vi "Omniax_MotorDrive_XYZR_LOOP_V.vi"() -> ()   [LabVIEW 2009]
uses:
  <vilib>/Utility/file.llb/Read From Spreadsheet File (DBL).vi
  <vilib>/Utility/file.llb/Read From Spreadsheet File (string).vi
  <vilib>/Instr/_visa.llb/VISA Configure Serial Port (Instr).vi
  <vilib>/Utility/file.llb/Write To Spreadsheet File (string).vi
  <vilib>/Utility/file.llb/Write To Spreadsheet File (DBL).vi
panel:
  out "NewLoop":bool
  out "LoopCheck":bool
  out "Only GO":bool
  in  "Loop Scan":bool
  out "FirstScan":bool
  out "Z Moved":bool
  out "GOBACK":bool
  out "LoopScanConfirmed":bool
  out "counter":i32
  out "OP":bool
  out "CL":bool
  out "Valve \nopend/closed":bool
  in  "OK Button":bool
  out "STATUS":string
  in  "Delete Button":bool
  in  "String":string
  in  "Add Button":bool
  in  "Set Button":bool
  in  "Preset positions":i32(ring) items=["ZERO", "Default", "CDOSE", "QMS", "test", "test2", "test3"]
  out "Presets":i32[][](array[numeric])
  out "X MINPOS":i32=-94296
  out "X MAXPOS":i32=-34296
  out "Y MINPOS":i32=-94296
  out "Y MAXPOS":i32=-34296
  out "R MAXPOS":i32=-34296
  out "R MINPOS":i32=-94296
  out "Z MINPOS":i32=-94296
  out "Z MAXPOS":i32=-34296
  in  "HARDSTOP":bool
  in  "GO":bool
  out "XYZR VEL PV Array":i32[](array[numeric])
  out "XYZ in RANGE Array":bool[](array[boolean])
  out "STEP SP Array":i32[](array[numeric])
  out "RUNHOLDArray":i32[](array[numeric])
  out "ZCONSTArray":dbl[](array[numeric])
  out "RCONSTArray":dbl[](array[numeric])
  out "XCONSTArray":dbl[](array[numeric])
  out "YCONSTArray":dbl[](array[numeric])
  out "Error Array":errorcluster[](array[cluster])
  out "COM PORT Array":refnum<visa-resource-name>[](array[refnum])
  out "Z COM PORT":refnum<visa-resource-name>="COM6"
  in  "Tab Control 3":enum32{"Status", "Reset"}(tab)
  out "Y in Range":bool
  out "Y Scan":bool
  out "Y in Motion":bool
  out "Y Backlash corr":bool
  out "X  in Range":bool
  out "X Scan":bool
  out "X  in Motion":bool
  out "X Backlash corr":bool
  out "Z in Range":bool
  out "Z Scan":bool
  out "Z in Motion":bool
  out "Z Backlash corr":bool
  out "R in Range":bool
  out "R Scan":bool
  out "R in Motion":bool
  out "R Backlash corr":bool
  out "X Ready":bool
  out "Y Ready":bool
  out "Z Ready":bool
  out "R Ready":bool
  in  "Reset Y Position mm":dbl
  out "Reset Y Motor Steps":i32
  in  "Reset X Position mm":dbl
  out "Reset X Motor Steps":i32
  in  "Reset Z Position mm":dbl
  out "Reset Z Motor Steps":i32
  in  "Reset R Position deg":dbl
  out "Reset R Motor Steps":i32
  in  "Reset":bool
  in  "Tab Control 2":enum32{"mm", "step"}(tab)
  in  "X Scan Length SP mm":dbl
  in  "X Scan Velocity SP mm/sec":dbl
  in  "Y Scan Length SP mm":dbl
  in  "Y Scan Velocity SP mm/sec":dbl
  in  "Set Scan \nParameters":bool
  in  "Z Scan Length SP mm":dbl
  in  "Z Scan Velocity SP mm/sec":dbl
  in  "R Scan Length SP deg":dbl
  in  "R Scan Velocity SP deg/sec":dbl
  in  "Z as dominating length":bool
  in  "Nr LOOPS":i32
  in  "X Scan Velocity SP steps/sec":i32=1 min=1 max=102400 step=1
  in  "X Scan Length SP steps":i32 min=-2304000 max=2304000 step=100
  out "X Scan length MV mm":dbl
  out "X Scan velocity MV mm/sec":dbl format="%#_6f"
  in  "Y Scan Velocity SP steps/sec":i32=1 min=1 max=102400 step=1
  in  "Y Scan Length SP steps":i32 min=-2560000 max=2048000 step=100
  out "Y Scan length MV mm":dbl
  out "Y Scan velocity MV mm/sec":dbl format="%#_6f"
  in  "Z Scan Velocity SP steps/sec":i32=1 min=1 max=102400 step=1
  in  "Z Scan Length SP steps":i32 min=-11520000 max=90880000 step=100
  out "Z Scan length MV mm":dbl
  out "Z Scan velocity MV mm/sec":dbl format="%#_6f"
  in  "R Scan Velocity SP steps/sec":i32=1 min=1 max=102400 step=1
  in  "R Scan Length SP steps":i32 min=-1501867 max=4642133 step=100
  out "R Scan length MV deg":dbl
  out "R Scan velocity MV deg/sec":dbl format="%#_6f"
  out "atan Y/Z":dbl
  in  "Tab Control":enum32{"mm", "step"}(tab)
  in  "X Position SP mm":dbl
  in  "X Velocity SP mm/sec":dbl
  in  "X Move Set":bool
  in  "Y Move Set":bool
  in  "Y Position SP mm":dbl
  in  "Y Velocity SP mm/sec":dbl
  in  "Z Position SP mm":dbl
  in  "Z Velocity SP mm/sec":dbl
  in  "Z Move Set":bool
  in  "R Position SP deg":dbl
  in  "R Velocity SP deg/sec":dbl
  in  "R Move Set":bool
  in  "X Velocity SP step/sec":i32 min=1 max=128000
  out "X Velocity MV mm/sec":dbl
  in  "Y Velocity SP step/sec":i32 min=1 max=128000
  out "Y Velocity MV mm/sec":dbl
  in  "Z Velocity SP step/sec":i32 min=1 max=204800
  out "Z Velocity MV mm/sec":dbl
  in  "R Velocity SP step/sec":i32 min=1 max=20000
  out "R Velocity MVdeg/sec":dbl
  in  "Y Step SP":i32=-20000 min=-2304000 max=2304000 step=500
  out "Y Position MV mm":dbl
  in  "X Step SP":i32=-20000 min=-2304000 max=2304000 step=500
  out "X Position MV mm":dbl
  in  "Z Step SP":i32=-20000 min=0 max=102400000 step=500
  out "Z Position MV mm":dbl
  in  "R Step SP":i32=-20000 min=-6144000 max=0 step=500
  out "R Position MV deg":dbl
  out "X Step PV":i32 max=2000
  out "Y Step PV":i32 max=2000
  out "Z Step PV":i32 max=2000
  out "R Step PV":i32 max=2000
  in  "Clear ZY":bool
  out "ZY Graph":cluster{dbl[], dbl[]}(graph)
  out "ZR Graph":cluster{"Y":dbl[], "Y":dbl[]}[](graph)
  out "XY Graph":cluster{"Y":dbl[], "Y":dbl[]}[](graph)
  out "X Scan Duration":dbl
  out "Y Scan Duration":dbl
  out "Z Scan Duration":dbl
  out "R Scan Duration":dbl
  out "R Backlash steps/sec":i32
  out "R Backlash":i32
  out "R Holding Current %":i32
  out "R Run Current %":i32
  out "R offset deg":dbl
  out "R deg/rev":dbl
  out "R steps/rev":u32
  out "R velocity PV step/sec":i32
  out "R COM PORT":refnum<visa-resource-name>="COM5"
  out "R Position deg PV":dbl
  out "Z Backlash steps/sec":i32
  out "Z Backlash":i32
  out "Z Holding Current %":i32
  out "Z Run Current %":i32
  out "Z offset mm":dbl
  out "Z mm/rev":dbl
  out "Z steps/rev":u32
  out "Z  velocity PV step/sec":i32
  out "Z Position mm PV":dbl
  out "X Position mm PV":dbl
  out "X velocity PV step/sec":i32
  in  "Set for Scan":bool
  out "X Backlash steps/sec":i32
  out "X Backlash":i32
  out "X Holding Current %":i32
  out "X Run Current %":i32
  out "X offset mm":dbl
  out "X mm/rev":dbl
  out "X steps/rev":u32
  out "X COM PORT":refnum<visa-resource-name>="COM5"
  out "Y Backlash steps/sec":i32
  out "Y Backlash":i32
  out "Y Holding Current %":i32
  out "Y Run Current %":i32
  in  "Scan Cancel":bool
  out "Y Position mm PV":dbl
  out "Y offset mm":dbl
  out "Y mm/rev":dbl
  out "Y steps/rev":u32
  out "Y velocity PV step/sec":i32
  in  "Scan Go":bool
  in  "Stop":bool
  out "Y COM PORT":refnum<visa-resource-name>="COM5"
  # "MX"
  # "MY"
  # "MZ"
  # "MR"
  # "Indicators"
  # "L"
  # "M"
  # "B"
  # "S"
  # "R"
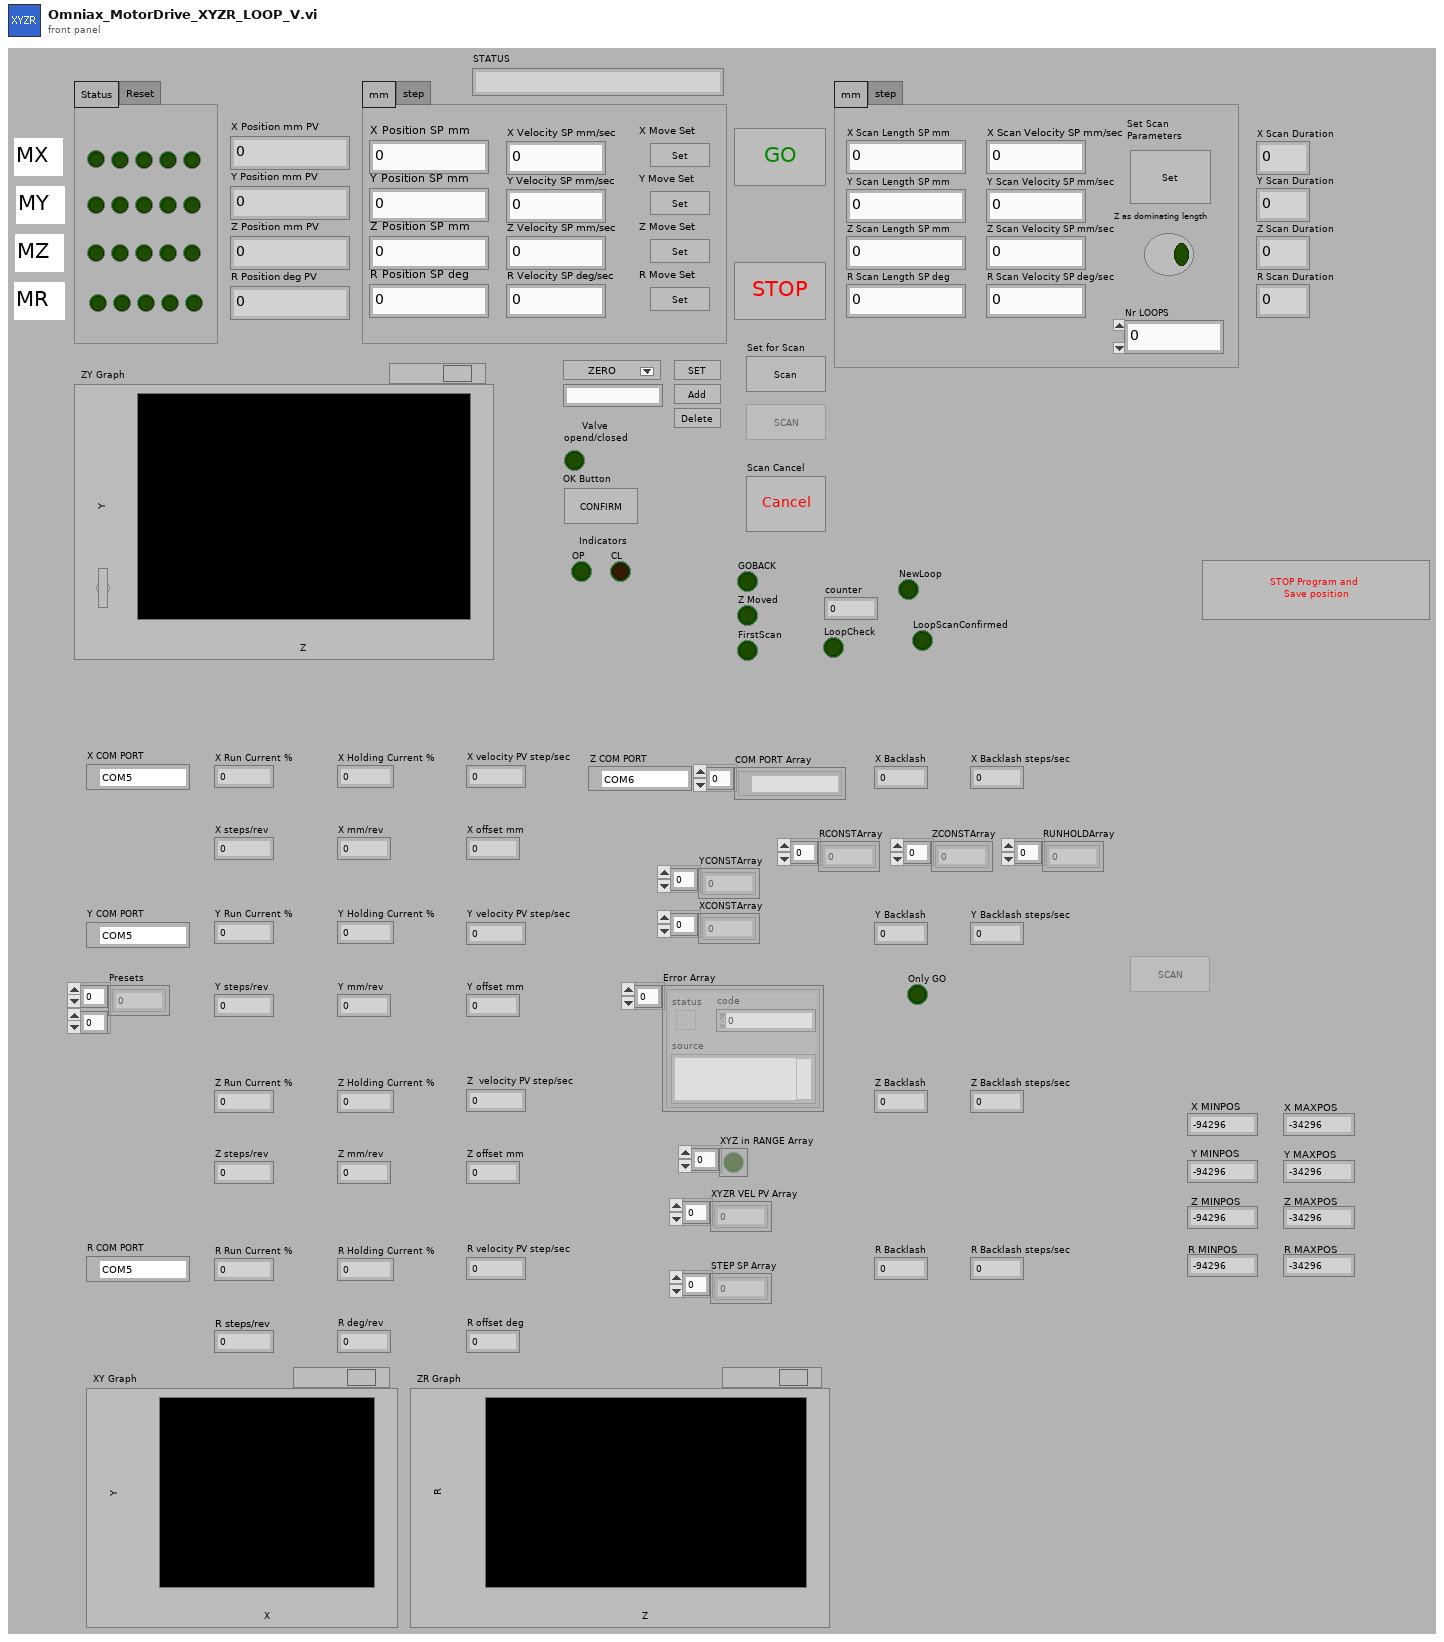
[diagram p1: front panel]
types:
  T1 = enum8{"Enabled", "Disabled", "Disabled and Grayed Out"}
  T2 = cluster{"[0]":i32, "[1]":i32, "[2]":i32, "[3]":i32, "[4]":i32, "[5]":i32, "[6]":i32, "[7]":i32, "[8]":i32}
  T3 = cluster{"XY Max Min array OUT[0]":dbl, "XY Max Min array OUT[1]":dbl, "XY Max Min array OUT[2]":dbl, "XY Max Min array OUT[3]":dbl, "XY Max Min array OUT[4]":dbl, "XY Max Min array OUT[5]":dbl, "XY Max Min array OUT[6]":dbl, "XY Max Min array OUT[7]":dbl, "XY Max Min array OUT[8]":dbl}
  T4 = cluster{"COM PORT Array OUT[0]":refnum<visa-resource-name>, "COM PORT Array OUT[1]":refnum<visa-resource-name>, "COM PORT Array OUT[2]":refnum<visa-resource-name>, "COM PORT Array OUT[3]":refnum<visa-resource-name>, "COM PORT Array OUT[4]":refnum<visa-resource-name>, "COM PORT Array OUT[5]":refnum<visa-resource-name>, "COM PORT Array OUT[6]":refnum<visa-resource-name>, "COM PORT Array OUT[7]":refnum<visa-resource-name>, "COM PORT Array OUT[8]":refnum<visa-resource-name>}
  T5 = cluster{"STEP SP Array OUT[0]":i32, "STEP SP Array OUT[1]":i32, "STEP SP Array OUT[2]":i32, "STEP SP Array OUT[3]":i32, "STEP SP Array OUT[4]":i32, "STEP SP Array OUT[5]":i32, "STEP SP Array OUT[6]":i32, "STEP SP Array OUT[7]":i32, "STEP SP Array OUT[8]":i32}
  T6 = cluster{"XYZ in RANGE Array OUT[0]":bool, "XYZ in RANGE Array OUT[1]":bool, "XYZ in RANGE Array OUT[2]":bool, "XYZ in RANGE Array OUT[3]":bool, "XYZ in RANGE Array OUT[4]":bool, "XYZ in RANGE Array OUT[5]":bool, "XYZ in RANGE Array OUT[6]":bool, "XYZ in RANGE Array OUT[7]":bool, "XYZ in RANGE Array OUT[8]":bool}
  T7 = cluster{"XYZR VEL PV Array OUT[0]":i32, "XYZR VEL PV Array OUT[1]":i32, "XYZR VEL PV Array OUT[2]":i32, "XYZR VEL PV Array OUT[3]":i32, "XYZR VEL PV Array OUT[4]":i32, "XYZR VEL PV Array OUT[5]":i32, "XYZR VEL PV Array OUT[6]":i32, "XYZR VEL PV Array OUT[7]":i32, "XYZR VEL PV Array OUT[8]":i32}
  T8 = cluster{"XYZR MAX MIN POS[0]":i32, "XYZR MAX MIN POS[1]":i32, "XYZR MAX MIN POS[2]":i32, "XYZR MAX MIN POS[3]":i32, "XYZR MAX MIN POS[4]":i32, "XYZR MAX MIN POS[5]":i32, "XYZR MAX MIN POS[6]":i32, "XYZR MAX MIN POS[7]":i32, "XYZR MAX MIN POS[8]":i32}
  T9 = cluster{"Error Array OUT[0]":errorcluster, "Error Array OUT[1]":errorcluster, "Error Array OUT[2]":errorcluster, "Error Array OUT[3]":errorcluster, "Error Array OUT[4]":errorcluster, "Error Array OUT[5]":errorcluster, "Error Array OUT[6]":errorcluster, "Error Array OUT[7]":errorcluster, "Error Array OUT[8]":errorcluster}
  T10 = enum16{"Stop", "Reset", "Run Current", "Holding Current", "Accel Rate", "Decel Rate", "Move to Relative Position", "Move to Absolute Position", "Echo Mode", "Print Parameter", "Send String", "Microstep Resolution", "Set Current Position", "Max Velocity"}
  T11 = cluster{"Presets[0]":i32, "Presets[1]":i32, "Presets[2]":i32, "Presets[3]":i32, "Presets[4]":i32, "Presets[5]":i32, "Presets[6]":i32, "Presets[7]":i32, "Presets[8]":i32}
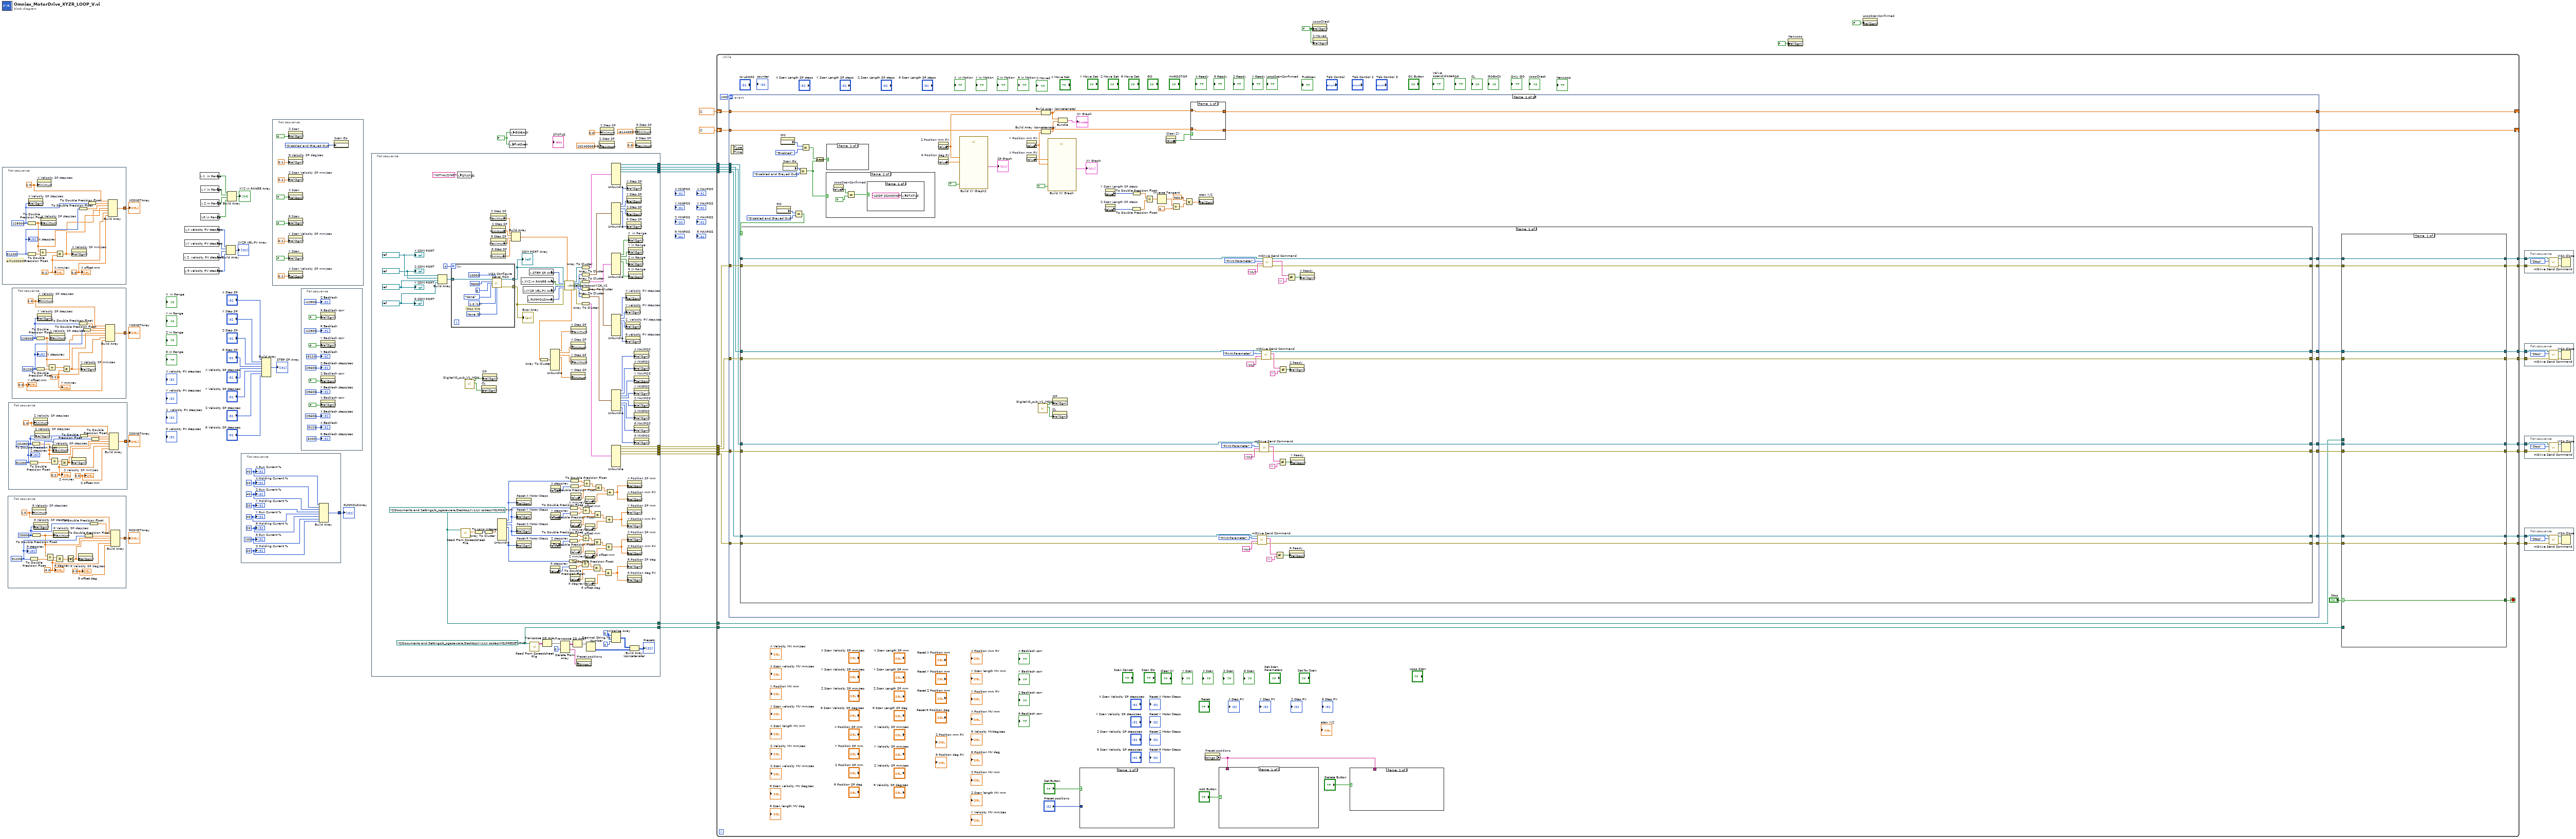
[diagram p0: block diagram]
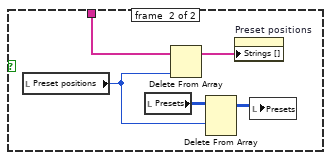
[diagram p2: hidden frame]
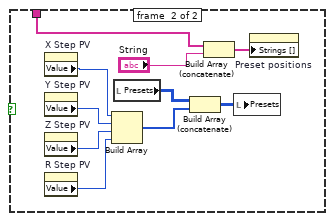
[diagram p3: hidden frame]
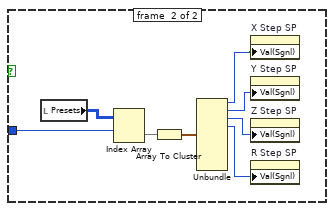
[diagram p4: hidden frame]
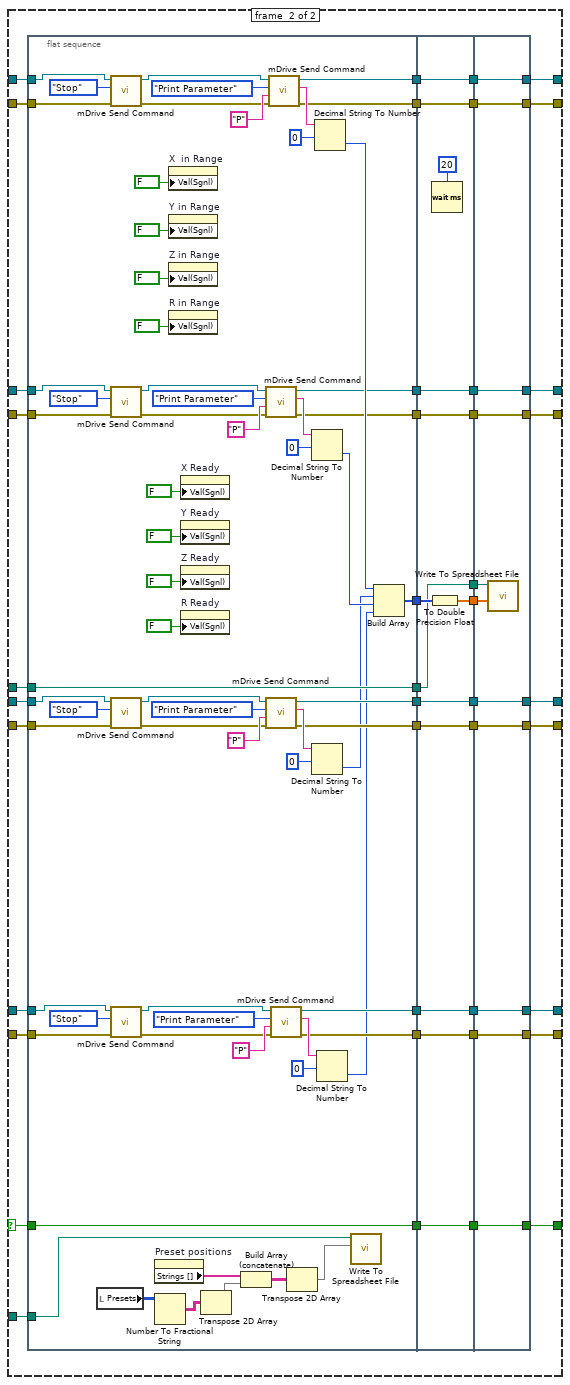
[diagram p5: hidden frame]
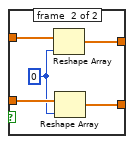
[diagram p6: hidden frame]
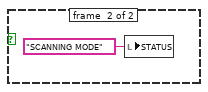
[diagram p7: hidden frame]
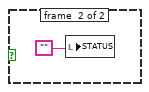
[diagram p9: hidden frame]
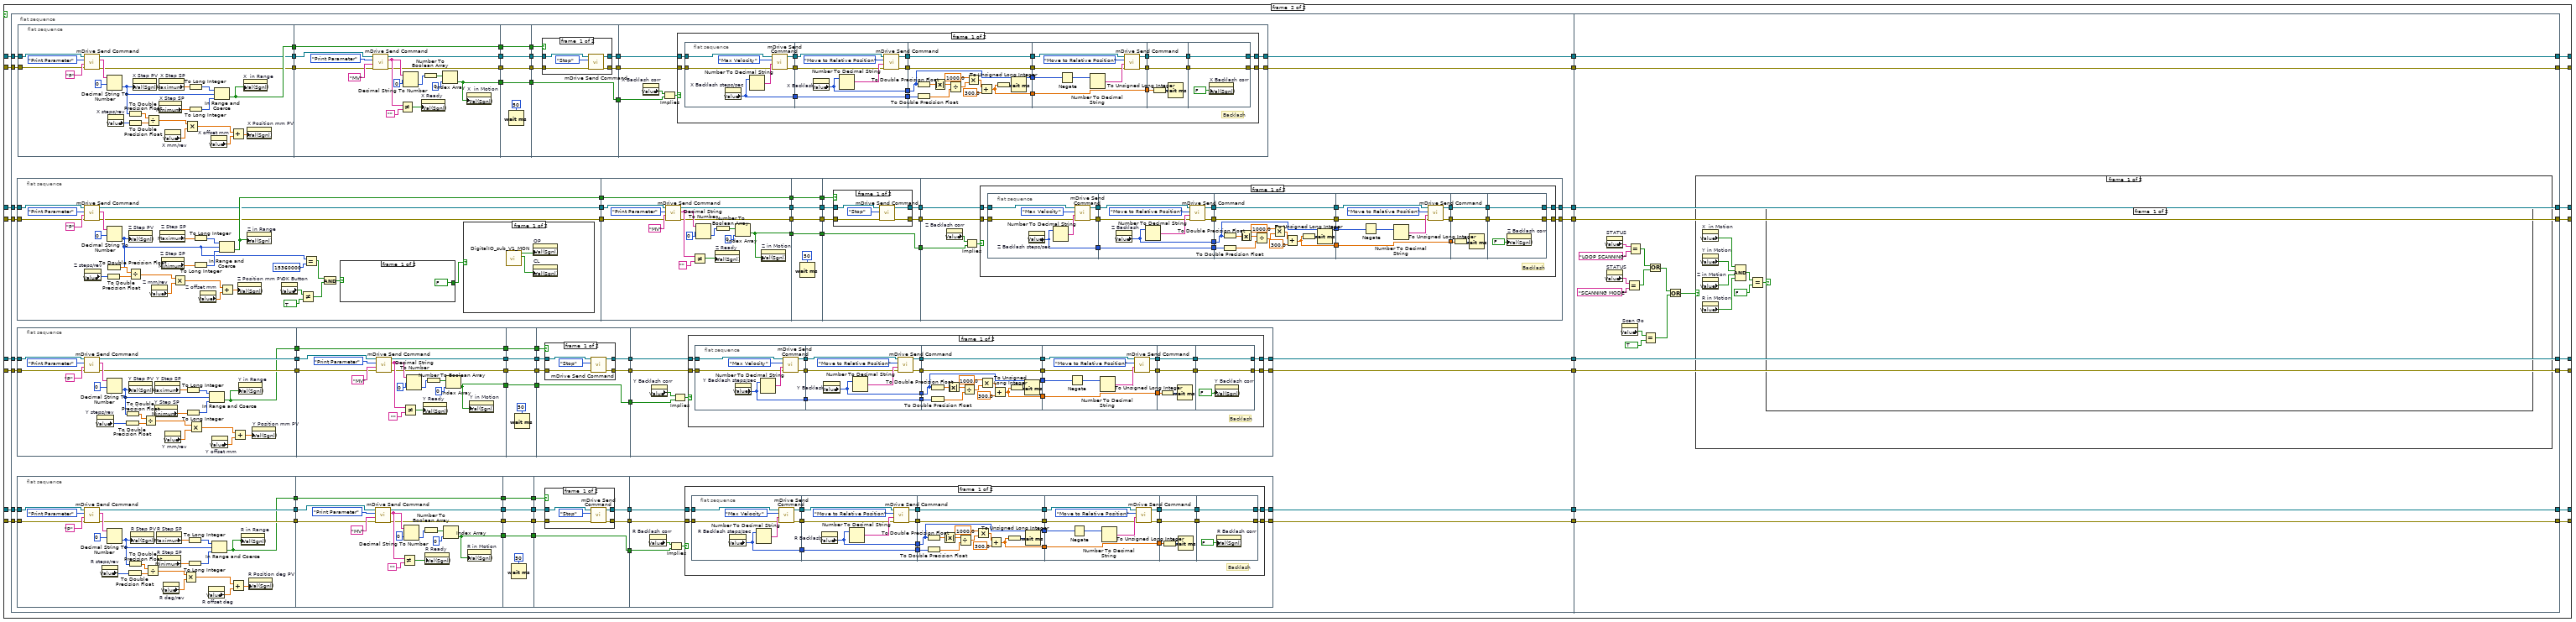
[diagram p10: hidden frame]
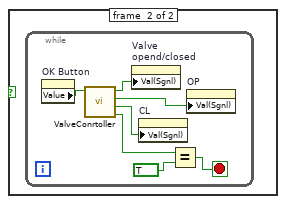
[diagram p15: hidden frame]
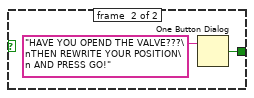
[diagram p16: hidden frame]
diagram:
  w3 = FALSE ("Value (Signaling)")
  w4 = FALSE
  n1 = flat-sequence {
    tunnel: [w56] -> w39
    frame #0 {
      w54 = 0.2 ("MM/rev")
      w59 = u32 51200 ("step/rev")
      w61 = 128000 ("Value (Signaling)")
      w62 = 1.0 ("Data Entry Limits:Minimum")
      w55 = 0.0 ("offset")
      # "a=1000000"
      n2 = To Double Precision Float(number=w61) -> (double precision float=w53:dbl)
      n3 = To Double Precision Float(number=w59) -> (double precision float=w64:dbl)
      n4 = property on="X Velocity SP step/sec" class="DigNum (strict)"("Val(Sgnl)"=w61) -> ()  [unwired: 2 in, 2 out]
      n5 = property on="X Velocity SP step/sec" class="DigNum (strict)"("Minimum"=w62) -> ()  [unwired: 2 in, 2 out]
      n6 = Divide(x=w53, y=w64) -> (x/y=w63:dbl)
      n7 = property on="X Velocity SP step/sec" class="DigNum (strict)"("Maximum"=w53) -> ()  [unwired: 2 in, 2 out]
      n8 = Multiply(x=w63, y=w54) -> (x*y=w57:dbl)
      n9 = property on="X Velocity SP mm/sec" class="DigNum (strict)"("Val(Sgnl)"=w57) -> ()  [unwired: 2 in, 2 out]
      n10 = To Double Precision Float(number=w59) -> (double precision float=w58:dbl)
      n11 = To Double Precision Float(number=w61) -> (double precision float=w60:dbl)
      n12 = Build Array(w62, w60, w58, w57, w53, w54, w55) -> (w56:dbl[])
      "X offset mm" <- w55
      "X steps/rev" <- w59
      "X mm/rev" <- w54
    }
  }
  n13 = flat-sequence {
    tunnel: [w65] -> w38
    frame #0 {
      w74 = 1.0 ("Data Entry Limits:Minimum")
      w68 = 0.0 ("R offset deg")
      w69 = -3.0 ("R deg/rev")
      w72 = u32 51200 ("step/rev")
      w73 = 20000 ("Value (Signaling)")
      n14 = To Double Precision Float(number=w72) -> (double precision float=w75:dbl)
      n15 = To Double Precision Float(number=w73) -> (double precision float=w71:dbl)
      n16 = property on="R Velocity SP step/sec" class="DigNum (strict)"("Minimum"=w74) -> ()  [unwired: 2 in, 2 out]
      n17 = property on="R Velocity SP step/sec" class="DigNum (strict)"("Val(Sgnl)"=w73) -> ()  [unwired: 2 in, 2 out]
      n18 = Divide(x=w71, y=w75) -> (x/y=w77:dbl)
      n19 = property on="R Velocity SP step/sec" class="DigNum (strict)"("Maximum"=w71) -> ()  [unwired: 2 in, 2 out]
      n20 = Multiply(x=w77, y=w69) -> (x*y=w76:dbl)
      n21 = Absolute Value(x=w76) -> (abs(x)=w70:dbl)
      n22 = property on="R Velocity SP deg/sec" class="DigNum (strict)"("Val(Sgnl)"=w70) -> ()  [unwired: 2 in, 2 out]
      n23 = To Double Precision Float(number=w72) -> (double precision float=w66:dbl)
      n24 = To Double Precision Float(number=w73) -> (double precision float=w67:dbl)
      n25 = Build Array(w74, w67, w66, w71, w70, w69, w68) -> (w65:dbl[])
      "R offset deg" <- w68
      "R deg/rev" <- w69
      "R steps/rev" <- w72
    }
  }
  n26 = flat-sequence {
    tunnel: [w78] -> w37
    frame #0 {
      w80 = 0.2 ("Z mm/rev")
      w84 = u32 51200 ("step/rev")
      w86 = 204800 ("Value (Signaling)")
      w87 = 1.0 ("Data Entry Limits:Minimum")
      w79 = 0.0 ("Z offset mm")
      n27 = To Double Precision Float(number=w84) -> (double precision float=w89:dbl)
      n28 = To Double Precision Float(number=w86) -> (double precision float=w82:dbl)
      n29 = property on="Z Velocity SP step/sec" class="DigNum (strict)"("Minimum"=w87) -> ()  [unwired: 2 in, 2 out]
      n30 = property on="Z Velocity SP step/sec" class="DigNum (strict)"("Val(Sgnl)"=w86) -> ()  [unwired: 2 in, 2 out]
      n31 = Divide(x=w82, y=w89) -> (x/y=w88:dbl)
      n32 = property on="Z Velocity SP step/sec" class="DigNum (strict)"("Maximum"=w82) -> ()  [unwired: 2 in, 2 out]
      n33 = Multiply(x=w88, y=w80) -> (x*y=w81:dbl)
      n34 = property on="Z Velocity SP mm/sec" class="DigNum (strict)"("Val(Sgnl)"=w81) -> ()  [unwired: 2 in, 2 out]
      n35 = To Double Precision Float(number=w86) -> (double precision float=w85:dbl)
      n36 = To Double Precision Float(number=w84) -> (double precision float=w83:dbl)
      n37 = Build Array(w87, w85, w83, w82, w81, w80, w79) -> (w78:dbl[])
      "Z offset mm" <- w79
      "Z mm/rev" <- w80
      "Z steps/rev" <- w84
    }
  }
  n38 = flat-sequence {
    tunnel: [w93] -> w40
    frame #0 {
      w91 = 0.2 ("MM/rev")
      w96 = u32 51200 ("step/rev")
      w98 = 128000 ("Value (Signaling)")
      w99 = 1.0 ("Data Entry Limits:Minimum")
      w92 = 0.0 ("offset")
      n39 = To Double Precision Float(number=w98) -> (double precision float=w90:dbl)
      n40 = To Double Precision Float(number=w96) -> (double precision float=w101:dbl)
      n41 = property on="Y Velocity SP step/sec" class="DigNum (strict)"("Val(Sgnl)"=w98) -> ()  [unwired: 2 in, 2 out]
      n42 = property on="Y Velocity SP step/sec" class="DigNum (strict)"("Minimum"=w99) -> ()  [unwired: 2 in, 2 out]
      n43 = Divide(x=w90, y=w101) -> (x/y=w100:dbl)
      n44 = property on="Y Velocity SP step/sec" class="DigNum (strict)"("Maximum"=w90) -> ()  [unwired: 2 in, 2 out]
      n45 = Multiply(x=w100, y=w91) -> (x*y=w94:dbl)
      n46 = To Double Precision Float(number=w98) -> (double precision float=w97:dbl)
      n47 = property on="Y Velocity SP mm/sec" class="DigNum (strict)"("Val(Sgnl)"=w94) -> ()  [unwired: 2 in, 2 out]
      n48 = To Double Precision Float(number=w96) -> (double precision float=w95:dbl)
      n49 = Build Array(w99, w97, w95, w94, w90, w91, w92) -> (w93:dbl[])
      "Y offset mm" <- w92
      "Y steps/rev" <- w96
      "Y mm/rev" <- w91
    }
  }
  n50 = local read "Z  velocity PV step/sec"() -> (w20:i32)
  n51 = local read "R velocity PV step/sec"() -> (w22:i32)
  n52 = local read "X velocity PV step/sec"() -> (w23:i32)
  n53 = local read "Y velocity PV step/sec"() -> (w21:i32)
  n54 = local read "X  in Range"() -> (w27:bool)
  n55 = local read "R in Range"() -> (w24:bool)
  n56 = local read "Y in Range"() -> (w26:bool)
  n57 = local read "Z in Range"() -> (w25:bool)
  n58 = Build Array(w23, w21, w20, w22) -> (→"XYZR VEL PV Array":i32[])
  n59 = Build Array(w27, w26, w25, w24) -> (→"XYZ in RANGE Array":bool[])
  n60 = flat-sequence {
    tunnel: [w102] -> w36
    frame #0 {
      w105 = 20 ("R Holding Current %")
      w104 = 100 ("R Run Current %")
      w107 = 20 ("Holding Current %")
      w106 = 40 ("Run Current %")
      w109 = 20 ("Holding Current %")
      w110 = 40 ("Run Current %")
      w108 = 40 ("Z Run Current %")
      w103 = 20 ("Z Holding Current %")
      n61 = Build Array(w110, w109, w108, w107, w106, w105, w104, w103) -> (w102:i32[])
      "Z Holding Current %" <- w103
      "Z Run Current %" <- w108
      "X Run Current %" <- w110
      "X Holding Current %" <- w109
      "Y Run Current %" <- w106
      "Y Holding Current %" <- w107
      "R Holding Current %" <- w105
      "R Run Current %" <- w104
    }
  }
  n62 = Build Array("X Step SP", "Y Step SP", "Z Step SP", "R Step SP", "X Velocity SP step/sec", "Y Velocity SP step/sec", "Z Velocity SP step/sec", "R Velocity SP step/sec") -> (→"STEP SP Array":i32[])
  n63 = flat-sequence {
    frame #0 {
      n64 = property on="Z Scan" class="Bool (strict)"("Val(Sgnl)"=FALSE ("Value (Signaling)")) -> ()  [unwired: 2 in, 2 out]
      n65 = property on="R Velocity SP deg/sec" class="DigNum (strict)"("Val(Sgnl)"=0.1 ("Value (Signaling)")) -> ()  [unwired: 2 in, 2 out]
      n66 = property on="Z Scan Velocity SP mm/sec" class="DigNum (strict)"("Val(Sgnl)"=0.1 ("Value (Signaling)")) -> ()  [unwired: 2 in, 2 out]
      n67 = property on="X Scan" class="Bool (strict)"("Val(Sgnl)"=FALSE ("Value (Signaling)")) -> ()  [unwired: 2 in, 2 out]
      n68 = property on="R Scan" class="Bool (strict)"("Val(Sgnl)"=FALSE ("Value (Signaling)")) -> ()  [unwired: 2 in, 2 out]
      n69 = property on="Y Scan Velocity SP mm/sec" class="DigNum (strict)"("Val(Sgnl)"=0.1 ("Value (Signaling)")) -> ()  [unwired: 2 in, 2 out]
      n70 = property on="Y Scan" class="Bool (strict)"("Val(Sgnl)"=FALSE ("Value (Signaling)")) -> ()  [unwired: 2 in, 2 out]
      n71 = property on="X Scan Velocity SP mm/sec" class="DigNum (strict)"("Val(Sgnl)"=0.1 ("Value (Signaling)")) -> ()  [unwired: 2 in, 2 out]
      n72 = property on="Scan Go" class="Bool (strict)"("DisabledEnum"=T1."Disabled and Grayed Out" ("Disabled")) -> ()  [unwired: 2 in, 2 out]
    }
  }
  n73 = flat-sequence {
    frame #0 {
      n74 = property on="R Backlash corr" class="Bool (strict)"("Val(Sgnl)"=FALSE ("Value (Signaling)")) -> ()  [unwired: 2 in, 2 out]
      n75 = property on="Y Backlash corr" class="Bool (strict)"("Val(Sgnl)"=FALSE ("Value (Signaling)")) -> ()  [unwired: 2 in, 2 out]
      n76 = property on="Z Backlash corr" class="Bool (strict)"("Val(Sgnl)"=FALSE ("Value (Signaling)")) -> ()  [unwired: 2 in, 2 out]
      n77 = property on="X Backlash corr" class="Bool (strict)"("Val(Sgnl)"=FALSE ("Value (Signaling)")) -> ()  [unwired: 2 in, 2 out]
      "Z Backlash steps/sec" <- 25600 ("Z Backlash steps/sec")
      "Z Backlash" <- -12800 ("Z Backlash")
      "X Backlash steps/sec" <- 25600 ("Value (Signaling)")
      "X Backlash" <- 5120 ("Backlash2")
      "Y Backlash" <- -5120 ("Backlash2")
      "Y Backlash steps/sec" <- 25600 ("Value (Signaling)")
      "R Backlash steps/sec" <- 6400 ("R Backlash steps/sec")
      "R Backlash" <- -12800 ("R Backlash")
    }
  }
  n78 = flat-sequence {
    tunnel: [w226] -> w16
    tunnel: [w225] -> w15
    tunnel: [w224] -> w14
    tunnel: [w223] -> w13
    tunnel: [w222] -> w12
    tunnel: [w221] -> w11
    tunnel: [w220] -> w10
    tunnel: [w219] -> w9
    tunnel: [w216] -> w8
    tunnel: [w186] -> w7
    frame #0 {
      w186 = path "C:/Documents and Settings/b_ogasawara/Desktop/lv1/LV codes/IMS/PRESET.TXT"
      w184 = 0 ("element")
      w216 = path "C:/Documents and Settings/b_ogasawara/Desktop/lv1/LV codes/IMS/POS.TXT"
      w246 = refnum<visa-resource-name> "COM7" ("COM PORT")
      w247 = refnum<visa-resource-name> "COM5" ("COM PORT")
      w248 = refnum<visa-resource-name> "COM6" ("VISA resource name")
      w249 = refnum<visa-resource-name> "COM4" ("COM PORT")
      n79 = Build Array(w249, w248, w247, w246) -> (w244:refnum<visa-resource-name>[])
      n80 = for {
        N: 4 -> [_]
        tunnel: w244 -> [w252] mode=indexing
        tunnel: [w251] -> w242 mode=indexing
        tunnel: [w250] -> w243 mode=indexing
        w254 = u16 0 items=["None", "XON/XOFF", "RTS/CTS", "XON/XOFF & RTS/CTS", "DTR/DSR", "XON/XOFF & DTR/DSR"] ("flow control (0:none)")
        w255 = u16 10 items=["1.0"=10, "1.5"=15, "2.0"=20] ("stop bits (10: 1 bit)")
        # "Stop bits"
        n81 = call-poly "VISA Configure Serial Port"("VISA resource name"=w252, "timeout (10sec)"=u32 10000, "baud rate (9600)"=u32 9600, "data bits (8)"=u16 8, "parity (0:none)"=enum16{"None", "Odd", "Even", "Mark", "Space"}."None", "stop bits (10: 1 bit)"=w255, "flow control (0:none)"=w254) -> ("VISA resource name out"=w251:refnum<visa-resource-name>, "error out"=w250:errorcluster)  [unwired: 7 in]
      }
      "COM PORT Array" <- w242
      "Error Array" <- w243
      n82 = local write "STATUS"("INITIALIZING" ("STATUS")) -> ()
      n83 = call-poly <vilib>:"Read From Spreadsheet File.vi"("file path (dialog if empty)"=w216) -> ("first row"=w217:dbl[])  [unwired: 6 in, 4 out]
      n84 = call "DigitalIO_sub_V1_MON.vi"() -> ("CL"=w143:bool, "OP"=w144:bool)  [unwired: 8 in]
      n85 = To Long Integer(number=w217) -> (32bit integer=w183:i32[])
      n86 = property on="CL" class="Bool (strict)"("Val(Sgnl)"=w143) -> ()  [unwired: 2 in, 2 out]
      n87 = property on="OP" class="Bool (strict)"("Val(Sgnl)"=w144) -> ()  [unwired: 2 in, 2 out]
      n88 = Array To Cluster(array=w183) -> (cluster=w182:T2)
      n89 = property on="Z Step SP" class="DigNum (strict)"() -> ("Maximum"=w141:dbl)  [unwired: 2 in, 2 out]
      n90 = property on="R Step SP" class="DigNum (strict)"() -> ("Maximum"=w139:dbl)  [unwired: 2 in, 2 out]
      n91 = property on="R Step SP" class="DigNum (strict)"() -> ("Minimum"=w140:dbl)  [unwired: 2 in, 2 out]
      n92 = property on="Z Step SP" class="DigNum (strict)"() -> ("Minimum"=w142:dbl)  [unwired: 2 in, 2 out]
      n93 = Unbundle(w182) -> ("[0]"=w158:i32, "[1]"=w159:i32, "[2]"=w160:i32, "[3]"=w161:i32)  [unwired: 5 out]
      n94 = Build Array(w141, w142, w139, w140) -> (w138:dbl[])
      n95 = property on="Reset X Motor Steps" class="DigNum (strict)"("Val(Sgnl)"=w158) -> ()  [unwired: 2 in, 2 out]
      n96 = property on="Reset Y Motor Steps" class="DigNum (strict)"("Val(Sgnl)"=w159) -> ()  [unwired: 2 in, 2 out]
      n97 = property on="Reset Z Motor Steps" class="DigNum (strict)"("Val(Sgnl)"=w160) -> ()  [unwired: 2 in, 2 out]
      n98 = property on="Reset R Motor Steps" class="DigNum (strict)"("Val(Sgnl)"=w161) -> ()  [unwired: 2 in, 2 out]
      n99 = local read "XYZ in RANGE Array"() -> (w238:bool[])
      n100 = local read "XYZR VEL PV Array"() -> (w237:i32[])
      n101 = local read "RUNHOLDArray"() -> (w236:i32[])
      n102 = local read "STEP SP Array"() -> (w239:i32[])
      n103 = call-poly <vilib>:"Read From Spreadsheet File.vi"("file path (dialog if empty)"=w186) -> ("all rows"=w191:string[][])  [unwired: 6 in, 4 out]
      n104 = Transpose 2D Array(2D array=w191) -> (transposed array=w190:string[][])
      n105 = property on="R steps/rev" class="DigNum (strict)"() -> ("Value"=w154:u32)  [unwired: 2 in, 2 out]
      n106 = property on="X steps/rev" class="DigNum (strict)"() -> ("Value"=w157:u32)  [unwired: 2 in, 2 out]
      n107 = property on="Y steps/rev" class="DigNum (strict)"() -> ("Value"=w156:u32)  [unwired: 2 in, 2 out]
      n108 = property on="Z steps/rev" class="DigNum (strict)"() -> ("Value"=w155:u32)  [unwired: 2 in, 2 out]
      n109 = Delete From Array(array=w190, index (row)=0) -> (deleted portion=w185:string[], array with subset deleted=w188:string[][])  [unwired: 2 in]
      n110 = call "InitializeMotorsXYZR_V2.vi"("COM PORT Array IN"=w242, "STEP SP Array IN"=w239, "XYZ in RANGE Array IN"=w238, "XYZR VEL PV Array IN"=w237, "RUNHOLDArray IN"=w236, "Error Array IN"=w243, "ZR Max Min array"=w138) -> ("XY Max Min array OUT"=w137:dbl[], "COM PORT Array OUT"=w241:refnum<visa-resource-name>[], "STEP SP Array OUT"=w235:i32[], "XYZ in RANGE Array OUT"=w234:bool[], "XYZR VEL PV Array OUT"=w233:i32[], "XYZR MAX MIN POS"=w218:i32[], "Error Array OUT"=w240:errorcluster[])  [unwired: 6 in]
      n111 = Array To Cluster(array=w137) -> (cluster=w136:T3)
      n112 = Unbundle(w136) -> ("XY Max Min array OUT[0]"=w135:dbl, "XY Max Min array OUT[1]"=w133:dbl, "XY Max Min array OUT[2]"=w132:dbl, "XY Max Min array OUT[3]"=w134:dbl)  [unwired: 5 out]
      n113 = To Double Precision Float(number=w161) -> (double precision float=w167:dbl)
      n114 = To Double Precision Float(number=w154) -> (double precision float=w166:dbl)
      n115 = To Double Precision Float(number=w160) -> (double precision float=w171:dbl)
      n116 = To Double Precision Float(number=w155) -> (double precision float=w170:dbl)
      n117 = To Double Precision Float(number=w159) -> (double precision float=w175:dbl)
      n118 = To Double Precision Float(number=w156) -> (double precision float=w174:dbl)
      n119 = To Double Precision Float(number=w158) -> (double precision float=w179:dbl)
      n120 = To Double Precision Float(number=w157) -> (double precision float=w178:dbl)
      n121 = property on="R deg/rev" class="DigNum (strict)"() -> ("Value"=w150:dbl)  [unwired: 2 in, 2 out]
      n122 = property on="X Step SP" class="DigNum (strict)"("Maximum"=w135) -> ()  [unwired: 2 in, 2 out]
      n123 = property on="X Step SP" class="DigNum (strict)"("Minimum"=w133) -> ()  [unwired: 2 in, 2 out]
      n124 = property on="Y Step SP" class="DigNum (strict)"("Maximum"=w132) -> ()  [unwired: 2 in, 2 out]
      n125 = property on="Y Step SP" class="DigNum (strict)"("Minimum"=w134) -> ()  [unwired: 2 in, 2 out]
      n126 = property on="X mm/rev" class="DigNum (strict)"() -> ("Value"=w151:dbl)  [unwired: 2 in, 2 out]
      n127 = property on="Y mm/rev" class="DigNum (strict)"() -> ("Value"=w152:dbl)  [unwired: 2 in, 2 out]
      n128 = property on="Z mm/rev" class="DigNum (strict)"() -> ("Value"=w153:dbl)  [unwired: 2 in, 2 out]
      n129 = Transpose 2D Array(2D array=w188) -> (transposed array=w187:string[][])
      n130 = property on="Preset positions" class="Ring (strict)"("Strings []"=w185) -> ()  [unwired: 2 in, 2 out]
      n131 = Divide(x=w167, y=w166) -> (x/y=w169:dbl)
      n132 = Array To Cluster(array=w241) -> (cluster=w232:T4)
      n133 = Array To Cluster(array=w235) -> (cluster=w230:T5)
      n134 = Array To Cluster(array=w234) -> (cluster=w229:T6)
      n135 = Array To Cluster(array=w233) -> (cluster=w228:T7)
      n136 = Array To Cluster(array=w218) -> (cluster=w227:T8)
      n137 = Array To Cluster(array=w240) -> (cluster=w231:T9)
      n138 = Divide(x=w171, y=w170) -> (x/y=w173:dbl)
      n139 = Divide(x=w175, y=w174) -> (x/y=w177:dbl)
      n140 = Divide(x=w179, y=w178) -> (x/y=w181:dbl)
      n141 = property on="X offset mm" class="DigNum (strict)"() -> ("Value"=w146:dbl)  [unwired: 2 in, 2 out]
      n142 = property on="Y offset mm" class="DigNum (strict)"() -> ("Value"=w147:dbl)  [unwired: 2 in, 2 out]
      n143 = property on="Z offset mm" class="DigNum (strict)"() -> ("Value"=w148:dbl)  [unwired: 2 in, 2 out]
      n144 = property on="R offset deg" class="DigNum (strict)"() -> ("Value"=w149:dbl)  [unwired: 2 in, 2 out]
      n145 = Decimal String To Number(string=w187) -> (number=w189:i32[][])  [unwired: 2 in, 1 out]
      n146 = Multiply(x=w169, y=w150) -> (x*y=w168:dbl)
      n147 = Multiply(x=w173, y=w153) -> (x*y=w172:dbl)
      n148 = Multiply(x=w177, y=w152) -> (x*y=w176:dbl)
      n149 = Multiply(x=w181, y=w151) -> (x*y=w180:dbl)
      n150 = Add(x=w168, y=w149) -> (x+y=w165:dbl)
      n151 = Add(x=w172, y=w148) -> (x+y=w164:dbl)
      n152 = Add(x=w176, y=w147) -> (x+y=w163:dbl)
      n153 = Add(x=w180, y=w146) -> (x+y=w162:dbl)
      n154 = Unbundle(w232) -> ("COM PORT Array OUT[0]"=w226:refnum<visa-resource-name>, "COM PORT Array OUT[1]"=w225:refnum<visa-resource-name>, "COM PORT Array OUT[2]"=w224:refnum<visa-resource-name>, "COM PORT Array OUT[3]"=w223:refnum<visa-resource-name>)  [unwired: 5 out]
      n155 = Unbundle(w230) -> ("STEP SP Array OUT[0]"=w200:i32, "STEP SP Array OUT[1]"=w201:i32, "STEP SP Array OUT[2]"=w202:i32, "STEP SP Array OUT[3]"=w203:i32)  [unwired: 5 out]
      n156 = Unbundle(w229) -> ("XYZ in RANGE Array OUT[0]"=w215:bool, "XYZ in RANGE Array OUT[1]"=w214:bool, "XYZ in RANGE Array OUT[2]"=w213:bool, "XYZ in RANGE Array OUT[3]"=w212:bool)  [unwired: 5 out]
      n157 = Unbundle(w228) -> ("XYZR VEL PV Array OUT[0]"=w199:i32, "XYZR VEL PV Array OUT[1]"=w198:i32, "XYZR VEL PV Array OUT[2]"=w197:i32, "XYZR VEL PV Array OUT[3]"=w196:i32)  [unwired: 5 out]
      n158 = Unbundle(w227) -> ("XYZR MAX MIN POS[0]"=w211:i32, "XYZR MAX MIN POS[1]"=w210:i32, "XYZR MAX MIN POS[2]"=w209:i32, "XYZR MAX MIN POS[3]"=w208:i32, "XYZR MAX MIN POS[4]"=w207:i32, "XYZR MAX MIN POS[5]"=w206:i32, "XYZR MAX MIN POS[6]"=w205:i32, "XYZR MAX MIN POS[7]"=w204:i32)  [unwired: 1 out]
      n159 = Unbundle(w231) -> ("Error Array OUT[0]"=w222:errorcluster, "Error Array OUT[1]"=w221:errorcluster, "Error Array OUT[2]"=w220:errorcluster, "Error Array OUT[3]"=w219:errorcluster)  [unwired: 5 out]
      n160 = Initialize Array(w184, w184, 4 ("dimension size")) -> (w194:i32[][])
      n161 = property on="X velocity PV step/sec" class="DigNum (strict)"("Val(Sgnl)"=w199) -> ()  [unwired: 2 in, 2 out]
      n162 = property on="Y velocity PV step/sec" class="DigNum (strict)"("Val(Sgnl)"=w198) -> ()  [unwired: 2 in, 2 out]
      n163 = property on="Z  velocity PV step/sec" class="DigNum (strict)"("Val(Sgnl)"=w197) -> ()  [unwired: 2 in, 2 out]
      n164 = property on="R velocity PV step/sec" class="DigNum (strict)"("Val(Sgnl)"=w196) -> ()  [unwired: 2 in, 2 out]
      n165 = property on="X Step SP" class="DigNum (strict)"("Val(Sgnl)"=w200) -> ()  [unwired: 2 in, 2 out]
      n166 = property on="Y Step SP" class="DigNum (strict)"("Val(Sgnl)"=w201) -> ()  [unwired: 2 in, 2 out]
      n167 = property on="Z Step SP" class="DigNum (strict)"("Val(Sgnl)"=w202) -> ()  [unwired: 2 in, 2 out]
      n168 = property on="R Step SP" class="DigNum (strict)"("Val(Sgnl)"=w203) -> ()  [unwired: 2 in, 2 out]
      n169 = property on="X Position SP mm" class="DigNum (strict)"("Val(Sgnl)"=w162) -> ()  [unwired: 2 in, 2 out]
      n170 = property on="X Position mm PV" class="DigNum (strict)"("Val(Sgnl)"=w162) -> ()  [unwired: 2 in, 2 out]
      n171 = property on="Y Position SP mm" class="DigNum (strict)"("Val(Sgnl)"=w163) -> ()  [unwired: 2 in, 2 out]
      n172 = property on="Y Position mm PV" class="DigNum (strict)"("Val(Sgnl)"=w163) -> ()  [unwired: 2 in, 2 out]
      n173 = property on="Z Position SP mm" class="DigNum (strict)"("Val(Sgnl)"=w164) -> ()  [unwired: 2 in, 2 out]
      n174 = property on="Z Position mm PV" class="DigNum (strict)"("Val(Sgnl)"=w164) -> ()  [unwired: 2 in, 2 out]
      n175 = property on="R Position SP deg" class="DigNum (strict)"("Val(Sgnl)"=w165) -> ()  [unwired: 2 in, 2 out]
      n176 = property on="R Position deg PV" class="DigNum (strict)"("Val(Sgnl)"=w165) -> ()  [unwired: 2 in, 2 out]
      n177 = property on="X  in Range" class="Bool (strict)"("Val(Sgnl)"=w215) -> ()  [unwired: 2 in, 2 out]
      n178 = property on="Y in Range" class="Bool (strict)"("Val(Sgnl)"=w214) -> ()  [unwired: 2 in, 2 out]
      n179 = property on="Z in Range" class="Bool (strict)"("Val(Sgnl)"=w213) -> ()  [unwired: 2 in, 2 out]
      n180 = property on="R in Range" class="Bool (strict)"("Val(Sgnl)"=w212) -> ()  [unwired: 2 in, 2 out]
      n181 = Build Array (concatenate)(w194, w189) -> (→"Presets":i32[][])
      n182 = property on="X MAXPOS" class="DigNum (strict)"("Val(Sgnl)"=w211) -> ()  [unwired: 2 in, 2 out]
      n183 = property on="X MINPOS" class="DigNum (strict)"("Val(Sgnl)"=w210) -> ()  [unwired: 2 in, 2 out]
      n184 = property on="Y MAXPOS" class="DigNum (strict)"("Val(Sgnl)"=w209) -> ()  [unwired: 2 in, 2 out]
      n185 = property on="Y MINPOS" class="DigNum (strict)"("Val(Sgnl)"=w208) -> ()  [unwired: 2 in, 2 out]
      n186 = property on="Z MAXPOS" class="DigNum (strict)"("Val(Sgnl)"=w207) -> ()  [unwired: 2 in, 2 out]
      n187 = property on="Z MINPOS" class="DigNum (strict)"("Val(Sgnl)"=w206) -> ()  [unwired: 2 in, 2 out]
      n188 = property on="R MAXPOS" class="DigNum (strict)"("Val(Sgnl)"=w205) -> ()  [unwired: 2 in, 2 out]
      n189 = property on="R MINPOS" class="DigNum (strict)"("Val(Sgnl)"=w204) -> ()  [unwired: 2 in, 2 out]
      "X COM PORT" <- w249
      "Z COM PORT" <- w248
      "Y COM PORT" <- w247
      "R COM PORT" <- w246
    }
  }
  n190 = local write "FirstScan"(w4) -> ()
  n191 = local write "GOBACK"(w4) -> ()
  n192 = property on="Z Step SP" class="DigNum (strict)"("Maximum"=102400000.0 ("upper limit")) -> ()  [unwired: 2 in, 2 out]
  n193 = property on="Z Step SP" class="DigNum (strict)"("Minimum"=0.0 ("lower limit")) -> ()  [unwired: 2 in, 2 out]
  n194 = property on="R Step SP" class="DigNum (strict)"("Maximum"=0.0 ("Data Entry Limits:Maximum")) -> ()  [unwired: 2 in, 2 out]
  n195 = property on="R Step SP" class="DigNum (strict)"("Minimum"=-6144000.0 ("Data Entry Limits:Minimum")) -> ()  [unwired: 2 in, 2 out]
  n196 = while {
    tunnel: [w273] -> w43
    tunnel: [w276] -> w44
    tunnel: [w279] -> w52
    tunnel: [w272] -> w51
    tunnel: [w278] -> w46
    tunnel: [w277] -> w45
    tunnel: [w275] -> w42
    tunnel: [w274] -> w41
    tunnel: w16 -> [w295]
    tunnel: w15 -> [w293]
    tunnel: w14 -> [w291]
    tunnel: w13 -> [w289]
    tunnel: w12 -> [w294]
    tunnel: w11 -> [w292]
    tunnel: w10 -> [w290]
    tunnel: w9 -> [w288]
    tunnel: w8 -> [w269]
    tunnel: w7 -> [w268]
    shift-right: [w262] -> _
    shift-left: dbl[] [] -> [w260]
    shift-right: [w261] -> _
    shift-left: dbl[] [] -> [w259]
    stop <- w270 stop-if-true
    n197 = event shown="[15] \"Scan Go\": Mouse Up" {
      selector: _ -> [_ _ _ _ _ _ _ _ _ _ _ _ _ _ _ _ _ _]
      dyn-events: _ -> [_ _ _ _ _ _ _ _ _ _ _ _ _ _ _ _ _ _]
      timeout: 100 -> [_ _ _ _ _ _ _ _ _ _ _ _ _ _ _ _ _ _]
      tunnel: [w493 w1343 w1380 w1701 w2035 w2163 w2207 w2285 w2375 w2404 w2432 w2462 w2491 w2618 w2805 w2877 w3115 w3354] -> w285
      tunnel: [w494 w1338 w1381 w1702 w2036 w2160 w2204 w2282 w2372 w2401 w2430 w2459 w2488 w2615 w2806 w2878 w3116 w3355] -> w284
      tunnel: [w512 w1340 w1389 w1706 w2026 w2158 w2202 w2280 w2370 w2399 w2428 w2457 w2486 w2642 w2799 w2870 w3120 w3359] -> w281
      tunnel: [w511 w1345 w1388 w1705 w2025 w2165 w2209 w2287 w2377 w2406 w2435 w2464 w2493 w2641 w2798 w2868 w3119 w3358] -> w280
      tunnel: [w496 w1339 w1385 w1704 w2024 w2159 w2203 w2281 w2371 w2400 w2429 w2458 w2487 w2602 w2795 w2876 w3118 w3357] -> w282
      tunnel: [w495 w1344 w1384 w1703 w2023 w2164 w2208 w2286 w2376 w2405 w2434 w2463 w2492 w2601 w2794 w2875 w3117 w3356] -> w283
      tunnel: [w462 w1341 w1377 w1700 w2034 w2161 w2205 w2283 w2373 w2402 w2431 w2460 w2489 w2588 w2791 w2873 w3114 w3353] -> w287
      tunnel: [w461 w1342 w1376 w1699 w2033 w2162 w2206 w2284 w2374 w2403 w2433 w2461 w2490 w2587 w2790 w2872 w3113 w3352] -> w286
      tunnel: w295 -> [w490 w1340 w1391 w1713 w2029 w2158 w2202 w2280 w2370 w2399 w2428 w2457 w2486 w2637 w2789 w2866 w3126 w3347]
      tunnel: w294 -> [w489 w1345 w1390 w1714 w2054 w2165 w2209 w2287 w2377 w2406 w2435 w2464 w2493 w2638 w2787 w2865 w3128 w3351]
      tunnel: w293 -> [w488 w1339 w1386 w1711 w2032 w2159 w2203 w2281 w2371 w2400 w2429 w2458 w2487 w2603 w2788 w2864 w3125 w3346]
      tunnel: w292 -> [w487 w1344 w1387 w1712 w2053 w2164 w2208 w2286 w2376 w2405 w2434 w2463 w2492 w2604 w2786 w2863 w3127 w3350]
      tunnel: w291 -> [w486 w1338 w1382 w1709 w2039 w2160 w2204 w2282 w2372 w2401 w2430 w2459 w2488 w2616 w2785 w2862 w3124 w3345]
      tunnel: w290 -> [w485 w1343 w1383 w1710 w2052 w2163 w2207 w2285 w2375 w2404 w2432 w2462 w2491 w2617 w2783 w2861 w3122 w3349]
      tunnel: w289 -> [w484 w1341 w1378 w1707 w2042 w2161 w2205 w2283 w2373 w2402 w2431 w2460 w2489 w2589 w2784 w2860 w3123 w3344]
      tunnel: w288 -> [w483 w1342 w1379 w1708 w2051 w2162 w2206 w2284 w2374 w2403 w2433 w2461 w2490 w2590 w2782 w2859 w3121 w3348]
      tunnel: [w466 _ _ w1698 w2021 w2156 _ _ _ _ _ _ _ _ _ w2848 _ _] -> w262
      tunnel: [w464 _ _ w1697 w2020 w2155 _ _ _ _ _ _ _ _ _ w2847 _ _] -> w261
      tunnel: w260 -> [w469 _ _ w1698 w2021 w2156 _ _ _ _ _ _ _ _ _ w2848 _ _]
      tunnel: w259 -> [w468 _ _ w1697 w2020 w2155 _ _ _ _ _ _ _ _ _ w2847 _ _]
      event #0 {
        n198 = event-data() -> ()  [unwired: 1 in, 2 out]
        n199 = property on="GO" class="Bool"() -> ("DisabledEnum"=w482:T1)  [unwired: 2 in, 2 out]
        n200 = property on="GO" class="Bool"() -> ("DisabledEnum"=w479:T1)  [unwired: 2 in, 2 out]
        n201 = property on="Scan Go" class="Bool (strict)"() -> ("DisabledEnum"=w476:T1)  [unwired: 2 in, 2 out]
        n202 = Equal?(x=w482, y=T1."Disabled and Grayed Out") -> (x = y?=w480:bool)
        n203 = case shown="True" w480 {
          tunnel: [w539 w587] -> w512
          tunnel: [w538 w586] -> w511
          tunnel: [w537 w585] -> w496
          tunnel: [w536 w584] -> w495
          tunnel: [w535 w583] -> w494
          tunnel: [w534 w582] -> w493
          tunnel: [w533 w565] -> w462
          tunnel: [w532 w564] -> w461
          tunnel: w490 -> [w547 w581]
          tunnel: w489 -> [w546 w580]
          tunnel: w488 -> [w545 w579]
          tunnel: w487 -> [w544 w578]
          tunnel: w486 -> [w543 w577]
          tunnel: w485 -> [w542 w576]
          tunnel: w484 -> [w541 w575]
          tunnel: w483 -> [w540 w574]
          frame #0 {
            n204 = call "DigitalIO_sub_V1_MON.vi"() -> ("CL"=w526:bool, "OP"=w527:bool)  [unwired: 8 in]
            n205 = property on="CL" class="Bool (strict)"("Val(Sgnl)"=w526) -> ()  [unwired: 2 in, 2 out]
            n206 = property on="OP" class="Bool (strict)"("Val(Sgnl)"=w527) -> ()  [unwired: 2 in, 2 out]
            n207 = call "mDrive Send Command.vi"("error in (no error)"=w540, "Extra"="MV", "Command"=T10."Print Parameter", "VISA resource name"=w541) -> ("error out"=w532:errorcluster, "read buffer"=w549:string, "VISA resource name out"=w533:refnum<visa-resource-name>)  [unwired: 3 in]
            n208 = call "mDrive Send Command.vi"("error in (no error)"=w542, "Extra"="MV", "Command"=T10."Print Parameter", "VISA resource name"=w543) -> ("error out"=w534:errorcluster, "read buffer"=w553:string, "VISA resource name out"=w535:refnum<visa-resource-name>)  [unwired: 3 in]
            n209 = call "mDrive Send Command.vi"("error in (no error)"=w544, "Extra"="MV", "Command"=T10."Print Parameter", "VISA resource name"=w545) -> ("error out"=w536:errorcluster, "read buffer"=w557:string, "VISA resource name out"=w537:refnum<visa-resource-name>)  [unwired: 3 in]
            n210 = call "mDrive Send Command.vi"("error in (no error)"=w546, "Extra"="MV", "Command"=T10."Print Parameter", "VISA resource name"=w547) -> ("error out"=w538:errorcluster, "read buffer"=w561:string, "VISA resource name out"=w539:refnum<visa-resource-name>)  [unwired: 3 in]
            n211 = Not Equal?(x=w549, y="") -> (x != y?=w528:bool)
            n212 = Not Equal?(x=w553, y="") -> (x != y?=w529:bool)
            n213 = Not Equal?(x=w557, y="") -> (x != y?=w530:bool)
            n214 = Not Equal?(x=w561, y="") -> (x != y?=w531:bool)
            n215 = property on="R Ready" class="Bool (strict)"("Val(Sgnl)"=w528) -> ()  [unwired: 2 in, 2 out]
            n216 = property on="Z Ready" class="Bool (strict)"("Val(Sgnl)"=w530) -> ()  [unwired: 2 in, 2 out]
            n217 = property on="Y Ready" class="Bool (strict)"("Val(Sgnl)"=w529) -> ()  [unwired: 2 in, 2 out]
            n218 = property on="X Ready" class="Bool (strict)"("Val(Sgnl)"=w531) -> ()  [unwired: 2 in, 2 out]
          }
          frame #1 {
            n219 = flat-sequence {
              tunnel: w581 -> [w595]
              tunnel: w580 -> [w594]
              tunnel: w579 -> [w593]
              tunnel: w578 -> [w592]
              tunnel: w577 -> [w591]
              tunnel: w576 -> [w590]
              tunnel: w575 -> [w589]
              tunnel: w574 -> [w588]
              tunnel: [w603] -> w573
              tunnel: [w602] -> w572
              tunnel: [w601] -> w571
              tunnel: [w600] -> w570
              tunnel: [w599] -> w569
              tunnel: [w598] -> w568
              tunnel: [w597] -> w567
              tunnel: [w596] -> w566
              tunnel: [w1202] -> w564
              tunnel: [w1203] -> w565
              tunnel: [w1204] -> w582
              tunnel: [w1205] -> w583
              tunnel: [w1206] -> w584
              tunnel: [w1207] -> w585
              tunnel: [w1208] -> w586
              tunnel: [w1209] -> w587
              tunnel: w573 -> [w1209]
              tunnel: w572 -> [w1208]
              tunnel: w571 -> [w1207]
              tunnel: w570 -> [w1206]
              tunnel: w569 -> [w1205]
              tunnel: w568 -> [w1204]
              tunnel: w567 -> [w1203]
              tunnel: w566 -> [w1202]
              frame #0 {
                n220 = flat-sequence {
                  tunnel: [w934] -> w645
                  tunnel: [w925] -> w644
                  tunnel: [w924] -> w643
                  tunnel: w593 -> [w928]
                  tunnel: w592 -> [w927]
                  tunnel: [w966] -> w642
                  tunnel: [w965] -> w641
                  tunnel: [w964] -> w640
                  tunnel: [w957] -> w639
                  tunnel: w645 -> [w964]
                  tunnel: w644 -> [w963]
                  tunnel: w643 -> [w962]
                  tunnel: w642 -> [w976]
                  tunnel: [w976] -> w635
                  tunnel: w641 -> [w975]
                  tunnel: [w975] -> w636
                  tunnel: w640 -> [w974]
                  tunnel: [w974] -> w637
                  tunnel: w639 -> [w973]
                  tunnel: [w973] -> w638
                  tunnel: [w980] -> w634
                  tunnel: [w981] -> w633
                  tunnel: [w977] -> w632
                  tunnel: w638 -> [w977]
                  tunnel: w637 -> [w978]
                  tunnel: w636 -> [w982]
                  tunnel: w635 -> [w979]
                  tunnel: w634 -> [w993]
                  tunnel: w633 -> [w994]
                  tunnel: w632 -> [w996]
                  tunnel: [w992] -> w600
                  tunnel: [w991] -> w601
                  frame #0 {
                    n221 = call "mDrive Send Command.vi"("error in (no error)"=w927, "Extra"="P", "Command"=T10."Print Parameter", "VISA resource name"=w928) -> ("error out"=w924:errorcluster, "read buffer"=w944:string, "VISA resource name out"=w925:refnum<visa-resource-name>)  [unwired: 3 in]
                    n222 = property on="Z steps/rev" class="DigNum (strict)"() -> ("Value"=w933:u32)  [unwired: 2 in, 2 out]
                    n223 = To Double Precision Float(number=w933) -> (double precision float=w940:dbl)
                    n224 = Decimal String To Number(string=w944, offset=0) -> (number=w923:i32)  [unwired: 1 in, 1 out]
                    n225 = To Double Precision Float(number=w923) -> (double precision float=w938:dbl)
                    n226 = Divide(x=w938, y=w940) -> (x/y=w939:dbl)
                    n227 = property on="Z Step PV" class="DigNum (strict)"("Val(Sgnl)"=w923) -> ()  [unwired: 2 in, 2 out]
                    n228 = property on="Z mm/rev" class="DigNum (strict)"() -> ("Value"=w932:dbl)  [unwired: 2 in, 2 out]
                    n229 = property on="Z Step SP" class="DigNum (strict)"() -> ("Maximum"=w935:dbl)  [unwired: 2 in, 2 out]
                    n230 = property on="Z Step SP" class="DigNum (strict)"() -> ("Minimum"=w929:dbl)  [unwired: 2 in, 2 out]
                    n231 = Multiply(x=w939, y=w932) -> (x*y=w926:dbl)
                    n232 = To Long Integer(number=w935) -> (32bit integer=w941:i32)
                    n233 = To Long Integer(number=w929) -> (32bit integer=w942:i32)
                    n234 = property on="Z offset mm" class="DigNum (strict)"() -> ("Value"=w931:dbl)  [unwired: 2 in, 2 out]
                    n235 = In Range and Coerce(upper limit=w941, x=w923, lower limit=w942) -> (In Range?=w934:bool)  [unwired: 1 out]
                    n236 = Add(x=w926, y=w931) -> (x+y=w930:dbl)
                    n237 = property on="Z Position mm PV" class="DigNum (strict)"("Val(Sgnl)"=w930) -> ()  [unwired: 2 in, 2 out]
                    n238 = property on="Z in Range" class="Bool (strict)"("Val(Sgnl)"=w934) -> ()  [unwired: 2 in, 2 out]
                    n239 = property on="OK Button" class="Bool (strict)"() -> ("Value"=w920:bool)  [unwired: 2 in, 2 out]
                    n240 = Not Equal?(x=w920, y=TRUE) -> (x != y?=w918:bool)
                    n241 = Equal?(x=w923, y=15360000) -> (x = y?=w917:bool)
                    n242 = And(x=w917, y=w918) -> (x .and. y?=w916:bool)
                    n243 = case shown="False" w916 {
                      tunnel: [FALSE ("true") w955] -> w921
                      frame #0 {
                      }
                      frame #1 {
                        n244 = One Button Dialog(message="HAVE YOU OPEND THE VALVE???\nTHEN REWRITE YOUR POSITION\n AND PRESS GO!") -> (true=w955:bool)  [unwired: 1 in]
                      }
                    }
                    n245 = case shown="False" w921 {
                      frame #0 {
                        n246 = call "DigitalIO_sub_V1_MON.vi"() -> ("CL"=w945:bool, "OP"=w946:bool)  [unwired: 8 in]
                        n247 = property on="OP" class="Bool (strict)"("Val(Sgnl)"=w946) -> ()  [unwired: 2 in, 2 out]
                        n248 = property on="CL" class="Bool (strict)"("Val(Sgnl)"=w945) -> ()  [unwired: 2 in, 2 out]
                      }
                      frame #1 {
                        n249 = while {
                          stop <- w953 stop-if-true
                          n250 = property on="OK Button" class="Bool (strict)"() -> ("Value"=w947:bool)  [unwired: 2 in, 2 out]
                          n251 = call "ValveConrtoller.vi"("OK Button"=w947) -> ("OUTGOING SIGNAL"=w948:bool, "CL"=w949:bool, "OP"=w950:bool, "VALVE\nopend/closed"=w951:bool)  [unwired: 3 in]
                          n252 = property on="Valve \nopend/closed" class="Bool (strict)"("Val(Sgnl)"=w951) -> ()  [unwired: 2 in, 2 out]
                          n253 = property on="CL" class="Bool (strict)"("Val(Sgnl)"=w949) -> ()  [unwired: 2 in, 2 out]
                          n254 = Equal?(x=w948, y=TRUE) -> (x = y?=w953:bool)
                          n255 = property on="OP" class="Bool (strict)"("Val(Sgnl)"=w950) -> ()  [unwired: 2 in, 2 out]
                        }
                      }
                    }
                  }
                  frame #1 {
                    n256 = call "mDrive Send Command.vi"("error in (no error)"=w962, "Extra"="MV", "Command"=T10."Print Parameter", "VISA resource name"=w963) -> ("error out"=w965:errorcluster, "read buffer"=w968:string, "VISA resource name out"=w966:refnum<visa-resource-name>)  [unwired: 3 in]
                    n257 = Not Equal?(x=w968, y="") -> (x != y?=w961:bool)
                    n258 = Decimal String To Number(string=w968, offset=0 ("offset (0)")) -> (number=w958:i32)  [unwired: 1 in, 1 out]
                    n259 = property on="Z Ready" class="Bool (strict)"("Val(Sgnl)"=w961) -> ()  [unwired: 2 in, 2 out]
                    n260 = Number To Boolean Array(number=w958) -> (Boolean array=w960:bool[])
                    n261 = Index Array(array=w960, index=0) -> (element=w957:bool)
                    n262 = property on="Z in Motion" class="Bool (strict)"("Val(Sgnl)"=w957) -> ()  [unwired: 2 in, 2 out]
                  }
                  frame #2 {
                    n263 = Wait (ms)(milliseconds to wait=u32 50) -> ()  [unwired: 1 out]
                  }
                  frame #3 {
                    n264 = case shown="True" w978 {
                      tunnel: w979 -> [w985 w989]
                      tunnel: [w986 w989] -> w980
                      tunnel: [w987 w988] -> w981
                      tunnel: w982 -> [w984 w988]
                      frame #0 {
                        n265 = call "mDrive Send Command.vi"("error in (no error)"=w984, "Command"=T10."Stop", "VISA resource name"=w985) -> ("error out"=w987:errorcluster, "VISA resource name out"=w986:refnum<visa-resource-name>)  [unwired: 4 in, 1 out]
                      }
                      frame #1 {
                      }
                    }
                  }
                  frame #4 {
                    n266 = property on="Z Backlash corr" class="Bool (strict)"() -> ("Value"=w990:bool)  [unwired: 2 in, 2 out]
                    n267 = Implies(1:w996, 2:w990) -> (0:w995:bool)
                    n268 = case shown="True" w995 {
                      tunnel: w994 -> [w1004 w1061]
                      tunnel: w993 -> [w1003 w1062]
                      tunnel: [w998 w1061] -> w992
                      tunnel: [w1002 w1062] -> w991
                      frame #0 {
                        # "Backlash"
                        n269 = flat-sequence {
                          tunnel: [w1017] -> w1016
                          tunnel: [w1021] -> w1015
                          tunnel: [w1020] -> w1014
                          tunnel: w1004 -> [w1019]
                          tunnel: w1003 -> [w1018]
                          tunnel: w1016 -> [w1029]
                          tunnel: [w1029] -> w1013
                          tunnel: w1015 -> [w1028]
                          tunnel: w1014 -> [w1027]
                          tunnel: [w1026] -> w1012
                          tunnel: [w1025] -> w1011
                          tunnel: [w1024] -> w1001
                          tunnel: w1013 -> [w1043]
                          tunnel: w1012 -> [w1034]
                          tunnel: w1011 -> [w1042]
                          tunnel: [w1034] -> w1010
                          tunnel: [w1042] -> w1009
                          tunnel: [w1033] -> w1006
                          tunnel: [w1041] -> w1005
                          tunnel: w1001 -> [w1041]
                          tunnel: w1010 -> [w1046]
                          tunnel: w1009 -> [w1047]
                          tunnel: [w1045] -> w1008
                          tunnel: [w1053] -> w1007
                          tunnel: w1006 -> [w1053]
                          tunnel: w1005 -> [w1049]
                          tunnel: [w1048] -> w999
                          tunnel: w1008 -> [w1056]
                          tunnel: w1007 -> [w1055]
                          tunnel: [w1057] -> w1000
                          tunnel: w999 -> [w1057]
                          tunnel: [w1056] -> w997
                          tunnel: [w1060] -> w1002
                          tunnel: w1000 -> [w1060]
                          tunnel: [w1059] -> w998
                          tunnel: w997 -> [w1059]
                          frame #0 {
                            n270 = property on="Z Backlash steps/sec" class="DigNum (strict)"() -> ("Value"=w1017:i32)  [unwired: 2 in, 2 out]
                            n271 = Number To Decimal String(number=w1017) -> (decimal integer string=w1022:string)  [unwired: 1 in]
                            n272 = call "mDrive Send Command.vi"("error in (no error)"=w1019, "Extra"=w1022, "Command"=T10."Max Velocity", "VISA resource name"=w1018) -> ("error out"=w1020:errorcluster, "VISA resource name out"=w1021:refnum<visa-resource-name>)  [unwired: 3 in, 1 out]
                          }
                          frame #1 {
                            n273 = property on="Z Backlash" class="DigNum (strict)"() -> ("Value"=w1024:i32)  [unwired: 2 in, 2 out]
                            n274 = Number To Decimal String(number=w1024) -> (decimal integer string=w1030:string)  [unwired: 1 in]
                            n275 = call "mDrive Send Command.vi"("error in (no error)"=w1027, "Extra"=w1030, "Command"=T10."Move to Relative Position", "VISA resource name"=w1028) -> ("error out"=w1026:errorcluster, "VISA resource name out"=w1025:refnum<visa-resource-name>)  [unwired: 3 in, 1 out]
                          }
                          frame #2 {
                            n276 = To Double Precision Float(number=w1041) -> (double precision float=w1039:dbl)
                            n277 = To Double Precision Float(number=w1043) -> (double precision float=w1044:dbl)
                            n278 = Absolute Value(x=w1039) -> (abs(x)=w1040:dbl)
                            n279 = Divide(x=w1040, y=w1044) -> (x/y=w1037:dbl)
                            n280 = Multiply(x=1000.0, y=w1037) -> (x*y=w1035:dbl)
                            n281 = Add(x=w1035, y=300.0) -> (x+y=w1033:dbl)
                            n282 = To Unsigned Long Integer(number=w1033) -> (unsigned 32bit integer=w1032:u32)
                            n283 = Wait (ms)(milliseconds to wait=w1032) -> ()  [unwired: 1 out]
                          }
                          frame #3 {
                            n284 = Negate(x=w1049) -> (-x=w1050:i32)
                            n285 = Number To Decimal String(number=w1050) -> (decimal integer string=w1051:string)  [unwired: 1 in]
                            n286 = call "mDrive Send Command.vi"("error in (no error)"=w1046, "Extra"=w1051, "Command"=T10."Move to Relative Position", "VISA resource name"=w1047) -> ("error out"=w1045:errorcluster, "VISA resource name out"=w1048:refnum<visa-resource-name>)  [unwired: 3 in, 1 out]
                          }
                          frame #4 {
                            n287 = To Unsigned Long Integer(number=w1055) -> (unsigned 32bit integer=w1054:u32)
                            n288 = Wait (ms)(milliseconds to wait=w1054) -> ()  [unwired: 1 out]
                          }
                          frame #5 {
                            n289 = property on="Z Backlash corr" class="Bool (strict)"("Val(Sgnl)"=FALSE ("Value (Signaling)")) -> ()  [unwired: 2 in, 2 out]
                          }
                        }
                      }
                      frame #1 {
                      }
                    }
                  }
                }
                n290 = flat-sequence {
                  tunnel: [w797] -> w631
                  tunnel: [w799] -> w630
                  tunnel: [w798] -> w629
                  tunnel: w591 -> [w790]
                  tunnel: w590 -> [w789]
                  tunnel: [w819] -> w628
                  tunnel: [w818] -> w627
                  tunnel: [w817] -> w626
                  tunnel: [w810] -> w625
                  tunnel: w631 -> [w817]
                  tunnel: w630 -> [w816]
                  tunnel: w629 -> [w815]
                  tunnel: w628 -> [w829]
                  tunnel: [w829] -> w621
                  tunnel: w627 -> [w828]
                  tunnel: [w828] -> w622
                  tunnel: w626 -> [w827]
                  tunnel: [w827] -> w623
                  tunnel: w625 -> [w826]
                  tunnel: [w826] -> w624
                  tunnel: [w833] -> w620
                  tunnel: [w834] -> w619
                  tunnel: [w830] -> w618
                  tunnel: w624 -> [w830]
                  tunnel: w623 -> [w831]
                  tunnel: w622 -> [w835]
                  tunnel: w621 -> [w832]
                  tunnel: w620 -> [w846]
                  tunnel: w619 -> [w847]
                  tunnel: w618 -> [w849]
                  tunnel: [w845] -> w598
                  tunnel: [w844] -> w599
                  frame #0 {
                    n291 = call "mDrive Send Command.vi"("error in (no error)"=w789, "Extra"="P", "Command"=T10."Print Parameter", "VISA resource name"=w790) -> ("error out"=w798:errorcluster, "read buffer"=w809:string, "VISA resource name out"=w799:refnum<visa-resource-name>)  [unwired: 3 in]
                    n292 = property on="Y steps/rev" class="DigNum (strict)"() -> ("Value"=w793:u32)  [unwired: 2 in, 2 out]
                    n293 = Decimal String To Number(string=w809, offset=0) -> (number=w788:i32)  [unwired: 1 in, 1 out]
                    n294 = To Double Precision Float(number=w793) -> (double precision float=w805:dbl)
                    n295 = To Double Precision Float(number=w788) -> (double precision float=w802:dbl)
                    n296 = property on="Y Step PV" class="DigNum (strict)"("Val(Sgnl)"=w788) -> ()  [unwired: 2 in, 2 out]
                    n297 = Divide(x=w802, y=w805) -> (x/y=w804:dbl)
                    n298 = property on="Y Step SP" class="DigNum (strict)"() -> ("Maximum"=w792:dbl)  [unwired: 2 in, 2 out]
                    n299 = property on="Y Step SP" class="DigNum (strict)"() -> ("Minimum"=w791:dbl)  [unwired: 2 in, 2 out]
                    n300 = property on="Y mm/rev" class="DigNum (strict)"() -> ("Value"=w794:dbl)  [unwired: 2 in, 2 out]
                    n301 = To Long Integer(number=w792) -> (32bit integer=w806:i32)
                    n302 = To Long Integer(number=w791) -> (32bit integer=w807:i32)
                    n303 = Multiply(x=w804, y=w794) -> (x*y=w803:dbl)
                    n304 = In Range and Coerce(upper limit=w806, x=w788, lower limit=w807) -> (In Range?=w797:bool)  [unwired: 1 out]
                    n305 = property on="Y offset mm" class="DigNum (strict)"() -> ("Value"=w795:dbl)  [unwired: 2 in, 2 out]
                    n306 = Add(x=w803, y=w795) -> (x+y=w796:dbl)
                    n307 = property on="Y in Range" class="Bool (strict)"("Val(Sgnl)"=w797) -> ()  [unwired: 2 in, 2 out]
                    n308 = property on="Y Position mm PV" class="DigNum (strict)"("Val(Sgnl)"=w796) -> ()  [unwired: 2 in, 2 out]
                  }
                  frame #1 {
                    n309 = call "mDrive Send Command.vi"("error in (no error)"=w815, "Extra"="MV", "Command"=T10."Print Parameter", "VISA resource name"=w816) -> ("error out"=w818:errorcluster, "read buffer"=w821:string, "VISA resource name out"=w819:refnum<visa-resource-name>)  [unwired: 3 in]
                    n310 = Not Equal?(x=w821, y="") -> (x != y?=w814:bool)
                    n311 = Decimal String To Number(string=w821, offset=0 ("offset (0)")) -> (number=w811:i32)  [unwired: 1 in, 1 out]
                    n312 = property on="Y Ready" class="Bool (strict)"("Val(Sgnl)"=w814) -> ()  [unwired: 2 in, 2 out]
                    n313 = Number To Boolean Array(number=w811) -> (Boolean array=w813:bool[])
                    n314 = Index Array(array=w813, index=0) -> (element=w810:bool)
                    n315 = property on="Y in Motion" class="Bool (strict)"("Val(Sgnl)"=w810) -> ()  [unwired: 2 in, 2 out]
                  }
                  frame #2 {
                    n316 = Wait (ms)(milliseconds to wait=u32 50) -> ()  [unwired: 1 out]
                  }
                  frame #3 {
                    n317 = case shown="True" w831 {
                      tunnel: w832 -> [w838 w841]
                      tunnel: [w839 w841] -> w833
                      tunnel: [w840 w842] -> w834
                      tunnel: w835 -> [w837 w842]
                      frame #0 {
                        n318 = call "mDrive Send Command.vi"("error in (no error)"=w837, "Command"=T10."Stop", "VISA resource name"=w838) -> ("error out"=w840:errorcluster, "VISA resource name out"=w839:refnum<visa-resource-name>)  [unwired: 4 in, 1 out]
                      }
                      frame #1 {
                      }
                    }
                  }
                  frame #4 {
                    n319 = property on="Y Backlash corr" class="Bool (strict)"() -> ("Value"=w843:bool)  [unwired: 2 in, 2 out]
                    n320 = Implies(1:w849, 2:w843) -> (0:w848:bool)
                    n321 = case shown="True" w848 {
                      tunnel: w847 -> [w857 w914]
                      tunnel: w846 -> [w856 w915]
                      tunnel: [w851 w914] -> w845
                      tunnel: [w855 w915] -> w844
                      frame #0 {
                        # "Backlash"
                        n322 = flat-sequence {
                          tunnel: [w870] -> w869
                          tunnel: [w874] -> w868
                          tunnel: [w873] -> w867
                          tunnel: w857 -> [w872]
                          tunnel: w856 -> [w871]
                          tunnel: w869 -> [w882]
                          tunnel: [w882] -> w866
                          tunnel: w868 -> [w881]
                          tunnel: w867 -> [w880]
                          tunnel: [w879] -> w865
                          tunnel: [w878] -> w864
                          tunnel: [w877] -> w854
                          tunnel: w866 -> [w896]
                          tunnel: w865 -> [w887]
                          tunnel: w864 -> [w895]
                          tunnel: [w887] -> w863
                          tunnel: [w895] -> w862
                          tunnel: [w886] -> w859
                          tunnel: [w894] -> w858
                          tunnel: w854 -> [w894]
                          tunnel: w863 -> [w899]
                          tunnel: w862 -> [w900]
                          tunnel: [w898] -> w861
                          tunnel: [w906] -> w860
                          tunnel: w859 -> [w906]
                          tunnel: w858 -> [w902]
                          tunnel: [w901] -> w852
                          tunnel: w861 -> [w909]
                          tunnel: w860 -> [w908]
                          tunnel: [w910] -> w853
                          tunnel: w852 -> [w910]
                          tunnel: [w909] -> w850
                          tunnel: [w913] -> w855
                          tunnel: w853 -> [w913]
                          tunnel: [w912] -> w851
                          tunnel: w850 -> [w912]
                          frame #0 {
                            n323 = property on="Y Backlash steps/sec" class="DigNum (strict)"() -> ("Value"=w870:i32)  [unwired: 2 in, 2 out]
                            n324 = Number To Decimal String(number=w870) -> (decimal integer string=w875:string)  [unwired: 1 in]
                            n325 = call "mDrive Send Command.vi"("error in (no error)"=w872, "Extra"=w875, "Command"=T10."Max Velocity", "VISA resource name"=w871) -> ("error out"=w873:errorcluster, "VISA resource name out"=w874:refnum<visa-resource-name>)  [unwired: 3 in, 1 out]
                          }
                          frame #1 {
                            n326 = property on="Y Backlash" class="DigNum (strict)"() -> ("Value"=w877:i32)  [unwired: 2 in, 2 out]
                            n327 = Number To Decimal String(number=w877) -> (decimal integer string=w883:string)  [unwired: 1 in]
                            n328 = call "mDrive Send Command.vi"("error in (no error)"=w880, "Extra"=w883, "Command"=T10."Move to Relative Position", "VISA resource name"=w881) -> ("error out"=w879:errorcluster, "VISA resource name out"=w878:refnum<visa-resource-name>)  [unwired: 3 in, 1 out]
                          }
                          frame #2 {
                            n329 = To Double Precision Float(number=w894) -> (double precision float=w892:dbl)
                            n330 = To Double Precision Float(number=w896) -> (double precision float=w897:dbl)
                            n331 = Absolute Value(x=w892) -> (abs(x)=w893:dbl)
                            n332 = Divide(x=w893, y=w897) -> (x/y=w890:dbl)
                            n333 = Multiply(x=1000.0, y=w890) -> (x*y=w888:dbl)
                            n334 = Add(x=w888, y=300.0) -> (x+y=w886:dbl)
                            n335 = To Unsigned Long Integer(number=w886) -> (unsigned 32bit integer=w885:u32)
                            n336 = Wait (ms)(milliseconds to wait=w885) -> ()  [unwired: 1 out]
                          }
                          frame #3 {
                            n337 = Negate(x=w902) -> (-x=w903:i32)
                            n338 = Number To Decimal String(number=w903) -> (decimal integer string=w904:string)  [unwired: 1 in]
                            n339 = call "mDrive Send Command.vi"("error in (no error)"=w899, "Extra"=w904, "Command"=T10."Move to Relative Position", "VISA resource name"=w900) -> ("error out"=w898:errorcluster, "VISA resource name out"=w901:refnum<visa-resource-name>)  [unwired: 3 in, 1 out]
                          }
                          frame #4 {
                            n340 = To Unsigned Long Integer(number=w908) -> (unsigned 32bit integer=w907:u32)
                            n341 = Wait (ms)(milliseconds to wait=w907) -> ()  [unwired: 1 out]
                          }
                          frame #5 {
                            n342 = property on="Y Backlash corr" class="Bool (strict)"("Val(Sgnl)"=FALSE ("Value (Signaling)")) -> ()  [unwired: 2 in, 2 out]
                          }
                        }
                      }
                      frame #1 {
                      }
                    }
                  }
                }
                n343 = flat-sequence {
                  tunnel: [w669] -> w617
                  tunnel: [w671] -> w616
                  tunnel: [w670] -> w615
                  tunnel: w589 -> [w662]
                  tunnel: w588 -> [w661]
                  tunnel: [w691] -> w614
                  tunnel: [w690] -> w613
                  tunnel: [w689] -> w612
                  tunnel: [w682] -> w611
                  tunnel: w617 -> [w689]
                  tunnel: w616 -> [w688]
                  tunnel: w615 -> [w687]
                  tunnel: w614 -> [w701]
                  tunnel: [w701] -> w607
                  tunnel: w613 -> [w700]
                  tunnel: [w700] -> w608
                  tunnel: w612 -> [w699]
                  tunnel: [w699] -> w609
                  tunnel: w611 -> [w698]
                  tunnel: [w698] -> w610
                  tunnel: [w705] -> w606
                  tunnel: [w706] -> w605
                  tunnel: [w702] -> w604
                  tunnel: w610 -> [w702]
                  tunnel: w609 -> [w703]
                  tunnel: w608 -> [w707]
                  tunnel: w607 -> [w704]
                  tunnel: w606 -> [w718]
                  tunnel: w605 -> [w719]
                  tunnel: w604 -> [w721]
                  tunnel: [w717] -> w596
                  tunnel: [w716] -> w597
                  frame #0 {
                    n344 = call "mDrive Send Command.vi"("error in (no error)"=w661, "Extra"="P", "Command"=T10."Print Parameter", "VISA resource name"=w662) -> ("error out"=w670:errorcluster, "read buffer"=w681:string, "VISA resource name out"=w671:refnum<visa-resource-name>)  [unwired: 3 in]
                    n345 = property on="R steps/rev" class="DigNum (strict)"() -> ("Value"=w663:u32)  [unwired: 2 in, 2 out]
                    n346 = Decimal String To Number(string=w681, offset=0) -> (number=w660:i32)  [unwired: 1 in, 1 out]
                    n347 = To Double Precision Float(number=w663) -> (double precision float=w677:dbl)
                    n348 = To Double Precision Float(number=w660) -> (double precision float=w674:dbl)
                    n349 = property on="R Step PV" class="DigNum (strict)"("Val(Sgnl)"=w660) -> ()  [unwired: 2 in, 2 out]
                    n350 = Divide(x=w674, y=w677) -> (x/y=w676:dbl)
                    n351 = property on="R Step SP" class="DigNum (strict)"() -> ("Maximum"=w664:dbl)  [unwired: 2 in, 2 out]
                    n352 = property on="R Step SP" class="DigNum (strict)"() -> ("Minimum"=w665:dbl)  [unwired: 2 in, 2 out]
                    n353 = property on="R deg/rev" class="DigNum (strict)"() -> ("Value"=w666:dbl)  [unwired: 2 in, 2 out]
                    n354 = Multiply(x=w676, y=w666) -> (x*y=w675:dbl)
                    n355 = To Long Integer(number=w664) -> (32bit integer=w678:i32)
                    n356 = To Long Integer(number=w665) -> (32bit integer=w679:i32)
                    n357 = property on="R offset deg" class="DigNum (strict)"() -> ("Value"=w667:dbl)  [unwired: 2 in, 2 out]
                    n358 = In Range and Coerce(upper limit=w678, x=w660, lower limit=w679) -> (In Range?=w669:bool)  [unwired: 1 out]
                    n359 = Add(x=w675, y=w667) -> (x+y=w668:dbl)
                    n360 = property on="R in Range" class="Bool (strict)"("Val(Sgnl)"=w669) -> ()  [unwired: 2 in, 2 out]
                    n361 = property on="R Position deg PV" class="DigNum (strict)"("Val(Sgnl)"=w668) -> ()  [unwired: 2 in, 2 out]
                  }
                  frame #1 {
                    n362 = call "mDrive Send Command.vi"("error in (no error)"=w687, "Extra"="MV", "Command"=T10."Print Parameter", "VISA resource name"=w688) -> ("error out"=w690:errorcluster, "read buffer"=w693:string, "VISA resource name out"=w691:refnum<visa-resource-name>)  [unwired: 3 in]
                    n363 = Not Equal?(x=w693, y="") -> (x != y?=w686:bool)
                    n364 = Decimal String To Number(string=w693, offset=0 ("offset (0)")) -> (number=w683:i32)  [unwired: 1 in, 1 out]
                    n365 = Number To Boolean Array(number=w683) -> (Boolean array=w685:bool[])
                    n366 = property on="R Ready" class="Bool (strict)"("Val(Sgnl)"=w686) -> ()  [unwired: 2 in, 2 out]
                    n367 = Index Array(array=w685, index=0) -> (element=w682:bool)
                    n368 = property on="R in Motion" class="Bool (strict)"("Val(Sgnl)"=w682) -> ()  [unwired: 2 in, 2 out]
                  }
                  frame #2 {
                    n369 = Wait (ms)(milliseconds to wait=u32 50) -> ()  [unwired: 1 out]
                  }
                  frame #3 {
                    n370 = case shown="True" w703 {
                      tunnel: w704 -> [w710 w714]
                      tunnel: [w711 w714] -> w705
                      tunnel: [w712 w713] -> w706
                      tunnel: w707 -> [w709 w713]
                      frame #0 {
                        n371 = call "mDrive Send Command.vi"("error in (no error)"=w709, "Command"=T10."Stop", "VISA resource name"=w710) -> ("error out"=w712:errorcluster, "VISA resource name out"=w711:refnum<visa-resource-name>)  [unwired: 4 in, 1 out]
                      }
                      frame #1 {
                      }
                    }
                  }
                  frame #4 {
                    n372 = property on="R Backlash corr" class="Bool (strict)"() -> ("Value"=w715:bool)  [unwired: 2 in, 2 out]
                    n373 = Implies(1:w721, 2:w715) -> (0:w720:bool)
                    n374 = case shown="True" w720 {
                      tunnel: w719 -> [w729 w786]
                      tunnel: w718 -> [w728 w787]
                      tunnel: [w723 w786] -> w717
                      tunnel: [w727 w787] -> w716
                      frame #0 {
                        # "Backlash"
                        n375 = flat-sequence {
                          tunnel: [w742] -> w741
                          tunnel: [w746] -> w740
                          tunnel: [w745] -> w739
                          tunnel: w729 -> [w744]
                          tunnel: w728 -> [w743]
                          tunnel: w741 -> [w754]
                          tunnel: [w754] -> w738
                          tunnel: w740 -> [w753]
                          tunnel: w739 -> [w752]
                          tunnel: [w751] -> w737
                          tunnel: [w750] -> w736
                          tunnel: [w749] -> w726
                          tunnel: w738 -> [w768]
                          tunnel: w737 -> [w759]
                          tunnel: w736 -> [w767]
                          tunnel: [w759] -> w735
                          tunnel: [w767] -> w734
                          tunnel: [w758] -> w731
                          tunnel: [w766] -> w730
                          tunnel: w726 -> [w766]
                          tunnel: w735 -> [w771]
                          tunnel: w734 -> [w772]
                          tunnel: [w770] -> w733
                          tunnel: [w778] -> w732
                          tunnel: w731 -> [w778]
                          tunnel: w730 -> [w774]
                          tunnel: [w773] -> w724
                          tunnel: w733 -> [w781]
                          tunnel: w732 -> [w780]
                          tunnel: [w782] -> w725
                          tunnel: w724 -> [w782]
                          tunnel: [w781] -> w722
                          tunnel: [w785] -> w727
                          tunnel: w725 -> [w785]
                          tunnel: [w784] -> w723
                          tunnel: w722 -> [w784]
                          frame #0 {
                            n376 = property on="R Backlash steps/sec" class="DigNum (strict)"() -> ("Value"=w742:i32)  [unwired: 2 in, 2 out]
                            n377 = Number To Decimal String(number=w742) -> (decimal integer string=w747:string)  [unwired: 1 in]
                            n378 = call "mDrive Send Command.vi"("error in (no error)"=w744, "Extra"=w747, "Command"=T10."Max Velocity", "VISA resource name"=w743) -> ("error out"=w745:errorcluster, "VISA resource name out"=w746:refnum<visa-resource-name>)  [unwired: 3 in, 1 out]
                          }
                          frame #1 {
                            n379 = property on="R Backlash" class="DigNum (strict)"() -> ("Value"=w749:i32)  [unwired: 2 in, 2 out]
                            n380 = Number To Decimal String(number=w749) -> (decimal integer string=w755:string)  [unwired: 1 in]
                            n381 = call "mDrive Send Command.vi"("error in (no error)"=w752, "Extra"=w755, "Command"=T10."Move to Relative Position", "VISA resource name"=w753) -> ("error out"=w751:errorcluster, "VISA resource name out"=w750:refnum<visa-resource-name>)  [unwired: 3 in, 1 out]
                          }
                          frame #2 {
                            n382 = To Double Precision Float(number=w766) -> (double precision float=w764:dbl)
                            n383 = To Double Precision Float(number=w768) -> (double precision float=w769:dbl)
                            n384 = Absolute Value(x=w764) -> (abs(x)=w765:dbl)
                            n385 = Divide(x=w765, y=w769) -> (x/y=w762:dbl)
                            n386 = Multiply(x=1000.0, y=w762) -> (x*y=w760:dbl)
                            n387 = Add(x=w760, y=300.0) -> (x+y=w758:dbl)
                            n388 = To Unsigned Long Integer(number=w758) -> (unsigned 32bit integer=w757:u32)
                            n389 = Wait (ms)(milliseconds to wait=w757) -> ()  [unwired: 1 out]
                          }
                          frame #3 {
                            n390 = Negate(x=w774) -> (-x=w775:i32)
                            n391 = Number To Decimal String(number=w775) -> (decimal integer string=w776:string)  [unwired: 1 in]
                            n392 = call "mDrive Send Command.vi"("error in (no error)"=w771, "Extra"=w776, "Command"=T10."Move to Relative Position", "VISA resource name"=w772) -> ("error out"=w770:errorcluster, "VISA resource name out"=w773:refnum<visa-resource-name>)  [unwired: 3 in, 1 out]
                          }
                          frame #4 {
                            n393 = To Unsigned Long Integer(number=w780) -> (unsigned 32bit integer=w779:u32)
                            n394 = Wait (ms)(milliseconds to wait=w779) -> ()  [unwired: 1 out]
                          }
                          frame #5 {
                            n395 = property on="R Backlash corr" class="Bool (strict)"("Val(Sgnl)"=FALSE ("Value (Signaling)")) -> ()  [unwired: 2 in, 2 out]
                          }
                        }
                      }
                      frame #1 {
                      }
                    }
                  }
                }
                n396 = flat-sequence {
                  tunnel: [w1068] -> w659
                  tunnel: [w1067] -> w658
                  tunnel: [w1066] -> w657
                  tunnel: w595 -> [w1065]
                  tunnel: w594 -> [w1064]
                  tunnel: [w1090] -> w656
                  tunnel: [w1089] -> w655
                  tunnel: [w1087] -> w654
                  tunnel: [w1088] -> w653
                  tunnel: w659 -> [w1087]
                  tunnel: w658 -> [w1086]
                  tunnel: w657 -> [w1085]
                  tunnel: w656 -> [w1104]
                  tunnel: [w1104] -> w649
                  tunnel: w655 -> [w1103]
                  tunnel: [w1103] -> w650
                  tunnel: w654 -> [w1102]
                  tunnel: [w1102] -> w651
                  tunnel: w653 -> [w1101]
                  tunnel: [w1101] -> w652
                  tunnel: [w1108] -> w648
                  tunnel: [w1109] -> w647
                  tunnel: [w1105] -> w646
                  tunnel: w652 -> [w1105]
                  tunnel: w651 -> [w1106]
                  tunnel: w650 -> [w1110]
                  tunnel: w649 -> [w1107]
                  tunnel: w648 -> [w1120]
                  tunnel: w647 -> [w1121]
                  tunnel: w646 -> [w1123]
                  tunnel: [w1119] -> w602
                  tunnel: [w1118] -> w603
                  frame #0 {
                    n397 = call "mDrive Send Command.vi"("error in (no error)"=w1064, "Extra"="P", "Command"=T10."Print Parameter", "VISA resource name"=w1065) -> ("error out"=w1066:errorcluster, "read buffer"=w1084:string, "VISA resource name out"=w1067:refnum<visa-resource-name>)  [unwired: 3 in]
                    n398 = Decimal String To Number(string=w1084, offset=0) -> (number=w1063:i32)  [unwired: 1 in, 1 out]
                    n399 = property on="X steps/rev" class="DigNum (strict)"() -> ("Value"=w1077:u32)  [unwired: 2 in, 2 out]
                    n400 = To Double Precision Float(number=w1063) -> (double precision float=w1072:dbl)
                    n401 = To Double Precision Float(number=w1077) -> (double precision float=w1078:dbl)
                    n402 = property on="X Step PV" class="DigNum (strict)"("Val(Sgnl)"=w1063) -> ()  [unwired: 2 in, 2 out]
                    n403 = Divide(x=w1072, y=w1078) -> (x/y=w1076:dbl)
                    n404 = property on="X Step SP" class="DigNum (strict)"() -> ("Maximum"=w1080:dbl)  [unwired: 2 in, 2 out]
                    n405 = property on="X Step SP" class="DigNum (strict)"() -> ("Minimum"=w1082:dbl)  [unwired: 2 in, 2 out]
                    n406 = property on="X mm/rev" class="DigNum (strict)"() -> ("Value"=w1075:dbl)  [unwired: 2 in, 2 out]
                    n407 = Multiply(x=w1076, y=w1075) -> (x*y=w1074:dbl)
                    n408 = To Long Integer(number=w1080) -> (32bit integer=w1079:i32)
                    n409 = To Long Integer(number=w1082) -> (32bit integer=w1081:i32)
                    n410 = property on="X offset mm" class="DigNum (strict)"() -> ("Value"=w1073:dbl)  [unwired: 2 in, 2 out]
                    n411 = In Range and Coerce(upper limit=w1079, x=w1063, lower limit=w1081) -> (In Range?=w1068:bool)  [unwired: 1 out]
                    n412 = Add(x=w1074, y=w1073) -> (x+y=w1071:dbl)
                    n413 = property on="X  in Range" class="Bool (strict)"("Val(Sgnl)"=w1068) -> ()  [unwired: 2 in, 2 out]
                    n414 = property on="X Position mm PV" class="DigNum (strict)"("Val(Sgnl)"=w1071) -> ()  [unwired: 2 in, 2 out]
                  }
                  frame #1 {
                    n415 = call "mDrive Send Command.vi"("error in (no error)"=w1085, "Extra"="MV", "Command"=T10."Print Parameter", "VISA resource name"=w1086) -> ("error out"=w1089:errorcluster, "read buffer"=w1093:string, "VISA resource name out"=w1090:refnum<visa-resource-name>)  [unwired: 3 in]
                    n416 = Not Equal?(x=w1093, y="") -> (x != y?=w1091:bool)
                    n417 = Decimal String To Number(string=w1093, offset=0 ("offset (0)")) -> (number=w1096:i32)  [unwired: 1 in, 1 out]
                    n418 = property on="X Ready" class="Bool (strict)"("Val(Sgnl)"=w1091) -> ()  [unwired: 2 in, 2 out]
                    n419 = Number To Boolean Array(number=w1096) -> (Boolean array=w1095:bool[])
                    n420 = Index Array(array=w1095, index=0) -> (element=w1088:bool)
                    n421 = property on="X  in Motion" class="Bool (strict)"("Val(Sgnl)"=w1088) -> ()  [unwired: 2 in, 2 out]
                  }
                  frame #2 {
                    n422 = Wait (ms)(milliseconds to wait=u32 50) -> ()  [unwired: 1 out]
                  }
                  frame #3 {
                    n423 = case shown="True" w1106 {
                      tunnel: w1107 -> [w1113 w1117]
                      tunnel: [w1114 w1117] -> w1108
                      tunnel: [w1115 w1116] -> w1109
                      tunnel: w1110 -> [w1112 w1116]
                      frame #0 {
                        n424 = call "mDrive Send Command.vi"("error in (no error)"=w1112, "Command"=T10."Stop", "VISA resource name"=w1113) -> ("error out"=w1115:errorcluster, "VISA resource name out"=w1114:refnum<visa-resource-name>)  [unwired: 4 in, 1 out]
                      }
                      frame #1 {
                      }
                    }
                  }
                  frame #4 {
                    n425 = property on="X Backlash corr" class="Bool (strict)"() -> ("Value"=w1124:bool)  [unwired: 2 in, 2 out]
                    n426 = Implies(1:w1123, 2:w1124) -> (0:w1122:bool)
                    n427 = case shown="True" w1122 {
                      tunnel: w1121 -> [w1132 w1189]
                      tunnel: w1120 -> [w1131 w1190]
                      tunnel: [w1126 w1189] -> w1119
                      tunnel: [w1130 w1190] -> w1118
                      frame #0 {
                        # "Backlash"
                        n428 = flat-sequence {
                          tunnel: [w1147] -> w1144
                          tunnel: [w1149] -> w1143
                          tunnel: [w1148] -> w1142
                          tunnel: w1132 -> [w1146]
                          tunnel: w1131 -> [w1145]
                          tunnel: w1144 -> [w1157]
                          tunnel: [w1157] -> w1141
                          tunnel: w1143 -> [w1156]
                          tunnel: w1142 -> [w1155]
                          tunnel: [w1154] -> w1140
                          tunnel: [w1153] -> w1139
                          tunnel: [w1152] -> w1129
                          tunnel: w1141 -> [w1171]
                          tunnel: w1140 -> [w1162]
                          tunnel: w1139 -> [w1170]
                          tunnel: [w1162] -> w1138
                          tunnel: [w1170] -> w1137
                          tunnel: [w1161] -> w1134
                          tunnel: [w1169] -> w1133
                          tunnel: w1129 -> [w1169]
                          tunnel: w1138 -> [w1174]
                          tunnel: w1137 -> [w1175]
                          tunnel: [w1173] -> w1136
                          tunnel: [w1181] -> w1135
                          tunnel: w1134 -> [w1181]
                          tunnel: w1133 -> [w1177]
                          tunnel: [w1176] -> w1127
                          tunnel: w1136 -> [w1184]
                          tunnel: w1135 -> [w1183]
                          tunnel: [w1185] -> w1128
                          tunnel: w1127 -> [w1185]
                          tunnel: [w1184] -> w1125
                          tunnel: [w1188] -> w1130
                          tunnel: w1128 -> [w1188]
                          tunnel: [w1186] -> w1126
                          tunnel: w1125 -> [w1186]
                          frame #0 {
                            n429 = property on="X Backlash steps/sec" class="DigNum (strict)"() -> ("Value"=w1147:i32)  [unwired: 2 in, 2 out]
                            n430 = Number To Decimal String(number=w1147) -> (decimal integer string=w1150:string)  [unwired: 1 in]
                            n431 = call "mDrive Send Command.vi"("error in (no error)"=w1146, "Extra"=w1150, "Command"=T10."Max Velocity", "VISA resource name"=w1145) -> ("error out"=w1148:errorcluster, "VISA resource name out"=w1149:refnum<visa-resource-name>)  [unwired: 3 in, 1 out]
                          }
                          frame #1 {
                            n432 = property on="X Backlash" class="DigNum (strict)"() -> ("Value"=w1152:i32)  [unwired: 2 in, 2 out]
                            n433 = Number To Decimal String(number=w1152) -> (decimal integer string=w1158:string)  [unwired: 1 in]
                            n434 = call "mDrive Send Command.vi"("error in (no error)"=w1155, "Extra"=w1158, "Command"=T10."Move to Relative Position", "VISA resource name"=w1156) -> ("error out"=w1154:errorcluster, "VISA resource name out"=w1153:refnum<visa-resource-name>)  [unwired: 3 in, 1 out]
                          }
                          frame #2 {
                            n435 = To Double Precision Float(number=w1169) -> (double precision float=w1167:dbl)
                            n436 = To Double Precision Float(number=w1171) -> (double precision float=w1172:dbl)
                            n437 = Absolute Value(x=w1167) -> (abs(x)=w1168:dbl)
                            n438 = Divide(x=w1168, y=w1172) -> (x/y=w1165:dbl)
                            n439 = Multiply(x=1000.0, y=w1165) -> (x*y=w1163:dbl)
                            n440 = Add(x=w1163, y=300.0) -> (x+y=w1161:dbl)
                            n441 = To Unsigned Long Integer(number=w1161) -> (unsigned 32bit integer=w1160:u32)
                            n442 = Wait (ms)(milliseconds to wait=w1160) -> ()  [unwired: 1 out]
                          }
                          frame #3 {
                            n443 = Negate(x=w1177) -> (-x=w1178:i32)
                            n444 = Number To Decimal String(number=w1178) -> (decimal integer string=w1179:string)  [unwired: 1 in]
                            n445 = call "mDrive Send Command.vi"("error in (no error)"=w1174, "Extra"=w1179, "Command"=T10."Move to Relative Position", "VISA resource name"=w1175) -> ("error out"=w1173:errorcluster, "VISA resource name out"=w1176:refnum<visa-resource-name>)  [unwired: 3 in, 1 out]
                          }
                          frame #4 {
                            n446 = To Unsigned Long Integer(number=w1183) -> (unsigned 32bit integer=w1182:u32)
                            n447 = Wait (ms)(milliseconds to wait=w1182) -> ()  [unwired: 1 out]
                          }
                          frame #5 {
                            n448 = property on="X Backlash corr" class="Bool (strict)"("Val(Sgnl)"=FALSE ("Value (Signaling)")) -> ()  [unwired: 2 in, 2 out]
                          }
                        }
                      }
                      frame #1 {
                      }
                    }
                  }
                }
              }
              frame #1 {
                n449 = property on="STATUS" class="Str"() -> ("Value"=w1196:string)  [unwired: 2 in, 2 out]
                n450 = property on="STATUS" class="Str"() -> ("Value"=w1199:string)  [unwired: 2 in, 2 out]
                n451 = property on="Scan Go" class="Bool (strict)"() -> ("Value"=w1201:bool)  [unwired: 2 in, 2 out]
                n452 = Equal?(x=w1199, y="SCANNING MODE" ("STATUS")) -> (x = y?=w1194:bool)
                n453 = Equal?(x=w1196, y="LOOP SCANNING" ("STATUS")) -> (x = y?=w1191:bool)
                n454 = Equal?(x=w1201, y=TRUE) -> (x = y?=w1192:bool)
                n455 = Or(x=w1191, y=w1194) -> (x .or. y?=w1193:bool)
                n456 = Or(x=w1193, y=w1192) -> (x .or. y?=w1197:bool)
                n457 = case shown="False" w1197 {
                  frame #0 {
                    n458 = property on="X  in Motion" class="Bool (strict)"() -> ("Value"=w1214:bool)  [unwired: 2 in, 2 out]
                    n459 = property on="Y in Motion" class="Bool (strict)"() -> ("Value"=w1213:bool)  [unwired: 2 in, 2 out]
                    n460 = property on="Z in Motion" class="Bool (strict)"() -> ("Value"=w1216:bool)  [unwired: 2 in, 2 out]
                    n461 = property on="R in Motion" class="Bool (strict)"() -> ("Value"=w1215:bool)  [unwired: 2 in, 2 out]
                    n462 = Compound Arithmetic op=AND(w1214, w1213, w1216, w1215) -> (w1211:bool)
                    n463 = Equal?(x=w1211, y=FALSE) -> (x = y?=w1212:bool)
                    n464 = case shown="True" w1212 {
                      frame #0 {
                      }
                      frame #1 {
                        n465 = property on="Z Moved" class="Bool (strict)"() -> ("Value"=w1217:bool)  [unwired: 2 in, 2 out]
                        n466 = case shown="False" w1217 {
                          tunnel: [w1238 0 ("Value")] -> w1228
                          tunnel: [w1237 0 ("Value")] -> w1227
                          frame #0 {
                            n467 = property on="Scan Go" class="Bool (strict)"("Val(Sgnl)"=TRUE ("Value (Signaling)")) -> ()  [unwired: 2 in, 2 out]
                            n468 = property on="Y Step SP" class="DigNum (strict)"() -> ("Value"=w1238:i32)  [unwired: 2 in, 2 out]
                            n469 = property on="Y Step PV" class="DigNum (strict)"() -> ("Value"=w1237:i32)  [unwired: 2 in, 2 out]
                          }
                          frame #1 {
                          }
                        }
                        n470 = property on="X Step SP" class="DigNum (strict)"() -> ("Value"=w1230:i32)  [unwired: 2 in, 2 out]
                        n471 = property on="Z Step SP" class="DigNum (strict)"() -> ("Value"=w1226:i32)  [unwired: 2 in, 2 out]
                        n472 = property on="R Step SP" class="DigNum (strict)"() -> ("Value"=w1223:i32)  [unwired: 2 in, 2 out]
                        n473 = property on="X Step PV" class="DigNum (strict)"() -> ("Value"=w1229:i32)  [unwired: 2 in, 2 out]
                        n474 = property on="Z Step PV" class="DigNum (strict)"() -> ("Value"=w1225:i32)  [unwired: 2 in, 2 out]
                        n475 = property on="R Step PV" class="DigNum (strict)"() -> ("Value"=w1224:i32)  [unwired: 2 in, 2 out]
                        n476 = Equal?(x=w1230, y=w1229) -> (x = y?=w1234:bool)
                        n477 = Equal?(x=w1228, y=w1227) -> (x = y?=w1233:bool)
                        n478 = Equal?(x=w1226, y=w1225) -> (x = y?=w1231:bool)
                        n479 = Equal?(x=w1223, y=w1224) -> (x = y?=w1232:bool)
                        n480 = Compound Arithmetic op=AND(w1234, w1233, w1231, w1232) -> (w1218:bool)
                        n481 = property on="LoopScanConfirmed" class="Bool (strict)"() -> ("Value"=w1222:bool)  [unwired: 2 in, 2 out]
                        n482 = case shown="False" w1217 {
                          frame #0 {
                            n483 = property on="LoopCheck" class="Bool (strict)"("Val(Sgnl)"=TRUE ("Value (Signaling)")) -> ()  [unwired: 2 in, 2 out]
                          }
                          frame #1 {
                          }
                        }
                        n484 = Equal?(x=w1222, y=TRUE) -> (x = y?=w1220:bool)
                        n485 = And(x=w1218, y=w1220) -> (x .and. y?=w1219:bool)
                        n486 = case shown="True" w1219 {
                          tunnel: w1218 -> [w1241 _]
                          tunnel: w1217 -> [_ w1246]
                          frame #0 {
                            n487 = case shown="False" w1241 {
                              frame #0 {
                              }
                              frame #1 {
                                n488 = local write "STATUS"("DONE" ("STATUS")) -> ()
                                n489 = property on="GO" class="Bool"("DisabledEnum"=T1."Enabled" ("Disabled")) -> ()  [unwired: 2 in, 2 out]
                                n490 = property on="Only GO" class="Bool (strict)"("Val(Sgnl)"=FALSE ("Value (Signaling)")) -> ()  [unwired: 2 in, 2 out]
                              }
                            }
                          }
                          frame #1 {
                            n491 = flat-sequence {
                              tunnel: [w1252] -> w1248
                              tunnel: [w1251] -> w1247
                              tunnel: w1246 -> [w1249]
                              tunnel: [w1249] -> w1245
                              tunnel: w1247 -> [w1255]
                              tunnel: w1248 -> [w1256]
                              tunnel: w1245 -> [_]
                              frame #0 {
                                n492 = property on="Z Moved" class="Bool (strict)"() -> ("Value"=w1251:bool)  [unwired: 2 in, 2 out]
                                n493 = property on="FirstScan" class="Bool (strict)"() -> ("Value"=w1252:bool)  [unwired: 2 in, 2 out]
                                n494 = Or(x=w1252, y=w1251) -> (x .or. y?=w1250:bool)
                                n495 = case shown="False" w1250 {
                                tunnel: w1250 -> [_ w1253]
                                frame #0 {
                                }
                                frame #1 {
                                n496 = property on="GOBACK" class="Bool (strict)"("Val(Sgnl)"=w1253) -> ()  [unwired: 2 in, 2 out]
                                }
                                }
                              }
                              frame #1 {
                                w1259 = FALSE
                                n497 = Equal?(x=w1256, y=w1259) -> (x = y?=w1258:bool)
                                n498 = Equal?(x=w1259, y=w1255) -> (x = y?=w1257:bool)
                                n499 = And(x=w1258, y=w1257) -> (x .and. y?=w1254:bool)
                                n500 = case shown="True" w1254 {
                                tunnel: w1254 -> [_ w1260]
                                frame #0 {
                                }
                                frame #1 {
                                n501 = property on="Set for Scan" class="Bool (strict)"("Val(Sgnl)"=w1260) -> ()  [unwired: 2 in, 2 out]
                                n502 = property on="R Scan" class="Bool (strict)"("Val(Sgnl)"=w1260) -> ()  [unwired: 2 in, 2 out]
                                n503 = property on="Y Scan" class="Bool (strict)"("Val(Sgnl)"=w1260) -> ()  [unwired: 2 in, 2 out]
                                n504 = property on="X Scan" class="Bool (strict)"("Val(Sgnl)"=w1260) -> ()  [unwired: 2 in, 2 out]
                                n505 = property on="Z Scan" class="Bool (strict)"("Val(Sgnl)"=w1260) -> ()  [unwired: 2 in, 2 out]
                                }
                                }
                              }
                            }
                          }
                        }
                      }
                    }
                  }
                  frame #1 {
                    n506 = property on="LoopCheck" class="Bool (strict)"() -> ("Value"=w1262:bool)  [unwired: 2 in, 2 out]
                    n507 = case shown="False" w1262 {
                      tunnel: [w1288 TRUE] -> w1261
                      frame #0 {
                        n508 = property on="X Scan Length SP steps" class="DigNum (strict)"() -> ("Value"=w1279:i32)  [unwired: 2 in, 2 out]
                        n509 = property on="Y Scan Length SP steps" class="DigNum (strict)"() -> ("Value"=w1278:i32)  [unwired: 2 in, 2 out]
                        n510 = property on="Z Scan Length SP steps" class="DigNum (strict)"() -> ("Value"=w1277:i32)  [unwired: 2 in, 2 out]
                        n511 = property on="R Scan Length SP steps" class="DigNum (strict)"() -> ("Value"=w1276:i32)  [unwired: 2 in, 2 out]
                        n512 = property on="X Step SP" class="DigNum (strict)"() -> ("Value"=w1275:i32)  [unwired: 2 in, 2 out]
                        n513 = property on="Y Step SP" class="DigNum (strict)"() -> ("Value"=w1274:i32)  [unwired: 2 in, 2 out]
                        n514 = property on="Z Step SP" class="DigNum (strict)"() -> ("Value"=w1273:i32)  [unwired: 2 in, 2 out]
                        n515 = property on="R Step SP" class="DigNum (strict)"() -> ("Value"=w1272:i32)  [unwired: 2 in, 2 out]
                        n516 = Add(x=w1279, y=w1275) -> (x+y=w1287:i32)
                        n517 = Add(x=w1278, y=w1274) -> (x+y=w1286:i32)
                        n518 = Add(x=w1277, y=w1273) -> (x+y=w1285:i32)
                        n519 = Add(x=w1276, y=w1272) -> (x+y=w1284:i32)
                        n520 = property on="X Step PV" class="DigNum (strict)"() -> ("Value"=w1271:i32)  [unwired: 2 in, 2 out]
                        n521 = property on="Y Step PV" class="DigNum (strict)"() -> ("Value"=w1270:i32)  [unwired: 2 in, 2 out]
                        n522 = property on="Z Step PV" class="DigNum (strict)"() -> ("Value"=w1269:i32)  [unwired: 2 in, 2 out]
                        n523 = property on="R Step PV" class="DigNum (strict)"() -> ("Value"=w1268:i32)  [unwired: 2 in, 2 out]
                        n524 = Equal?(x=w1271, y=w1287) -> (x = y?=w1283:bool)
                        n525 = Equal?(x=w1270, y=w1286) -> (x = y?=w1282:bool)
                        n526 = Equal?(x=w1269, y=w1285) -> (x = y?=w1280:bool)
                        n527 = Equal?(x=w1268, y=w1284) -> (x = y?=w1281:bool)
                        n528 = Compound Arithmetic op=AND(w1283, w1282, w1280, w1281) -> (w1288:bool)
                      }
                      frame #1 {
                      }
                    }
                    n529 = property on="LoopScanConfirmed" class="Bool (strict)"() -> ("Value"=w1267:bool)  [unwired: 2 in, 2 out]
                    n530 = property on="LoopScanConfirmed" class="Bool (strict)"() -> ("Value"=w1263:bool)  [unwired: 2 in, 2 out]
                    n531 = Equal?(x=w1267, y=FALSE) -> (x = y?=w1264:bool)
                    n532 = And(x=w1264, y=w1261) -> (x .and. y?=w1265:bool)
                    n533 = case shown="False" w1265 {
                      tunnel: w1261 -> [w1291 _]
                      tunnel: w1263 -> [w1290 _]
                      frame #0 {
                        n534 = case shown="True" w1291 {
                          tunnel: w1290 -> [_ w1292]
                          frame #0 {
                          }
                          frame #1 {
                            n535 = case shown="True" w1292 {
                              frame #0 {
                                w1298 = FALSE
                                n536 = property on="Z Moved" class="Bool (strict)"() -> ("Value"=w1295:bool)  [unwired: 2 in, 2 out]
                                n537 = property on="FirstScan" class="Bool (strict)"() -> ("Value"=w1294:bool)  [unwired: 2 in, 2 out]
                                n538 = Equal?(x=w1295, y=w1298) -> (x = y?=w1297:bool)
                                n539 = Equal?(x=w1298, y=w1294) -> (x = y?=w1296:bool)
                                n540 = And(x=w1297, y=w1296) -> (x .and. y?=w1293:bool)
                                n541 = case shown="True" w1293 {
                                frame #0 {
                                }
                                frame #1 {
                                w1299 = TRUE ("Value (Signaling)")
                                n542 = property on="Loop Scan" class="Bool (strict)"("Val(Sgnl)"=w1299) -> ()  [unwired: 2 in, 2 out]
                                n543 = property on="X Scan" class="Bool (strict)"("Val(Sgnl)"=w1299) -> ()  [unwired: 2 in, 2 out]
                                n544 = property on="Y Scan" class="Bool (strict)"("Val(Sgnl)"=w1299) -> ()  [unwired: 2 in, 2 out]
                                n545 = property on="R Scan" class="Bool (strict)"("Val(Sgnl)"=w1299) -> ()  [unwired: 2 in, 2 out]
                                n546 = property on="Z Scan" class="Bool (strict)"("Val(Sgnl)"=w1299) -> ()  [unwired: 2 in, 2 out]
                                }
                                }
                              }
                              frame #1 {
                                n547 = flat-sequence {
                                tunnel: [w1311] -> w1303
                                tunnel: [w1310] -> w1302
                                tunnel: w1303 -> [w1313]
                                tunnel: [w1313] -> w1301
                                tunnel: w1302 -> [w1314]
                                tunnel: [w1314] -> w1300
                                tunnel: w1301 -> [w1324]
                                tunnel: w1300 -> [w1323]
                                frame #0 {
                                n548 = property on="LoopScanConfirmed" class="Bool (strict)"() -> ("Value"=w1306:bool)  [unwired: 2 in, 2 out]
                                n549 = property on="Scan Go" class="Bool (strict)"() -> ("Value"=w1305:bool)  [unwired: 2 in, 2 out]
                                n550 = And(x=w1306, y=w1305) -> (x .and. y?=w1304:bool)
                                n551 = case shown="True" w1304 {
                                frame #0 {
                                }
                                frame #1 {
                                n552 = property on="counter" class="DigNum (strict)"() -> ("Value"=w1308:i32)  [unwired: 2 in, 2 out]
                                n553 = Increment(x=w1308) -> (x+1=w1307:i32)
                                n554 = property on="counter" class="DigNum (strict)"("Val(Sgnl)"=w1307) -> ()  [unwired: 2 in, 2 out]
                                }
                                }
                                }
                                frame #1 {
                                n555 = property on="FirstScan" class="Bool (strict)"() -> ("Value"=w1310:bool)  [unwired: 2 in, 2 out]
                                n556 = property on="Z Moved" class="Bool (strict)"() -> ("Value"=w1311:bool)  [unwired: 2 in, 2 out]
                                n557 = Or(x=w1310, y=w1311) -> (x .or. y?=w1309:bool)
                                n558 = case shown="True" w1309 {
                                tunnel: w1309 -> [_ w1312]
                                frame #0 {
                                }
                                frame #1 {
                                n559 = property on="GOBACK" class="Bool (strict)"("Val(Sgnl)"=w1312) -> ()  [unwired: 2 in, 2 out]
                                }
                                }
                                }
                                frame #2 {
                                n560 = property on="counter" class="DigNum (strict)"() -> ("Value"=w1315:i32)  [unwired: 2 in, 2 out]
                                n561 = property on="Nr LOOPS" class="DigNum (strict)"() -> ("Value"=w1316:i32)  [unwired: 2 in, 2 out]
                                n562 = Greater Or Equal?(x=w1315, y=w1316) -> (x >= y?=w1317:bool)
                                n563 = Not(x=w1317) -> (.not. x?=w1318:bool)
                                n564 = property on="LoopScanConfirmed" class="Bool (strict)"("Val(Sgnl)"=w1318) -> ()  [unwired: 2 in, 2 out]
                                }
                                frame #3 {
                                w1322 = FALSE
                                n565 = Equal?(x=w1323, y=w1322) -> (x = y?=w1321:bool)
                                n566 = Equal?(x=w1322, y=w1324) -> (x = y?=w1320:bool)
                                n567 = And(x=w1321, y=w1320) -> (x .and. y?=w1319:bool)
                                n568 = case shown="True" w1319 {
                                selector: w1319 -> [_ w1326]
                                tunnel: w1319 -> [_ w1325]
                                frame #0 {
                                }
                                frame #1 {
                                n569 = property on="Set for Scan" class="Bool (strict)"("Val(Sgnl)"=w1325) -> ()  [unwired: 2 in, 2 out]
                                n570 = property on="Y Scan" class="Bool (strict)"("Val(Sgnl)"=w1326) -> ()  [unwired: 2 in, 2 out]
                                n571 = property on="X Scan" class="Bool (strict)"("Val(Sgnl)"=w1326) -> ()  [unwired: 2 in, 2 out]
                                n572 = property on="Z Scan" class="Bool (strict)"("Val(Sgnl)"=w1326) -> ()  [unwired: 2 in, 2 out]
                                n573 = property on="R Scan" class="Bool (strict)"("Val(Sgnl)"=w1326) -> ()  [unwired: 2 in, 2 out]
                                }
                                }
                                }
                                }
                              }
                            }
                          }
                        }
                      }
                      frame #1 {
                        n574 = property on="Set Scan \nParameters" class="Bool (strict)"("DisabledEnum"=T1."Enabled" ("Disabled")) -> ()  [unwired: 2 in, 2 out]
                        n575 = property on="GO" class="Bool"("DisabledEnum"=T1."Enabled" ("Disabled")) -> ()  [unwired: 2 in, 2 out]
                        n576 = property on="Set for Scan" class="Bool (strict)"("DisabledEnum"=T1."Enabled" ("Disabled")) -> ()  [unwired: 2 in, 2 out]
                        n577 = local write "STATUS"("DONE" ("STATUS")) -> ()
                      }
                    }
                  }
                }
              }
            }
          }
        }
        n578 = Equal?(x=w476, y=T1."Disabled and Grayed Out") -> (x = y?=w473:bool)
        n579 = Equal?(x=w479, y=T1."Enabled") -> (x = y?=w477:bool)
        n580 = And(x=w477, y=w473) -> (x .and. y?=w474:bool)
        n581 = case shown="True" w473 {
          frame #0 {
            n582 = property on="LoopScanConfirmed" class="Bool (strict)"() -> ("Value"=w521:bool)  [unwired: 2 in, 2 out]
            n583 = Equal?(x=w521, y=TRUE) -> (x = y?=w522:bool)
            n584 = case shown="False" w522 {
              frame #0 {
                n585 = local write "STATUS"("LOOP SCANNING" ("STATUS")) -> ()
              }
              frame #1 {
                n586 = local write "STATUS"("SCANNING MODE" ("STATUS")) -> ()
              }
            }
          }
          frame #1 {
          }
        }
        n587 = case shown="False" w474 {
          frame #0 {
          }
          frame #1 {
            n588 = local write "STATUS"("") -> ()
          }
        }
        n589 = property on="Z Position mm PV" class="DigNum (strict)"() -> ("Value"=w472:dbl)  [unwired: 2 in, 2 out]
        n590 = property on="R Position deg PV" class="DigNum (strict)"() -> ("Value"=w508:dbl)  [unwired: 2 in, 2 out]
        n591 = call "Build XY Graph2"("Reset"=TRUE, "Y Input"=w508, "X Input"=w472) -> ("XY Graph"=→"ZR Graph":cluster{"Y":dbl[], "Y":dbl[]}[])  [unwired: 7 in, 1 out]
        n592 = property on="Y Position mm PV" class="DigNum (strict)"() -> ("Value"=w471:dbl)  [unwired: 2 in, 2 out]
        n593 = property on="X Position mm PV" class="DigNum (strict)"() -> ("Value"=w507:dbl)  [unwired: 2 in, 2 out]
        n594 = Build Array (concatenate)(w469, w472) -> (w467:dbl[])
        n595 = Build Array (concatenate)(w468, w471) -> (w465:dbl[])
        n596 = call "Build XY Graph"("Reset"=TRUE, "Y Input"=w471, "X Input"=w507) -> ("XY Graph"=→"XY Graph":cluster{"Y":dbl[], "Y":dbl[]}[])  [unwired: 7 in, 1 out]
        n597 = Bundle(w467, w465) -> (→"ZY Graph":cluster{dbl[], dbl[]})  [unwired: 1 in]
        n598 = property on="Y Scan Length SP steps" class="DigNum (strict)"() -> ("Value"=w497:i32)  [unwired: 2 in, 2 out]
        n599 = property on="Z Scan Length SP steps" class="DigNum (strict)"() -> ("Value"=w498:i32)  [unwired: 2 in, 2 out]
        n600 = To Double Precision Float(number=w498) -> (double precision float=w491:dbl)
        n601 = To Double Precision Float(number=w497) -> (double precision float=w492:dbl)
        n602 = Divide(x=w492, y=w491) -> (x/y=w499:dbl)
        n603 = Inverse Tangent(1:w499) -> (0:w500:dbl)
        n604 = property on="Clear ZY" class="Bool (strict)"() -> ("Value"=w463:bool)  [unwired: 2 in, 2 out]
        n605 = Divide(x=w500, y=6.283185307179586) -> (x/y=w501:dbl)
        n606 = Multiply(x=360.0, y=w501) -> (x*y=w504:dbl)
        n607 = case shown="False" w463 {
          tunnel: w467 -> [w514 w519]
          tunnel: [w514 w518] -> w466
          tunnel: w465 -> [w513 w517]
          tunnel: [w513 w516] -> w464
          frame #0 {
          }
          frame #1 {
            w515 = 0 ("dimension size")
            n608 = Reshape Array(w519, w515) -> (w518:dbl[])
            n609 = Reshape Array(w517, w515) -> (w516:dbl[])
          }
        }
        n610 = property on="atan Y/Z" class="DigNum (strict)"("Val(Sgnl)"=w504) -> ()  [unwired: 2 in, 2 out]
      }
      event #1 {
        n611 = event-data() -> ()  [unwired: 1 in, 5 out]
        n612 = property on="OK Button" class="Bool (strict)"() -> ("Value"=w1331:bool)  [unwired: 2 in, 2 out]
        n613 = property on="Z Step PV" class="DigNum (strict)"() -> ("Value"=w1336:i32)  [unwired: 2 in, 2 out]
        n614 = Greater?(x=w1336, y=15360000) -> (0:w1333:bool)
        n615 = Equal?(x=w1331, y=TRUE) -> (x = y?=w1334:bool)
        n616 = And(x=w1334, y=w1333) -> (x .and. y?=w1332:bool)
        n617 = case shown="False" w1332 {
          frame #0 {
            n618 = property on="Z Step PV" class="DigNum (strict)"() -> ("Value"=w1352:i32)  [unwired: 2 in, 2 out]
            n619 = property on="OK Button" class="Bool (strict)"() -> ("Value"=w1347:bool)  [unwired: 2 in, 2 out]
            n620 = Greater?(x=w1352, y=15360000) -> (0:w1350:bool)
            n621 = Equal?(x=w1347, y=FALSE) -> (x = y?=w1349:bool)
            n622 = And(x=w1349, y=w1350) -> (x .and. y?=w1348:bool)
            n623 = case shown="True" w1348 {
              frame #0 {
              }
              frame #1 {
                n624 = One Button Dialog(message="YOU CAN'T CLOSE THE VALVE\nWHEN YOU ARE IN THE THIS\nPOSITION!!") -> (true=w1354:bool)  [unwired: 1 in]
                n625 = property on="OK Button" class="Bool (strict)"("Val(Sgnl)"=w1354) -> ()  [unwired: 2 in, 2 out]
              }
            }
          }
          frame #1 {
            n626 = flat-sequence {
              frame #0 {
                n627 = local read "OK Button"() -> (w1357:bool)
                n628 = call "DigitalIO_sub_V1_CNTL.vi"("OK Button"=w1357) -> ("Boolean"=w1356:bool)  [unwired: 2 in]
                n629 = property on="Valve \nopend/closed" class="Bool (strict)"("Val(Sgnl)"=w1356) -> ()  [unwired: 2 in, 2 out]
              }
              frame #1 {
                n630 = call "DigitalIO_sub_V1_MON.vi"() -> ("CL"=w1359:bool, "OP"=w1358:bool)  [unwired: 8 in]
                n631 = property on="OP" class="Bool (strict)"("Val(Sgnl)"=w1358) -> ()  [unwired: 2 in, 2 out]
                n632 = property on="CL" class="Bool (strict)"("Val(Sgnl)"=w1359) -> ()  [unwired: 2 in, 2 out]
              }
              frame #2 {
                n633 = Wait (ms)(milliseconds to wait=u32 100) -> ()  [unwired: 1 out]
              }
            }
          }
        }
        n634 = local write "STATUS"("VALVE CHANGED" ("STATUS")) -> ()
      }
      event #2 {
        n635 = event-data() -> ()  [unwired: 1 in, 7 out]
        n636 = property on="X Position mm PV" class="DigNum (strict)"() -> ("Value"=w1374:dbl)  [unwired: 2 in, 2 out]
        n637 = property on="X Position SP mm" class="DigNum (strict)"() -> ("Value"=w1373:dbl)  [unwired: 2 in, 2 out]
        n638 = property on="Z Position mm PV" class="DigNum (strict)"() -> ("Value"=w1370:dbl)  [unwired: 2 in, 2 out]
        n639 = property on="Z Position SP mm" class="DigNum (strict)"() -> ("Value"=w1362:dbl)  [unwired: 2 in, 2 out]
        n640 = property on="R Position SP deg" class="DigNum (strict)"() -> ("Value"=w1365:dbl)  [unwired: 2 in, 2 out]
        n641 = property on="R Position deg PV" class="DigNum (strict)"() -> ("Value"=w1364:dbl)  [unwired: 2 in, 2 out]
        n642 = property on="Y Position mm PV" class="DigNum (strict)"() -> ("Value"=w1368:dbl)  [unwired: 2 in, 2 out]
        n643 = property on="Y Position SP mm" class="DigNum (strict)"() -> ("Value"=w1367:dbl)  [unwired: 2 in, 2 out]
        n644 = Not Equal?(x=w1374, y=w1373) -> (x != y?=w1372:bool)
        n645 = Not Equal?(x=w1370, y=w1362) -> (x != y?=w1371:bool)
        n646 = Not Equal?(x=w1368, y=w1367) -> (x != y?=w1369:bool)
        n647 = Not Equal?(x=w1365, y=w1364) -> (x != y?=w1366:bool)
        n648 = case shown="True" w1371 {
          tunnel: w1387 -> [w1532 w1539]
          tunnel: w1386 -> [w1533 w1538]
          tunnel: [w1533 w1537] -> w1385
          tunnel: [w1532 w1536] -> w1384
          frame #0 {
          }
          frame #1 {
            n649 = flat-sequence {
              tunnel: w1538 -> [w1561]
              tunnel: w1539 -> [w1562]
              tunnel: [w1562] -> w1535
              tunnel: [w1561] -> w1534
              tunnel: [w1577] -> w1553
              tunnel: [w1576] -> w1552
              tunnel: [w1564] -> w1551
              tunnel: w1535 -> [w1577]
              tunnel: w1534 -> [w1576]
              tunnel: [w1580] -> w1550
              tunnel: [w1579] -> w1549
              tunnel: [w1578] -> w1548
              tunnel: w1551 -> [w1578]
              tunnel: w1552 -> [w1579]
              tunnel: w1553 -> [w1580]
              tunnel: [w1596] -> w1547
              tunnel: [w1595] -> w1546
              tunnel: w1550 -> [w1594]
              tunnel: w1549 -> [w1593]
              tunnel: [w1592] -> w1545
              tunnel: w1548 -> [w1592]
              tunnel: w1547 -> [w1603]
              tunnel: [w1603] -> w1544
              tunnel: w1546 -> [w1602]
              tunnel: [w1602] -> w1543
              tunnel: w1545 -> [w1601]
              tunnel: [w1601] -> w1542
              tunnel: [w1608] -> w1541
              tunnel: [w1607] -> w1540
              tunnel: w1544 -> [w1606]
              tunnel: w1543 -> [w1605]
              tunnel: w1542 -> [w1604]
              tunnel: [w1612] -> w1536
              tunnel: [w1613] -> w1537
              tunnel: w1541 -> [w1613]
              tunnel: w1540 -> [w1612]
              frame #0 {
                n650 = property on="Z Position SP mm" class="DigNum (strict)"() -> ("Value"=w1556:dbl)  [unwired: 2 in, 2 out]
                n651 = property on="Z Position mm PV" class="DigNum (strict)"() -> ("Value"=w1554:dbl)  [unwired: 2 in, 2 out]
                n652 = Greater?(x=w1556, y=60.0) -> (0:w1559:bool)
                n653 = Less?(x=w1554, y=60.0) -> (x < y?=w1558:bool)
                n654 = And(x=w1558, y=w1559) -> (x .and. y?=w1560:bool)
                n655 = case shown="True" w1560 {
                  frame #0 {
                  }
                  frame #1 {
                    n656 = property on="Z Position SP mm" class="DigNum (strict)"("Val(Sgnl)"=60.0 ("Value (Signaling)")) -> ()  [unwired: 2 in, 2 out]
                  }
                }
              }
              frame #1 {
                n657 = property on="Z Position SP mm" class="DigNum (strict)"() -> ("Value"=w1570:dbl)  [unwired: 2 in, 2 out]
                n658 = property on="Z offset mm" class="DigNum (strict)"() -> ("Value"=w1571:dbl)  [unwired: 2 in, 2 out]
                n659 = property on="Z mm/rev" class="DigNum (strict)"() -> ("Value"=w1572:dbl)  [unwired: 2 in, 2 out]
                n660 = property on="Z steps/rev" class="DigNum (strict)"() -> ("Value"=w1573:u32)  [unwired: 2 in, 2 out]
                n661 = To Double Precision Float(number=w1573) -> (double precision float=w1569:dbl)
                n662 = Subtract(x=w1570, y=w1571) -> (x-y=w1566:dbl)
                n663 = Divide(x=w1566, y=w1572) -> (x/y=w1565:dbl)
                n664 = property on="Z Step SP" class="DigNum (strict)"() -> ("Maximum"=w1575:dbl)  [unwired: 2 in, 2 out]
                n665 = property on="Z Step SP" class="DigNum (strict)"() -> ("Minimum"=w1574:dbl)  [unwired: 2 in, 2 out]
                n666 = Multiply(x=w1565, y=w1569) -> (x*y=w1567:dbl)
                n667 = In Range and Coerce(upper limit=w1575, x=w1567, lower limit=w1574) -> (coerced(x)=w1568:dbl)  [unwired: 1 out]
                n668 = To Long Integer(number=w1568) -> (32bit integer=w1564:i32)
                n669 = property on="Z Step SP" class="DigNum (strict)"("Val(Sgnl)"=w1564) -> ()  [unwired: 2 in, 2 out]
              }
              frame #2 {
                n670 = property on="Z Step SP" class="DigNum (strict)"() -> ("Value"=w1589:i32)  [unwired: 2 in, 2 out]
                n671 = property on="Z Step PV" class="DigNum (strict)"() -> ("Value"=w1588:i32)  [unwired: 2 in, 2 out]
                n672 = property on="Z Backlash" class="DigNum (strict)"() -> ("Value"=w1581:i32)  [unwired: 2 in, 2 out]
                n673 = Subtract(x=w1589, y=w1588) -> (x-y=w1587:i32)
                n674 = Sign(1:w1581) -> (0:w1585:i32)
                n675 = Sign(1:w1587) -> (0:w1586:i32)
                n676 = Multiply(x=w1586, y=w1585) -> (x*y=w1584:i32)
                n677 = Equal?(x=w1584, y=1) -> (x = y?=w1582:bool)
                n678 = case shown="False" w1582 {
                  frame #0 {
                    n679 = property on="Z Backlash corr" class="Bool (strict)"("Val(Sgnl)"=FALSE ("Value (Signaling)")) -> ()  [unwired: 2 in, 2 out]
                  }
                  frame #1 {
                    n680 = property on="Z Backlash corr" class="Bool (strict)"("Val(Sgnl)"=TRUE ("Value (Signaling)")) -> ()  [unwired: 2 in, 2 out]
                  }
                }
              }
              frame #3 {
                # "Velocity Setting"
                n681 = property on="Z Velocity SP step/sec" class="DigNum (strict)"() -> ("Value"=w1597:i32)  [unwired: 2 in, 2 out]
                n682 = Number To Decimal String(number=w1597) -> (decimal integer string=w1598:string)  [unwired: 1 in]
                n683 = call "mDrive Send Command.vi"("error in (no error)"=w1594, "Extra"=w1598, "Command"=T10."Max Velocity", "VISA resource name"=w1593) -> ("error out"=w1595:errorcluster, "VISA resource name out"=w1596:refnum<visa-resource-name>)  [unwired: 3 in, 1 out]
              }
              frame #4 {
                n684 = Wait (ms)(milliseconds to wait=u32 50) -> ()  [unwired: 1 out]
              }
              frame #5 {
                # "Move to Abs Position"
                n685 = Number To Decimal String(number=w1604) -> (decimal integer string=w1610:string)  [unwired: 1 in]
                n686 = call "mDrive Send Command.vi"("error in (no error)"=w1605, "Extra"=w1610, "Command"=T10."Move to Absolute Position", "VISA resource name"=w1606) -> ("error out"=w1607:errorcluster, "VISA resource name out"=w1608:refnum<visa-resource-name>)  [unwired: 3 in, 1 out]
              }
              frame #6 {
                n687 = Wait (ms)(milliseconds to wait=u32 50) -> ()  [unwired: 1 out]
              }
            }
          }
        }
        n688 = case shown="True" w1372 {
          tunnel: w1391 -> [w1615 w1619]
          tunnel: w1390 -> [w1614 w1618]
          tunnel: [w1615 w1617] -> w1389
          tunnel: [w1614 w1616] -> w1388
          frame #0 {
          }
          frame #1 {
            n689 = flat-sequence {
              tunnel: w1618 -> [w1646]
              tunnel: w1619 -> [w1647]
              tunnel: [w1647] -> w1633
              tunnel: [w1646] -> w1632
              tunnel: [w1635] -> w1631
              tunnel: [w1650] -> w1630
              tunnel: [w1649] -> w1629
              tunnel: [w1648] -> w1628
              tunnel: w1631 -> [w1648]
              tunnel: w1632 -> [w1649]
              tunnel: w1633 -> [w1650]
              tunnel: [w1666] -> w1627
              tunnel: [w1665] -> w1626
              tunnel: w1630 -> [w1664]
              tunnel: w1629 -> [w1663]
              tunnel: w1628 -> [w1662]
              tunnel: [w1662] -> w1625
              tunnel: w1627 -> [w1673]
              tunnel: [w1673] -> w1624
              tunnel: w1626 -> [w1672]
              tunnel: [w1672] -> w1623
              tunnel: [w1670] -> w1622
              tunnel: w1625 -> [w1670]
              tunnel: [w1678] -> w1621
              tunnel: [w1677] -> w1620
              tunnel: w1624 -> [w1676]
              tunnel: w1623 -> [w1675]
              tunnel: w1622 -> [w1674]
              tunnel: [w1682] -> w1616
              tunnel: [w1683] -> w1617
              tunnel: w1621 -> [w1683]
              tunnel: w1620 -> [w1682]
              frame #0 {
                n690 = property on="X Position SP mm" class="DigNum (strict)"() -> ("Value"=w1643:dbl)  [unwired: 2 in, 2 out]
                n691 = property on="X offset mm" class="DigNum (strict)"() -> ("Value"=w1644:dbl)  [unwired: 2 in, 2 out]
                n692 = property on="X mm/rev" class="DigNum (strict)"() -> ("Value"=w1634:dbl)  [unwired: 2 in, 2 out]
                n693 = property on="X steps/rev" class="DigNum (strict)"() -> ("Value"=w1645:u32)  [unwired: 2 in, 2 out]
                n694 = To Double Precision Float(number=w1645) -> (double precision float=w1640:dbl)
                n695 = Subtract(x=w1643, y=w1644) -> (x-y=w1637:dbl)
                n696 = Divide(x=w1637, y=w1634) -> (x/y=w1636:dbl)
                n697 = Multiply(x=w1636, y=w1640) -> (x*y=w1638:dbl)
                n698 = property on="X Step SP" class="DigNum (strict)"() -> ("Maximum"=w1642:dbl)  [unwired: 2 in, 2 out]
                n699 = property on="X Step SP" class="DigNum (strict)"() -> ("Minimum"=w1641:dbl)  [unwired: 2 in, 2 out]
                n700 = In Range and Coerce(upper limit=w1642, x=w1638, lower limit=w1641) -> (coerced(x)=w1639:dbl)  [unwired: 1 out]
                n701 = To Long Integer(number=w1639) -> (32bit integer=w1635:i32)
                n702 = property on="X Step SP" class="DigNum (strict)"("Val(Sgnl)"=w1635) -> ()  [unwired: 2 in, 2 out]
              }
              frame #1 {
                n703 = property on="X Step SP" class="DigNum (strict)"() -> ("Value"=w1659:i32)  [unwired: 2 in, 2 out]
                n704 = property on="X Step PV" class="DigNum (strict)"() -> ("Value"=w1658:i32)  [unwired: 2 in, 2 out]
                n705 = property on="X Backlash" class="DigNum (strict)"() -> ("Value"=w1651:i32)  [unwired: 2 in, 2 out]
                n706 = Sign(1:w1651) -> (0:w1655:i32)
                n707 = Subtract(x=w1659, y=w1658) -> (x-y=w1657:i32)
                n708 = Sign(1:w1657) -> (0:w1656:i32)
                n709 = Multiply(x=w1656, y=w1655) -> (x*y=w1654:i32)
                n710 = Equal?(x=w1654, y=1) -> (x = y?=w1652:bool)
                n711 = case shown="False" w1652 {
                  frame #0 {
                    n712 = property on="X Backlash corr" class="Bool (strict)"("Val(Sgnl)"=FALSE ("Value (Signaling)")) -> ()  [unwired: 2 in, 2 out]
                  }
                  frame #1 {
                    n713 = property on="X Backlash corr" class="Bool (strict)"("Val(Sgnl)"=TRUE ("Value (Signaling)")) -> ()  [unwired: 2 in, 2 out]
                  }
                }
              }
              frame #2 {
                # "Velocity Setting"
                n714 = property on="X Velocity SP step/sec" class="DigNum (strict)"() -> ("Value"=w1667:i32)  [unwired: 2 in, 2 out]
                n715 = Number To Decimal String(number=w1667) -> (decimal integer string=w1668:string)  [unwired: 1 in]
                n716 = call "mDrive Send Command.vi"("error in (no error)"=w1663, "Extra"=w1668, "Command"=T10."Max Velocity", "VISA resource name"=w1664) -> ("error out"=w1665:errorcluster, "VISA resource name out"=w1666:refnum<visa-resource-name>)  [unwired: 3 in, 1 out]
              }
              frame #3 {
                n717 = Wait (ms)(milliseconds to wait=u32 50) -> ()  [unwired: 1 out]
              }
              frame #4 {
                # "Move to Abs Position"
                n718 = Number To Decimal String(number=w1674) -> (decimal integer string=w1680:string)  [unwired: 1 in]
                n719 = call "mDrive Send Command.vi"("error in (no error)"=w1675, "Extra"=w1680, "Command"=T10."Move to Absolute Position", "VISA resource name"=w1676) -> ("error out"=w1677:errorcluster, "VISA resource name out"=w1678:refnum<visa-resource-name>)  [unwired: 3 in, 1 out]
              }
              frame #5 {
                n720 = Wait (ms)(milliseconds to wait=u32 50) -> ()  [unwired: 1 out]
              }
            }
          }
        }
        n721 = case shown="True" w1369 {
          tunnel: w1383 -> [w1462 w1467]
          tunnel: w1382 -> [w1463 w1466]
          tunnel: [w1463 w1465] -> w1381
          tunnel: [w1462 w1464] -> w1380
          frame #0 {
          }
          frame #1 {
            n722 = flat-sequence {
              tunnel: [w1495] -> w1481
              tunnel: [w1494] -> w1480
              tunnel: [w1482] -> w1479
              tunnel: w1466 -> [w1494]
              tunnel: w1467 -> [w1495]
              tunnel: [w1498] -> w1478
              tunnel: [w1497] -> w1477
              tunnel: [w1496] -> w1476
              tunnel: w1479 -> [w1496]
              tunnel: w1480 -> [w1497]
              tunnel: w1481 -> [w1498]
              tunnel: [w1514] -> w1475
              tunnel: [w1513] -> w1474
              tunnel: w1478 -> [w1512]
              tunnel: w1477 -> [w1511]
              tunnel: [w1510] -> w1473
              tunnel: w1476 -> [w1510]
              tunnel: w1475 -> [w1521]
              tunnel: [w1521] -> w1472
              tunnel: w1474 -> [w1520]
              tunnel: [w1520] -> w1471
              tunnel: [w1518] -> w1470
              tunnel: w1473 -> [w1518]
              tunnel: [w1526] -> w1469
              tunnel: [w1525] -> w1468
              tunnel: w1472 -> [w1524]
              tunnel: w1471 -> [w1523]
              tunnel: w1470 -> [w1522]
              tunnel: [w1529] -> w1464
              tunnel: [w1531] -> w1465
              tunnel: w1469 -> [w1531]
              tunnel: w1468 -> [w1529]
              frame #0 {
                n723 = property on="Y Position SP mm" class="DigNum (strict)"() -> ("Value"=w1488:dbl)  [unwired: 2 in, 2 out]
                n724 = property on="Y offset mm" class="DigNum (strict)"() -> ("Value"=w1489:dbl)  [unwired: 2 in, 2 out]
                n725 = property on="Y mm/rev" class="DigNum (strict)"() -> ("Value"=w1490:dbl)  [unwired: 2 in, 2 out]
                n726 = property on="Y steps/rev" class="DigNum (strict)"() -> ("Value"=w1491:u32)  [unwired: 2 in, 2 out]
                n727 = To Double Precision Float(number=w1491) -> (double precision float=w1487:dbl)
                n728 = Subtract(x=w1488, y=w1489) -> (x-y=w1484:dbl)
                n729 = Divide(x=w1484, y=w1490) -> (x/y=w1483:dbl)
                n730 = Multiply(x=w1483, y=w1487) -> (x*y=w1485:dbl)
                n731 = property on="Y Step SP" class="DigNum (strict)"() -> ("Maximum"=w1492:dbl)  [unwired: 2 in, 2 out]
                n732 = property on="Y Step SP" class="DigNum (strict)"() -> ("Minimum"=w1493:dbl)  [unwired: 2 in, 2 out]
                n733 = In Range and Coerce(upper limit=w1492, x=w1485, lower limit=w1493) -> (coerced(x)=w1486:dbl)  [unwired: 1 out]
                n734 = To Long Integer(number=w1486) -> (32bit integer=w1482:i32)
                n735 = property on="Y Step SP" class="DigNum (strict)"("Val(Sgnl)"=w1482) -> ()  [unwired: 2 in, 2 out]
              }
              frame #1 {
                n736 = property on="Y Step SP" class="DigNum (strict)"() -> ("Value"=w1507:i32)  [unwired: 2 in, 2 out]
                n737 = property on="Y Step PV" class="DigNum (strict)"() -> ("Value"=w1506:i32)  [unwired: 2 in, 2 out]
                n738 = property on="Y Backlash" class="DigNum (strict)"() -> ("Value"=w1499:i32)  [unwired: 2 in, 2 out]
                n739 = Subtract(x=w1507, y=w1506) -> (x-y=w1505:i32)
                n740 = Sign(1:w1499) -> (0:w1503:i32)
                n741 = Sign(1:w1505) -> (0:w1504:i32)
                n742 = Multiply(x=w1504, y=w1503) -> (x*y=w1502:i32)
                n743 = Equal?(x=w1502, y=1) -> (x = y?=w1500:bool)
                n744 = case shown="False" w1500 {
                  frame #0 {
                    n745 = property on="Y Backlash corr" class="Bool (strict)"("Val(Sgnl)"=FALSE ("Value (Signaling)")) -> ()  [unwired: 2 in, 2 out]
                  }
                  frame #1 {
                    n746 = property on="Y Backlash corr" class="Bool (strict)"("Val(Sgnl)"=TRUE ("Value (Signaling)")) -> ()  [unwired: 2 in, 2 out]
                  }
                }
              }
              frame #2 {
                # "Velocity Setting"
                n747 = property on="Y Velocity SP step/sec" class="DigNum (strict)"() -> ("Value"=w1515:i32)  [unwired: 2 in, 2 out]
                n748 = Number To Decimal String(number=w1515) -> (decimal integer string=w1516:string)  [unwired: 1 in]
                n749 = call "mDrive Send Command.vi"("error in (no error)"=w1512, "Extra"=w1516, "Command"=T10."Max Velocity", "VISA resource name"=w1511) -> ("error out"=w1513:errorcluster, "VISA resource name out"=w1514:refnum<visa-resource-name>)  [unwired: 3 in, 1 out]
              }
              frame #3 {
                n750 = Wait (ms)(milliseconds to wait=u32 50) -> ()  [unwired: 1 out]
              }
              frame #4 {
                # "Move to Abs Position"
                n751 = Number To Decimal String(number=w1522) -> (decimal integer string=w1528:string)  [unwired: 1 in]
                n752 = call "mDrive Send Command.vi"("error in (no error)"=w1523, "Extra"=w1528, "Command"=T10."Move to Absolute Position", "VISA resource name"=w1524) -> ("error out"=w1525:errorcluster, "VISA resource name out"=w1526:refnum<visa-resource-name>)  [unwired: 3 in, 1 out]
              }
              frame #5 {
                n753 = Wait (ms)(milliseconds to wait=u32 25) -> ()  [unwired: 1 out]
              }
            }
          }
        }
        n754 = case shown="True" w1366 {
          tunnel: w1379 -> [w1392 w1397]
          tunnel: w1378 -> [w1393 w1396]
          tunnel: [w1393 w1395] -> w1377
          tunnel: [w1392 w1394] -> w1376
          frame #0 {
          }
          frame #1 {
            n755 = flat-sequence {
              tunnel: w1396 -> [w1424]
              tunnel: w1397 -> [w1425]
              tunnel: [w1425] -> w1411
              tunnel: [w1424] -> w1410
              tunnel: [w1412] -> w1409
              tunnel: [w1428] -> w1408
              tunnel: [w1427] -> w1407
              tunnel: [w1426] -> w1406
              tunnel: w1409 -> [w1426]
              tunnel: w1410 -> [w1427]
              tunnel: w1411 -> [w1428]
              tunnel: [w1444] -> w1405
              tunnel: [w1443] -> w1404
              tunnel: w1408 -> [w1442]
              tunnel: w1407 -> [w1441]
              tunnel: [w1440] -> w1403
              tunnel: w1406 -> [w1440]
              tunnel: w1405 -> [w1451]
              tunnel: [w1451] -> w1402
              tunnel: w1404 -> [w1450]
              tunnel: [w1450] -> w1401
              tunnel: w1403 -> [w1449]
              tunnel: [w1449] -> w1400
              tunnel: [w1456] -> w1399
              tunnel: [w1455] -> w1398
              tunnel: w1402 -> [w1454]
              tunnel: w1401 -> [w1453]
              tunnel: w1400 -> [w1452]
              tunnel: [w1461] -> w1395
              tunnel: w1399 -> [w1461]
              tunnel: w1398 -> [w1460]
              tunnel: [w1460] -> w1394
              frame #0 {
                n756 = property on="R Position SP deg" class="DigNum (strict)"() -> ("Value"=w1422:dbl)  [unwired: 2 in, 2 out]
                n757 = property on="R offset deg" class="DigNum (strict)"() -> ("Value"=w1421:dbl)  [unwired: 2 in, 2 out]
                n758 = property on="R deg/rev" class="DigNum (strict)"() -> ("Value"=w1423:dbl)  [unwired: 2 in, 2 out]
                n759 = property on="R steps/rev" class="DigNum (strict)"() -> ("Value"=w1420:u32)  [unwired: 2 in, 2 out]
                n760 = To Double Precision Float(number=w1420) -> (double precision float=w1417:dbl)
                n761 = Subtract(x=w1422, y=w1421) -> (x-y=w1414:dbl)
                n762 = Divide(x=w1414, y=w1423) -> (x/y=w1413:dbl)
                n763 = Multiply(x=w1413, y=w1417) -> (x*y=w1415:dbl)
                n764 = property on="R Step SP" class="DigNum (strict)"() -> ("Maximum"=w1418:dbl)  [unwired: 2 in, 2 out]
                n765 = property on="R Step SP" class="DigNum (strict)"() -> ("Minimum"=w1419:dbl)  [unwired: 2 in, 2 out]
                n766 = In Range and Coerce(upper limit=w1418, x=w1415, lower limit=w1419) -> (coerced(x)=w1416:dbl)  [unwired: 1 out]
                n767 = To Long Integer(number=w1416) -> (32bit integer=w1412:i32)
                n768 = property on="R Step SP" class="DigNum (strict)"("Val(Sgnl)"=w1412) -> ()  [unwired: 2 in, 2 out]
              }
              frame #1 {
                n769 = property on="R Step SP" class="DigNum (strict)"() -> ("Value"=w1437:i32)  [unwired: 2 in, 2 out]
                n770 = property on="R Step PV" class="DigNum (strict)"() -> ("Value"=w1436:i32)  [unwired: 2 in, 2 out]
                n771 = property on="R Backlash" class="DigNum (strict)"() -> ("Value"=w1429:i32)  [unwired: 2 in, 2 out]
                n772 = Subtract(x=w1437, y=w1436) -> (x-y=w1435:i32)
                n773 = Sign(1:w1429) -> (0:w1433:i32)
                n774 = Sign(1:w1435) -> (0:w1434:i32)
                n775 = Multiply(x=w1434, y=w1433) -> (x*y=w1432:i32)
                n776 = Equal?(x=w1432, y=1) -> (x = y?=w1430:bool)
                n777 = case shown="False" w1430 {
                  frame #0 {
                    n778 = property on="R Backlash corr" class="Bool (strict)"("Val(Sgnl)"=FALSE ("Value (Signaling)")) -> ()  [unwired: 2 in, 2 out]
                  }
                  frame #1 {
                    n779 = property on="R Backlash corr" class="Bool (strict)"("Val(Sgnl)"=TRUE ("Value (Signaling)")) -> ()  [unwired: 2 in, 2 out]
                  }
                }
              }
              frame #2 {
                # "Velocity Setting"
                n780 = property on="R Velocity SP step/sec" class="DigNum (strict)"() -> ("Value"=w1445:i32)  [unwired: 2 in, 2 out]
                n781 = Number To Decimal String(number=w1445) -> (decimal integer string=w1446:string)  [unwired: 1 in]
                n782 = call "mDrive Send Command.vi"("error in (no error)"=w1442, "Extra"=w1446, "Command"=T10."Max Velocity", "VISA resource name"=w1441) -> ("error out"=w1443:errorcluster, "VISA resource name out"=w1444:refnum<visa-resource-name>)  [unwired: 3 in, 1 out]
              }
              frame #3 {
                n783 = Wait (ms)(milliseconds to wait=u32 50) -> ()  [unwired: 1 out]
              }
              frame #4 {
                # "Move to Abs Position"
                n784 = Number To Decimal String(number=w1452) -> (decimal integer string=w1458:string)  [unwired: 1 in]
                n785 = call "mDrive Send Command.vi"("error in (no error)"=w1453, "Extra"=w1458, "Command"=T10."Move to Absolute Position", "VISA resource name"=w1454) -> ("error out"=w1455:errorcluster, "VISA resource name out"=w1456:refnum<visa-resource-name>)  [unwired: 3 in, 1 out]
              }
              frame #5 {
                n786 = Wait (ms)(milliseconds to wait=u32 25) -> ()  [unwired: 1 out]
              }
            }
          }
        }
        n787 = property on="GO" class="Bool"("DisabledEnum"=T1."Disabled and Grayed Out" ("Disabled")) -> ()  [unwired: 2 in, 2 out]
        n788 = local write "STATUS"("MOVING" ("STATUS")) -> ()
        n789 = property on="Z Moved" class="Bool (strict)"("Val(Sgnl)"=FALSE ("Value (Signaling)")) -> ()  [unwired: 2 in, 2 out]
      }
      event #3 {
        n790 = event-data() -> ()  [unwired: 1 in, 5 out]
        n791 = property on="Y Position mm PV" class="DigNum (strict)"() -> ("Value"=w1691:dbl)  [unwired: 2 in, 2 out]
        n792 = property on="Y Position SP mm" class="DigNum (strict)"() -> ("Value"=w1694:dbl)  [unwired: 2 in, 2 out]
        n793 = property on="Z Moved" class="Bool (strict)"() -> ("Value"=w1686:bool)  [unwired: 2 in, 2 out]
        n794 = property on="X Position mm PV" class="DigNum (strict)"() -> ("Value"=w1689:dbl)  [unwired: 2 in, 2 out]
        n795 = property on="X Position SP mm" class="DigNum (strict)"() -> ("Value"=w1696:dbl)  [unwired: 2 in, 2 out]
        n796 = property on="Z Position mm PV" class="DigNum (strict)"() -> ("Value"=w1690:dbl)  [unwired: 2 in, 2 out]
        n797 = property on="Z Position SP mm" class="DigNum (strict)"() -> ("Value"=w1695:dbl)  [unwired: 2 in, 2 out]
        n798 = property on="R Position deg PV" class="DigNum (strict)"() -> ("Value"=w1692:dbl)  [unwired: 2 in, 2 out]
        n799 = property on="R Position SP deg" class="DigNum (strict)"() -> ("Value"=w1693:dbl)  [unwired: 2 in, 2 out]
        n800 = Equal?(x=w1686, y=TRUE) -> (x = y?=w1684:bool)
        n801 = Not Equal?(x=w1691, y=w1694) -> (x != y?=w1687:bool)
        n802 = Not Equal?(x=w1689, y=w1696) -> (x != y?=w1717:bool)
        n803 = Not Equal?(x=w1690, y=w1695) -> (x != y?=w1716:bool)
        n804 = Not Equal?(x=w1692, y=w1693) -> (x != y?=w1715:bool)
        n805 = And(x=w1687, y=w1684) -> (x .and. y?=w1688:bool)
        n806 = case shown="True" w1716 {
          tunnel: w1712 -> [w1866 w1876]
          tunnel: w1711 -> [w1867 w1875]
          tunnel: [w1867 w1874] -> w1704
          tunnel: [w1866 w1873] -> w1703
          frame #0 {
          }
          frame #1 {
            n807 = flat-sequence {
              tunnel: [w1904] -> w1890
              tunnel: [w1903] -> w1889
              tunnel: [w1891] -> w1888
              tunnel: w1876 -> [w1904]
              tunnel: w1875 -> [w1903]
              tunnel: [w1891] -> w1872
              tunnel: [w1910] -> w1887
              tunnel: [w1909] -> w1886
              tunnel: [w1908] -> w1885
              tunnel: w1888 -> [w1908]
              tunnel: w1889 -> [w1909]
              tunnel: w1890 -> [w1910]
              tunnel: w1872 -> [w1907]
              tunnel: [w1924] -> w1884
              tunnel: [w1923] -> w1883
              tunnel: w1887 -> [w1922]
              tunnel: w1886 -> [w1921]
              tunnel: [w1920] -> w1882
              tunnel: w1885 -> [w1920]
              tunnel: w1884 -> [w1930]
              tunnel: [w1930] -> w1881
              tunnel: w1883 -> [w1929]
              tunnel: [w1929] -> w1880
              tunnel: w1882 -> [w1928]
              tunnel: [w1928] -> w1879
              tunnel: [w1935] -> w1878
              tunnel: [w1934] -> w1877
              tunnel: w1881 -> [w1933]
              tunnel: w1880 -> [w1932]
              tunnel: w1879 -> [w1931]
              tunnel: w1878 -> [w1940]
              tunnel: w1877 -> [w1939]
              tunnel: [w1940] -> w1871
              tunnel: [w1939] -> w1870
              tunnel: w1871 -> [w1945]
              tunnel: w1870 -> [w1944]
              tunnel: [w1945] -> w1869
              tunnel: [w1944] -> w1868
              tunnel: [w1947] -> w1873
              tunnel: [w1948] -> w1874
              tunnel: w1869 -> [w1948]
              tunnel: w1868 -> [w1947]
              frame #0 {
                n808 = property on="Z Position SP mm" class="DigNum (strict)"() -> ("Value"=w1897:dbl)  [unwired: 2 in, 2 out]
                n809 = property on="Z offset mm" class="DigNum (strict)"() -> ("Value"=w1894:dbl)  [unwired: 2 in, 2 out]
                n810 = property on="Z mm/rev" class="DigNum (strict)"() -> ("Value"=w1893:dbl)  [unwired: 2 in, 2 out]
                n811 = property on="Z steps/rev" class="DigNum (strict)"() -> ("Value"=w1892:u32)  [unwired: 2 in, 2 out]
                n812 = To Double Precision Float(number=w1892) -> (double precision float=w1902:dbl)
                n813 = Subtract(x=w1897, y=w1894) -> (x-y=w1899:dbl)
                n814 = Divide(x=w1899, y=w1893) -> (x/y=w1898:dbl)
                n815 = property on="Z Step SP" class="DigNum (strict)"() -> ("Maximum"=w1896:dbl)  [unwired: 2 in, 2 out]
                n816 = property on="Z Step SP" class="DigNum (strict)"() -> ("Minimum"=w1895:dbl)  [unwired: 2 in, 2 out]
                n817 = Multiply(x=w1898, y=w1902) -> (x*y=w1900:dbl)
                n818 = In Range and Coerce(upper limit=w1896, x=w1900, lower limit=w1895) -> (coerced(x)=w1901:dbl)  [unwired: 1 out]
                n819 = To Long Integer(number=w1901) -> (32bit integer=w1891:i32)
              }
              frame #1 {
                n820 = property on="Z Backlash" class="DigNum (strict)"() -> ("Value"=w1906:i32)  [unwired: 2 in, 2 out]
                n821 = property on="Z Step PV" class="DigNum (strict)"() -> ("Value"=w1905:i32)  [unwired: 2 in, 2 out]
                n822 = Subtract(x=w1907, y=w1905) -> (x-y=w1916:i32)
                n823 = Sign(1:w1906) -> (0:w1914:i32)
                n824 = Sign(1:w1916) -> (0:w1915:i32)
                n825 = Multiply(x=w1915, y=w1914) -> (x*y=w1913:i32)
                n826 = Equal?(x=w1913, y=1) -> (x = y?=w1911:bool)
                n827 = case shown="True" w1911 {
                  frame #0 {
                    n828 = property on="Z Backlash corr" class="Bool (strict)"("Val(Sgnl)"=FALSE ("Value (Signaling)")) -> ()  [unwired: 2 in, 2 out]
                  }
                  frame #1 {
                    n829 = property on="Z Backlash corr" class="Bool (strict)"("Val(Sgnl)"=TRUE ("Value (Signaling)")) -> ()  [unwired: 2 in, 2 out]
                  }
                }
              }
              frame #2 {
                # "Velocity Setting"
                n830 = property on="Z Velocity SP step/sec" class="DigNum (strict)"() -> ("Value"=w1919:i32)  [unwired: 2 in, 2 out]
                n831 = Number To Decimal String(number=w1919) -> (decimal integer string=w1925:string)  [unwired: 1 in]
                n832 = call "mDrive Send Command.vi"("error in (no error)"=w1922, "Extra"=w1925, "Command"=T10."Max Velocity", "VISA resource name"=w1921) -> ("error out"=w1923:errorcluster, "VISA resource name out"=w1924:refnum<visa-resource-name>)  [unwired: 3 in, 1 out]
              }
              frame #3 {
                n833 = Wait (ms)(milliseconds to wait=u32 50) -> ()  [unwired: 1 out]
              }
              frame #4 {
                # "Move to Abs Position"
                n834 = Number To Decimal String(number=w1931) -> (decimal integer string=w1937:string)  [unwired: 1 in]
                n835 = call "mDrive Send Command.vi"("error in (no error)"=w1932, "Extra"=w1937, "Command"=T10."Move to Absolute Position", "VISA resource name"=w1933) -> ("error out"=w1934:errorcluster, "VISA resource name out"=w1935:refnum<visa-resource-name>)  [unwired: 3 in, 1 out]
              }
              frame #5 {
                n836 = Wait (ms)(milliseconds to wait=u32 50) -> ()  [unwired: 1 out]
              }
              frame #6 {
                w1942 = TRUE ("Value (Signaling)")
                n837 = Not(x=w1942) -> (.not. x?=w1941:bool)
                n838 = Not(x=w1942) -> (.not. x?=w1943:bool)
                n839 = property on="FirstScan" class="Bool (strict)"("Val(Sgnl)"=w1943) -> ()  [unwired: 2 in, 2 out]
                n840 = property on="Z Moved" class="Bool (strict)"("Val(Sgnl)"=w1942) -> ()  [unwired: 2 in, 2 out]
                n841 = property on="Scan Go" class="Bool (strict)"("Val(Sgnl)"=w1941) -> ()  [unwired: 2 in, 2 out]
              }
              frame #7 {
                n842 = Wait (ms)(milliseconds to wait=u32 75) -> ()  [unwired: 1 out]
              }
            }
          }
        }
        n843 = case shown="False" w1715 {
          tunnel: w1708 -> [w1718 w1724]
          tunnel: w1707 -> [w1719 w1723]
          tunnel: [w1719 w1722] -> w1700
          tunnel: [w1718 w1721] -> w1699
          frame #0 {
          }
          frame #1 {
            n844 = flat-sequence {
              tunnel: w1723 -> [w1751]
              tunnel: w1724 -> [w1752]
              tunnel: [w1752] -> w1738
              tunnel: [w1751] -> w1737
              tunnel: [w1739] -> w1736
              tunnel: [w1739] -> w1720
              tunnel: [w1758] -> w1735
              tunnel: [w1757] -> w1734
              tunnel: [w1756] -> w1733
              tunnel: w1736 -> [w1756]
              tunnel: w1737 -> [w1757]
              tunnel: w1738 -> [w1758]
              tunnel: w1720 -> [w1755]
              tunnel: [w1772] -> w1732
              tunnel: [w1771] -> w1731
              tunnel: w1735 -> [w1770]
              tunnel: w1734 -> [w1769]
              tunnel: [w1768] -> w1730
              tunnel: w1733 -> [w1768]
              tunnel: w1732 -> [w1778]
              tunnel: [w1778] -> w1729
              tunnel: w1731 -> [w1777]
              tunnel: [w1777] -> w1728
              tunnel: w1730 -> [w1776]
              tunnel: [w1776] -> w1727
              tunnel: [w1783] -> w1726
              tunnel: [w1782] -> w1725
              tunnel: w1729 -> [w1781]
              tunnel: w1728 -> [w1780]
              tunnel: w1727 -> [w1779]
              tunnel: [w1788] -> w1722
              tunnel: w1726 -> [w1788]
              tunnel: w1725 -> [w1787]
              tunnel: [w1787] -> w1721
              frame #0 {
                n845 = property on="R Position SP deg" class="DigNum (strict)"() -> ("Value"=w1745:dbl)  [unwired: 2 in, 2 out]
                n846 = property on="R offset deg" class="DigNum (strict)"() -> ("Value"=w1740:dbl)  [unwired: 2 in, 2 out]
                n847 = property on="R deg/rev" class="DigNum (strict)"() -> ("Value"=w1741:dbl)  [unwired: 2 in, 2 out]
                n848 = property on="R steps/rev" class="DigNum (strict)"() -> ("Value"=w1742:u32)  [unwired: 2 in, 2 out]
                n849 = To Double Precision Float(number=w1742) -> (double precision float=w1750:dbl)
                n850 = Subtract(x=w1745, y=w1740) -> (x-y=w1747:dbl)
                n851 = Divide(x=w1747, y=w1741) -> (x/y=w1746:dbl)
                n852 = Multiply(x=w1746, y=w1750) -> (x*y=w1748:dbl)
                n853 = property on="R Step SP" class="DigNum (strict)"() -> ("Maximum"=w1743:dbl)  [unwired: 2 in, 2 out]
                n854 = property on="R Step SP" class="DigNum (strict)"() -> ("Minimum"=w1744:dbl)  [unwired: 2 in, 2 out]
                n855 = In Range and Coerce(upper limit=w1743, x=w1748, lower limit=w1744) -> (coerced(x)=w1749:dbl)  [unwired: 1 out]
                n856 = To Long Integer(number=w1749) -> (32bit integer=w1739:i32)
              }
              frame #1 {
                n857 = property on="R Backlash" class="DigNum (strict)"() -> ("Value"=w1754:i32)  [unwired: 2 in, 2 out]
                n858 = property on="R Step PV" class="DigNum (strict)"() -> ("Value"=w1753:i32)  [unwired: 2 in, 2 out]
                n859 = Subtract(x=w1755, y=w1753) -> (x-y=w1764:i32)
                n860 = Sign(1:w1754) -> (0:w1762:i32)
                n861 = Sign(1:w1764) -> (0:w1763:i32)
                n862 = Multiply(x=w1763, y=w1762) -> (x*y=w1761:i32)
                n863 = Equal?(x=w1761, y=1) -> (x = y?=w1759:bool)
                n864 = case shown="True" w1759 {
                  frame #0 {
                    n865 = property on="R Backlash corr" class="Bool (strict)"("Val(Sgnl)"=FALSE ("Value (Signaling)")) -> ()  [unwired: 2 in, 2 out]
                  }
                  frame #1 {
                    n866 = property on="R Backlash corr" class="Bool (strict)"("Val(Sgnl)"=TRUE ("Value (Signaling)")) -> ()  [unwired: 2 in, 2 out]
                  }
                }
              }
              frame #2 {
                # "Velocity Setting"
                n867 = property on="R Velocity SP step/sec" class="DigNum (strict)"() -> ("Value"=w1767:i32)  [unwired: 2 in, 2 out]
                n868 = Number To Decimal String(number=w1767) -> (decimal integer string=w1773:string)  [unwired: 1 in]
                n869 = call "mDrive Send Command.vi"("error in (no error)"=w1770, "Extra"=w1773, "Command"=T10."Max Velocity", "VISA resource name"=w1769) -> ("error out"=w1771:errorcluster, "VISA resource name out"=w1772:refnum<visa-resource-name>)  [unwired: 3 in, 1 out]
              }
              frame #3 {
                n870 = Wait (ms)(milliseconds to wait=u32 50) -> ()  [unwired: 1 out]
              }
              frame #4 {
                # "Move to Abs Position"
                n871 = Number To Decimal String(number=w1779) -> (decimal integer string=w1785:string)  [unwired: 1 in]
                n872 = call "mDrive Send Command.vi"("error in (no error)"=w1780, "Extra"=w1785, "Command"=T10."Move to Absolute Position", "VISA resource name"=w1781) -> ("error out"=w1782:errorcluster, "VISA resource name out"=w1783:refnum<visa-resource-name>)  [unwired: 3 in, 1 out]
              }
              frame #5 {
                n873 = Wait (ms)(milliseconds to wait=u32 25) -> ()  [unwired: 1 out]
              }
            }
          }
        }
        n874 = case shown="True" w1688 {
          tunnel: w1710 -> [w1789 w1797]
          tunnel: w1709 -> [w1790 w1796]
          tunnel: [w1790 w1795] -> w1702
          tunnel: [w1789 w1794] -> w1701
          frame #0 {
          }
          frame #1 {
            n875 = flat-sequence {
              tunnel: [w1825] -> w1811
              tunnel: [w1824] -> w1810
              tunnel: [w1812] -> w1809
              tunnel: w1796 -> [w1824]
              tunnel: w1797 -> [w1825]
              tunnel: [w1812] -> w1793
              tunnel: [w1831] -> w1808
              tunnel: [w1830] -> w1807
              tunnel: [w1829] -> w1806
              tunnel: w1809 -> [w1829]
              tunnel: w1810 -> [w1830]
              tunnel: w1811 -> [w1831]
              tunnel: w1793 -> [w1828]
              tunnel: [w1845] -> w1805
              tunnel: [w1844] -> w1804
              tunnel: w1808 -> [w1843]
              tunnel: w1807 -> [w1842]
              tunnel: [w1841] -> w1803
              tunnel: w1806 -> [w1841]
              tunnel: w1805 -> [w1851]
              tunnel: [w1851] -> w1802
              tunnel: w1804 -> [w1850]
              tunnel: [w1850] -> w1801
              tunnel: [w1848] -> w1800
              tunnel: w1803 -> [w1848]
              tunnel: [w1856] -> w1799
              tunnel: [w1855] -> w1798
              tunnel: w1802 -> [w1854]
              tunnel: w1801 -> [w1853]
              tunnel: w1800 -> [w1852]
              tunnel: w1799 -> [w1861]
              tunnel: w1798 -> [w1859]
              tunnel: [w1861] -> w1792
              tunnel: [w1859] -> w1791
              tunnel: [w1864] -> w1794
              tunnel: [w1865] -> w1795
              tunnel: w1792 -> [w1865]
              tunnel: w1791 -> [w1864]
              frame #0 {
                n876 = property on="Y Position SP mm" class="DigNum (strict)"() -> ("Value"=w1818:dbl)  [unwired: 2 in, 2 out]
                n877 = property on="Y offset mm" class="DigNum (strict)"() -> ("Value"=w1813:dbl)  [unwired: 2 in, 2 out]
                n878 = property on="Y mm/rev" class="DigNum (strict)"() -> ("Value"=w1814:dbl)  [unwired: 2 in, 2 out]
                n879 = property on="Y steps/rev" class="DigNum (strict)"() -> ("Value"=w1815:u32)  [unwired: 2 in, 2 out]
                n880 = To Double Precision Float(number=w1815) -> (double precision float=w1823:dbl)
                n881 = Subtract(x=w1818, y=w1813) -> (x-y=w1820:dbl)
                n882 = Divide(x=w1820, y=w1814) -> (x/y=w1819:dbl)
                n883 = Multiply(x=w1819, y=w1823) -> (x*y=w1821:dbl)
                n884 = property on="Y Step SP" class="DigNum (strict)"() -> ("Maximum"=w1817:dbl)  [unwired: 2 in, 2 out]
                n885 = property on="Y Step SP" class="DigNum (strict)"() -> ("Minimum"=w1816:dbl)  [unwired: 2 in, 2 out]
                n886 = In Range and Coerce(upper limit=w1817, x=w1821, lower limit=w1816) -> (coerced(x)=w1822:dbl)  [unwired: 1 out]
                n887 = To Long Integer(number=w1822) -> (32bit integer=w1812:i32)
              }
              frame #1 {
                n888 = property on="Y Step PV" class="DigNum (strict)"() -> ("Value"=w1826:i32)  [unwired: 2 in, 2 out]
                n889 = property on="Y Backlash" class="DigNum (strict)"() -> ("Value"=w1827:i32)  [unwired: 2 in, 2 out]
                n890 = Subtract(x=w1828, y=w1826) -> (x-y=w1837:i32)
                n891 = Sign(1:w1827) -> (0:w1835:i32)
                n892 = Sign(1:w1837) -> (0:w1836:i32)
                n893 = Multiply(x=w1836, y=w1835) -> (x*y=w1834:i32)
                n894 = Equal?(x=w1834, y=1) -> (x = y?=w1832:bool)
                n895 = case shown="False" w1832 {
                  frame #0 {
                    n896 = property on="Y Backlash corr" class="Bool (strict)"("Val(Sgnl)"=FALSE ("Value (Signaling)")) -> ()  [unwired: 2 in, 2 out]
                  }
                  frame #1 {
                    n897 = property on="Y Backlash corr" class="Bool (strict)"("Val(Sgnl)"=TRUE ("Value (Signaling)")) -> ()  [unwired: 2 in, 2 out]
                  }
                }
              }
              frame #2 {
                # "Velocity Setting"
                n898 = property on="Y Velocity SP step/sec" class="DigNum (strict)"() -> ("Value"=w1840:i32)  [unwired: 2 in, 2 out]
                n899 = Number To Decimal String(number=w1840) -> (decimal integer string=w1846:string)  [unwired: 1 in]
                n900 = call "mDrive Send Command.vi"("error in (no error)"=w1843, "Extra"=w1846, "Command"=T10."Max Velocity", "VISA resource name"=w1842) -> ("error out"=w1844:errorcluster, "VISA resource name out"=w1845:refnum<visa-resource-name>)  [unwired: 3 in, 1 out]
              }
              frame #3 {
                n901 = Wait (ms)(milliseconds to wait=u32 50) -> ()  [unwired: 1 out]
              }
              frame #4 {
                # "Move to Abs Position"
                n902 = Number To Decimal String(number=w1852) -> (decimal integer string=w1858:string)  [unwired: 1 in]
                n903 = call "mDrive Send Command.vi"("error in (no error)"=w1853, "Extra"=w1858, "Command"=T10."Move to Absolute Position", "VISA resource name"=w1854) -> ("error out"=w1855:errorcluster, "VISA resource name out"=w1856:refnum<visa-resource-name>)  [unwired: 3 in, 1 out]
              }
              frame #5 {
                n904 = Wait (ms)(milliseconds to wait=u32 25) -> ()  [unwired: 1 out]
              }
              frame #6 {
                n905 = property on="Z Moved" class="Bool (strict)"("Val(Sgnl)"=FALSE ("Value (Signaling)")) -> ()  [unwired: 2 in, 2 out]
                n906 = property on="NewLoop" class="Bool (strict)"("Val(Sgnl)"=TRUE ("Value (Signaling)")) -> ()  [unwired: 2 in, 2 out]
              }
            }
          }
        }
        n907 = case shown="False" w1717 {
          tunnel: w1713 -> [w1950 w1955]
          tunnel: w1714 -> [w1949 w1954]
          tunnel: [w1950 w1953] -> w1706
          tunnel: [w1949 w1952] -> w1705
          frame #0 {
          }
          frame #1 {
            n908 = flat-sequence {
              tunnel: w1954 -> [w1982]
              tunnel: w1955 -> [w1983]
              tunnel: [w1983] -> w1969
              tunnel: [w1982] -> w1968
              tunnel: [w1970] -> w1967
              tunnel: [w1970] -> w1951
              tunnel: [w1989] -> w1966
              tunnel: [w1988] -> w1965
              tunnel: [w1987] -> w1964
              tunnel: w1967 -> [w1987]
              tunnel: w1968 -> [w1988]
              tunnel: w1969 -> [w1989]
              tunnel: w1951 -> [w1986]
              tunnel: [w2003] -> w1963
              tunnel: [w2002] -> w1962
              tunnel: w1966 -> [w2001]
              tunnel: w1965 -> [w2000]
              tunnel: w1964 -> [w1999]
              tunnel: [w1999] -> w1961
              tunnel: w1963 -> [w2009]
              tunnel: [w2009] -> w1960
              tunnel: w1962 -> [w2008]
              tunnel: [w2008] -> w1959
              tunnel: [w2006] -> w1958
              tunnel: w1961 -> [w2006]
              tunnel: [w2014] -> w1957
              tunnel: [w2013] -> w1956
              tunnel: w1960 -> [w2012]
              tunnel: w1959 -> [w2011]
              tunnel: w1958 -> [w2010]
              tunnel: [w2018] -> w1952
              tunnel: [w2019] -> w1953
              tunnel: w1957 -> [w2019]
              tunnel: w1956 -> [w2018]
              frame #0 {
                n909 = property on="X Position SP mm" class="DigNum (strict)"() -> ("Value"=w1976:dbl)  [unwired: 2 in, 2 out]
                n910 = property on="X offset mm" class="DigNum (strict)"() -> ("Value"=w1975:dbl)  [unwired: 2 in, 2 out]
                n911 = property on="X mm/rev" class="DigNum (strict)"() -> ("Value"=w1974:dbl)  [unwired: 2 in, 2 out]
                n912 = property on="X steps/rev" class="DigNum (strict)"() -> ("Value"=w1973:u32)  [unwired: 2 in, 2 out]
                n913 = To Double Precision Float(number=w1973) -> (double precision float=w1981:dbl)
                n914 = Subtract(x=w1976, y=w1975) -> (x-y=w1978:dbl)
                n915 = Divide(x=w1978, y=w1974) -> (x/y=w1977:dbl)
                n916 = property on="X Step SP" class="DigNum (strict)"() -> ("Maximum"=w1971:dbl)  [unwired: 2 in, 2 out]
                n917 = Multiply(x=w1977, y=w1981) -> (x*y=w1979:dbl)
                n918 = property on="X Step SP" class="DigNum (strict)"() -> ("Minimum"=w1972:dbl)  [unwired: 2 in, 2 out]
                n919 = In Range and Coerce(upper limit=w1971, x=w1979, lower limit=w1972) -> (coerced(x)=w1980:dbl)  [unwired: 1 out]
                n920 = To Long Integer(number=w1980) -> (32bit integer=w1970:i32)
              }
              frame #1 {
                n921 = property on="X Step PV" class="DigNum (strict)"() -> ("Value"=w1984:i32)  [unwired: 2 in, 2 out]
                n922 = property on="X Backlash" class="DigNum (strict)"() -> ("Value"=w1985:i32)  [unwired: 2 in, 2 out]
                n923 = Sign(1:w1985) -> (0:w1993:i32)
                n924 = Subtract(x=w1986, y=w1984) -> (x-y=w1995:i32)
                n925 = Sign(1:w1995) -> (0:w1994:i32)
                n926 = Multiply(x=w1994, y=w1993) -> (x*y=w1992:i32)
                n927 = Equal?(x=w1992, y=1) -> (x = y?=w1990:bool)
                n928 = case shown="False" w1990 {
                  frame #0 {
                    n929 = property on="X Backlash corr" class="Bool (strict)"("Val(Sgnl)"=FALSE ("Value (Signaling)")) -> ()  [unwired: 2 in, 2 out]
                  }
                  frame #1 {
                    n930 = property on="X Backlash corr" class="Bool (strict)"("Val(Sgnl)"=TRUE ("Value (Signaling)")) -> ()  [unwired: 2 in, 2 out]
                  }
                }
              }
              frame #2 {
                # "Velocity Setting"
                n931 = property on="X Velocity SP step/sec" class="DigNum (strict)"() -> ("Value"=w1998:i32)  [unwired: 2 in, 2 out]
                n932 = Number To Decimal String(number=w1998) -> (decimal integer string=w2004:string)  [unwired: 1 in]
                n933 = call "mDrive Send Command.vi"("error in (no error)"=w2000, "Extra"=w2004, "Command"=T10."Max Velocity", "VISA resource name"=w2001) -> ("error out"=w2002:errorcluster, "VISA resource name out"=w2003:refnum<visa-resource-name>)  [unwired: 3 in, 1 out]
              }
              frame #3 {
                n934 = Wait (ms)(milliseconds to wait=u32 50) -> ()  [unwired: 1 out]
              }
              frame #4 {
                # "Move to Abs Position"
                n935 = Number To Decimal String(number=w2010) -> (decimal integer string=w2016:string)  [unwired: 1 in]
                n936 = call "mDrive Send Command.vi"("error in (no error)"=w2011, "Extra"=w2016, "Command"=T10."Move to Absolute Position", "VISA resource name"=w2012) -> ("error out"=w2013:errorcluster, "VISA resource name out"=w2014:refnum<visa-resource-name>)  [unwired: 3 in, 1 out]
              }
              frame #5 {
                n937 = Wait (ms)(milliseconds to wait=u32 50) -> ()  [unwired: 1 out]
              }
            }
          }
        }
      }
      event #4 {
        n938 = event-data() -> ()  [unwired: 1 in, 7 out]
        n939 = flat-sequence {
          tunnel: w2053 -> [w2108]
          tunnel: [w2107] -> w2047
          tunnel: w2032 -> [w2106]
          tunnel: [w2105] -> w2030
          tunnel: [w2112] -> w2048
          tunnel: w2047 -> [w2112]
          tunnel: [w2111] -> w2031
          tunnel: w2030 -> [w2111]
          tunnel: w2048 -> [w2129]
          tunnel: w2031 -> [w2126]
          tunnel: [w2125] -> w2024
          tunnel: [w2124] -> w2023
          frame #0 {
            n940 = call "mDrive Send Command.vi"("error in (no error)"=w2108, "Command"=T10."Stop", "VISA resource name"=w2106) -> ("error out"=w2107:errorcluster, "VISA resource name out"=w2105:refnum<visa-resource-name>)  [unwired: 4 in, 1 out]
          }
          frame #1 {
            n941 = Wait (ms)(milliseconds to wait=u32 50) -> ()  [unwired: 1 out]
          }
          frame #2 {
            n942 = call "mDrive Send Command.vi"("error in (no error)"=w2129, "Extra"="P", "Command"=T10."Print Parameter", "VISA resource name"=w2126) -> ("error out"=w2124:errorcluster, "read buffer"=w2119:string, "VISA resource name out"=w2125:refnum<visa-resource-name>)  [unwired: 3 in]
            n943 = property on="Z steps/rev" class="DigNum (strict)"() -> ("Value"=w2115:u32)  [unwired: 2 in, 2 out]
            n944 = Decimal String To Number(string=w2119, offset=0) -> (number=w2117:i32)  [unwired: 1 in, 1 out]
            n945 = property on="Z mm/rev" class="DigNum (strict)"() -> ("Value"=w2114:dbl)  [unwired: 2 in, 2 out]
            n946 = property on="Z Step PV" class="DigNum (strict)"("Val(Sgnl)"=w2117) -> ()  [unwired: 2 in, 2 out]
            n947 = To Double Precision Float(number=w2117) -> (double precision float=w2121:dbl)
            n948 = To Double Precision Float(number=w2115) -> (double precision float=w2120:dbl)
            n949 = property on="Z offset mm" class="DigNum (strict)"() -> ("Value"=w2113:dbl)  [unwired: 2 in, 2 out]
            n950 = Divide(x=w2121, y=w2120) -> (x/y=w2123:dbl)
            n951 = Multiply(x=w2123, y=w2114) -> (x*y=w2122:dbl)
            n952 = Add(x=w2122, y=w2113) -> (x+y=w2116:dbl)
            n953 = property on="Z Position mm PV" class="DigNum (strict)"("Val(Sgnl)"=w2116) -> ()  [unwired: 2 in, 2 out]
          }
        }
        n954 = flat-sequence {
          tunnel: w2054 -> [w2083]
          tunnel: [w2082] -> w2049
          tunnel: w2029 -> [w2081]
          tunnel: [w2080] -> w2027
          tunnel: [w2087] -> w2050
          tunnel: w2049 -> [w2087]
          tunnel: [w2086] -> w2028
          tunnel: w2027 -> [w2086]
          tunnel: w2050 -> [w2104]
          tunnel: w2028 -> [w2101]
          tunnel: [w2100] -> w2026
          tunnel: [w2099] -> w2025
          frame #0 {
            n955 = call "mDrive Send Command.vi"("error in (no error)"=w2083, "Command"=T10."Stop", "VISA resource name"=w2081) -> ("error out"=w2082:errorcluster, "VISA resource name out"=w2080:refnum<visa-resource-name>)  [unwired: 4 in, 1 out]
          }
          frame #1 {
            n956 = Wait (ms)(milliseconds to wait=u32 50) -> ()  [unwired: 1 out]
          }
          frame #2 {
            n957 = call "mDrive Send Command.vi"("error in (no error)"=w2104, "Extra"="P", "Command"=T10."Print Parameter", "VISA resource name"=w2101) -> ("error out"=w2099:errorcluster, "read buffer"=w2094:string, "VISA resource name out"=w2100:refnum<visa-resource-name>)  [unwired: 3 in]
            n958 = property on="X steps/rev" class="DigNum (strict)"() -> ("Value"=w2090:u32)  [unwired: 2 in, 2 out]
            n959 = Decimal String To Number(string=w2094, offset=0) -> (number=w2092:i32)  [unwired: 1 in, 1 out]
            n960 = property on="X mm/rev" class="DigNum (strict)"() -> ("Value"=w2089:dbl)  [unwired: 2 in, 2 out]
            n961 = property on="X Step PV" class="DigNum (strict)"("Val(Sgnl)"=w2092) -> ()  [unwired: 2 in, 2 out]
            n962 = To Double Precision Float(number=w2092) -> (double precision float=w2096:dbl)
            n963 = To Double Precision Float(number=w2090) -> (double precision float=w2095:dbl)
            n964 = property on="X offset mm" class="DigNum (strict)"() -> ("Value"=w2088:dbl)  [unwired: 2 in, 2 out]
            n965 = Divide(x=w2096, y=w2095) -> (x/y=w2098:dbl)
            n966 = Multiply(x=w2098, y=w2089) -> (x*y=w2097:dbl)
            n967 = Add(x=w2097, y=w2088) -> (x+y=w2091:dbl)
            n968 = property on="X Position mm PV" class="DigNum (strict)"("Val(Sgnl)"=w2091) -> ()  [unwired: 2 in, 2 out]
          }
        }
        n969 = flat-sequence {
          tunnel: w2052 -> [w2133]
          tunnel: [w2132] -> w2045
          tunnel: w2039 -> [w2131]
          tunnel: [w2130] -> w2037
          tunnel: [w2137] -> w2046
          tunnel: w2045 -> [w2137]
          tunnel: [w2136] -> w2038
          tunnel: w2037 -> [w2136]
          tunnel: w2046 -> [w2154]
          tunnel: w2038 -> [w2151]
          tunnel: [w2150] -> w2036
          tunnel: [w2149] -> w2035
          frame #0 {
            n970 = call "mDrive Send Command.vi"("error in (no error)"=w2133, "Command"=T10."Stop", "VISA resource name"=w2131) -> ("error out"=w2132:errorcluster, "VISA resource name out"=w2130:refnum<visa-resource-name>)  [unwired: 4 in, 1 out]
          }
          frame #1 {
            n971 = Wait (ms)(milliseconds to wait=u32 50) -> ()  [unwired: 1 out]
          }
          frame #2 {
            n972 = call "mDrive Send Command.vi"("error in (no error)"=w2154, "Extra"="P", "Command"=T10."Print Parameter", "VISA resource name"=w2151) -> ("error out"=w2149:errorcluster, "read buffer"=w2144:string, "VISA resource name out"=w2150:refnum<visa-resource-name>)  [unwired: 3 in]
            n973 = property on="Y steps/rev" class="DigNum (strict)"() -> ("Value"=w2140:u32)  [unwired: 2 in, 2 out]
            n974 = Decimal String To Number(string=w2144, offset=0) -> (number=w2141:i32)  [unwired: 1 in, 1 out]
            n975 = property on="Y mm/rev" class="DigNum (strict)"() -> ("Value"=w2139:dbl)  [unwired: 2 in, 2 out]
            n976 = To Double Precision Float(number=w2141) -> (double precision float=w2146:dbl)
            n977 = To Double Precision Float(number=w2140) -> (double precision float=w2145:dbl)
            n978 = property on="Y offset mm" class="DigNum (strict)"() -> ("Value"=w2138:dbl)  [unwired: 2 in, 2 out]
            n979 = Divide(x=w2146, y=w2145) -> (x/y=w2148:dbl)
            n980 = property on="Y Step PV" class="DigNum (strict)"("Val(Sgnl)"=w2141) -> ()  [unwired: 2 in, 2 out]
            n981 = Multiply(x=w2148, y=w2139) -> (x*y=w2147:dbl)
            n982 = Add(x=w2147, y=w2138) -> (x+y=w2142:dbl)
            n983 = property on="Y Position mm PV" class="DigNum (strict)"("Val(Sgnl)"=w2142) -> ()  [unwired: 2 in, 2 out]
          }
        }
        n984 = flat-sequence {
          tunnel: w2051 -> [w2058]
          tunnel: [w2057] -> w2043
          tunnel: w2042 -> [w2056]
          tunnel: [w2055] -> w2040
          tunnel: [w2062] -> w2044
          tunnel: w2043 -> [w2062]
          tunnel: [w2061] -> w2041
          tunnel: w2040 -> [w2061]
          tunnel: w2044 -> [w2079]
          tunnel: w2041 -> [w2076]
          tunnel: [w2075] -> w2034
          tunnel: [w2074] -> w2033
          frame #0 {
            n985 = call "mDrive Send Command.vi"("error in (no error)"=w2058, "Command"=T10."Stop", "VISA resource name"=w2056) -> ("error out"=w2057:errorcluster, "VISA resource name out"=w2055:refnum<visa-resource-name>)  [unwired: 4 in, 1 out]
          }
          frame #1 {
            n986 = Wait (ms)(milliseconds to wait=u32 50) -> ()  [unwired: 1 out]
          }
          frame #2 {
            n987 = call "mDrive Send Command.vi"("error in (no error)"=w2079, "Extra"="P", "Command"=T10."Print Parameter", "VISA resource name"=w2076) -> ("error out"=w2074:errorcluster, "read buffer"=w2069:string, "VISA resource name out"=w2075:refnum<visa-resource-name>)  [unwired: 3 in]
            n988 = property on="R steps/rev" class="DigNum (strict)"() -> ("Value"=w2067:u32)  [unwired: 2 in, 2 out]
            n989 = Decimal String To Number(string=w2069, offset=0) -> (number=w2066:i32)  [unwired: 1 in, 1 out]
            n990 = property on="R deg/rev" class="DigNum (strict)"() -> ("Value"=w2065:dbl)  [unwired: 2 in, 2 out]
            n991 = property on="R Step PV" class="DigNum (strict)"("Val(Sgnl)"=w2066) -> ()  [unwired: 2 in, 2 out]
            n992 = To Double Precision Float(number=w2066) -> (double precision float=w2071:dbl)
            n993 = To Double Precision Float(number=w2067) -> (double precision float=w2070:dbl)
            n994 = property on="R offset deg" class="DigNum (strict)"() -> ("Value"=w2064:dbl)  [unwired: 2 in, 2 out]
            n995 = Divide(x=w2071, y=w2070) -> (x/y=w2073:dbl)
            n996 = Multiply(x=w2073, y=w2065) -> (x*y=w2072:dbl)
            n997 = Add(x=w2072, y=w2064) -> (x+y=w2063:dbl)
            n998 = property on="R Position deg PV" class="DigNum (strict)"("Val(Sgnl)"=w2063) -> ()  [unwired: 2 in, 2 out]
          }
        }
        n999 = property on="GO" class="Bool"("DisabledEnum"=T1."Enabled" ("Disabled")) -> ()  [unwired: 2 in, 2 out]
      }
      event #5 {
        n1000 = event-data() -> ()  [unwired: 1 in, 5 out]
        n1001 = local write "STATUS"("RESSETTING" ("STATUS")) -> ()
        n1002 = property on="R offset deg" class="DigNum (strict)"() -> ("Value"=w2166:dbl)  [unwired: 2 in, 2 out]
        n1003 = property on="Reset Z Position mm" class="DigNum (strict)"() -> ("Value"=w2183:dbl)  [unwired: 2 in, 2 out]
        n1004 = property on="Z offset mm" class="DigNum (strict)"() -> ("Value"=w2175:dbl)  [unwired: 2 in, 2 out]
        n1005 = property on="Reset R Position deg" class="DigNum (strict)"() -> ("Value"=w2174:dbl)  [unwired: 2 in, 2 out]
        n1006 = property on="Reset X Position mm" class="DigNum (strict)"() -> ("Value"=w2192:dbl)  [unwired: 2 in, 2 out]
        n1007 = property on="X offset mm" class="DigNum (strict)"() -> ("Value"=w2184:dbl)  [unwired: 2 in, 2 out]
        n1008 = property on="Reset Y Position mm" class="DigNum (strict)"() -> ("Value"=w2201:dbl)  [unwired: 2 in, 2 out]
        n1009 = property on="Y offset mm" class="DigNum (strict)"() -> ("Value"=w2193:dbl)  [unwired: 2 in, 2 out]
        n1010 = Subtract(x=w2183, y=w2175) -> (x-y=w2182:dbl)
        n1011 = Subtract(x=w2174, y=w2166) -> (x-y=w2173:dbl)
        n1012 = Subtract(x=w2192, y=w2184) -> (x-y=w2191:dbl)
        n1013 = Subtract(x=w2201, y=w2193) -> (x-y=w2200:dbl)
        n1014 = property on="X mm/rev" class="DigNum (strict)"() -> ("Value"=w2185:dbl)  [unwired: 2 in, 2 out]
        n1015 = property on="R deg/rev" class="DigNum (strict)"() -> ("Value"=w2167:dbl)  [unwired: 2 in, 2 out]
        n1016 = property on="Y mm/rev" class="DigNum (strict)"() -> ("Value"=w2194:dbl)  [unwired: 2 in, 2 out]
        n1017 = property on="Z mm/rev" class="DigNum (strict)"() -> ("Value"=w2176:dbl)  [unwired: 2 in, 2 out]
        n1018 = Divide(x=w2173, y=w2167) -> (x/y=w2172:dbl)
        n1019 = Divide(x=w2191, y=w2185) -> (x/y=w2190:dbl)
        n1020 = Divide(x=w2200, y=w2194) -> (x/y=w2199:dbl)
        n1021 = Divide(x=w2182, y=w2176) -> (x/y=w2181:dbl)
        n1022 = property on="R steps/rev" class="DigNum (strict)"() -> ("Value"=w2168:u32)  [unwired: 2 in, 2 out]
        n1023 = property on="Z steps/rev" class="DigNum (strict)"() -> ("Value"=w2177:u32)  [unwired: 2 in, 2 out]
        n1024 = property on="X steps/rev" class="DigNum (strict)"() -> ("Value"=w2186:u32)  [unwired: 2 in, 2 out]
        n1025 = property on="Y steps/rev" class="DigNum (strict)"() -> ("Value"=w2195:u32)  [unwired: 2 in, 2 out]
        n1026 = To Double Precision Float(number=w2177) -> (double precision float=w2180:dbl)
        n1027 = To Double Precision Float(number=w2168) -> (double precision float=w2171:dbl)
        n1028 = To Double Precision Float(number=w2186) -> (double precision float=w2189:dbl)
        n1029 = To Double Precision Float(number=w2195) -> (double precision float=w2198:dbl)
        n1030 = Multiply(x=w2181, y=w2180) -> (x*y=w2179:dbl)
        n1031 = Multiply(x=w2172, y=w2171) -> (x*y=w2170:dbl)
        n1032 = Multiply(x=w2190, y=w2189) -> (x*y=w2188:dbl)
        n1033 = Multiply(x=w2199, y=w2198) -> (x*y=w2197:dbl)
        n1034 = To Long Integer(number=w2179) -> (32bit integer=w2178:i32)
        n1035 = To Long Integer(number=w2170) -> (32bit integer=w2169:i32)
        n1036 = To Long Integer(number=w2188) -> (32bit integer=w2187:i32)
        n1037 = To Long Integer(number=w2197) -> (32bit integer=w2196:i32)
        n1038 = property on="Reset Z Motor Steps" class="DigNum (strict)"("Val(Sgnl)"=w2178) -> ()  [unwired: 2 in, 2 out]
        n1039 = property on="Reset R Motor Steps" class="DigNum (strict)"("Val(Sgnl)"=w2169) -> ()  [unwired: 2 in, 2 out]
        n1040 = property on="Reset X Motor Steps" class="DigNum (strict)"("Val(Sgnl)"=w2187) -> ()  [unwired: 2 in, 2 out]
        n1041 = property on="Reset Y Motor Steps" class="DigNum (strict)"("Val(Sgnl)"=w2196) -> ()  [unwired: 2 in, 2 out]
      }
      event #6 {
        n1042 = event-data() -> ()  [unwired: 1 in, 5 out]
        n1043 = property on="Y steps/rev" class="DigNum (strict)"() -> ("Value"=w2265:u32)  [unwired: 2 in, 2 out]
        n1044 = property on="Y Step SP" class="DigNum (strict)"() -> ("Value"=w2242:i32)  [unwired: 2 in, 2 out]
        n1045 = property on="Y steps/rev" class="DigNum (strict)"() -> ("Value"=w2240:u32)  [unwired: 2 in, 2 out]
        n1046 = property on="Y Velocity SP step/sec" class="DigNum (strict)"() -> ("Value"=w2267:i32)  [unwired: 2 in, 2 out]
        n1047 = property on="Y mm/rev" class="DigNum (strict)"() -> ("Value"=w2211:dbl)  [unwired: 2 in, 2 out]
        n1048 = property on="Y offset mm" class="DigNum (strict)"() -> ("Value"=w2239:dbl)  [unwired: 2 in, 2 out]
        n1049 = To Double Precision Float(number=w2242) -> (double precision float=w2243:dbl)
        n1050 = To Double Precision Float(number=w2240) -> (double precision float=w2246:dbl)
        n1051 = To Double Precision Float(number=w2267) -> (double precision float=w2268:dbl)
        n1052 = To Double Precision Float(number=w2265) -> (double precision float=w2270:dbl)
        n1053 = Divide(x=w2243, y=w2246) -> (x/y=w2245:dbl)
        n1054 = Divide(x=w2268, y=w2270) -> (x/y=w2269:dbl)
        n1055 = Multiply(x=w2245, y=w2211) -> (x*y=w2244:dbl)
        n1056 = Multiply(x=w2269, y=w2211) -> (x*y=w2266:dbl)
        n1057 = Add(x=w2244, y=w2239) -> (x+y=w2241:dbl)
        n1058 = property on="Y Velocity MV mm/sec" class="DigNum (strict)"("Val(Sgnl)"=w2266) -> ()  [unwired: 2 in, 2 out]
        n1059 = property on="Y Position MV mm" class="DigNum (strict)"("Val(Sgnl)"=w2241) -> ()  [unwired: 2 in, 2 out]
        n1060 = property on="Z steps/rev" class="DigNum (strict)"() -> ("Value"=w2253:u32)  [unwired: 2 in, 2 out]
        n1061 = property on="Z Step SP" class="DigNum (strict)"() -> ("Value"=w2226:i32)  [unwired: 2 in, 2 out]
        n1062 = property on="Z steps/rev" class="DigNum (strict)"() -> ("Value"=w2224:u32)  [unwired: 2 in, 2 out]
        n1063 = property on="Z Velocity SP step/sec" class="DigNum (strict)"() -> ("Value"=w2255:i32)  [unwired: 2 in, 2 out]
        n1064 = property on="Z mm/rev" class="DigNum (strict)"() -> ("Value"=w2213:dbl)  [unwired: 2 in, 2 out]
        n1065 = property on="Z offset mm" class="DigNum (strict)"() -> ("Value"=w2223:dbl)  [unwired: 2 in, 2 out]
        n1066 = To Double Precision Float(number=w2255) -> (double precision float=w2256:dbl)
        n1067 = To Double Precision Float(number=w2253) -> (double precision float=w2258:dbl)
        n1068 = To Double Precision Float(number=w2226) -> (double precision float=w2227:dbl)
        n1069 = To Double Precision Float(number=w2224) -> (double precision float=w2230:dbl)
        n1070 = Divide(x=w2227, y=w2230) -> (x/y=w2229:dbl)
        n1071 = Divide(x=w2256, y=w2258) -> (x/y=w2257:dbl)
        n1072 = Multiply(x=w2229, y=w2213) -> (x*y=w2228:dbl)
        n1073 = Multiply(x=w2257, y=w2213) -> (x*y=w2254:dbl)
        n1074 = Add(x=w2228, y=w2223) -> (x+y=w2225:dbl)
        n1075 = property on="Z Velocity MV mm/sec" class="DigNum (strict)"("Val(Sgnl)"=w2254) -> ()  [unwired: 2 in, 2 out]
        n1076 = property on="Z Position MV mm" class="DigNum (strict)"("Val(Sgnl)"=w2225) -> ()  [unwired: 2 in, 2 out]
        n1077 = property on="X Velocity SP step/sec" class="DigNum (strict)"() -> ("Value"=w2261:i32)  [unwired: 2 in, 2 out]
        n1078 = property on="X steps/rev" class="DigNum (strict)"() -> ("Value"=w2259:u32)  [unwired: 2 in, 2 out]
        n1079 = property on="X Step SP" class="DigNum (strict)"() -> ("Value"=w2234:i32)  [unwired: 2 in, 2 out]
        n1080 = property on="X steps/rev" class="DigNum (strict)"() -> ("Value"=w2232:u32)  [unwired: 2 in, 2 out]
        n1081 = property on="X offset mm" class="DigNum (strict)"() -> ("Value"=w2231:dbl)  [unwired: 2 in, 2 out]
        n1082 = property on="X mm/rev" class="DigNum (strict)"() -> ("Value"=w2212:dbl)  [unwired: 2 in, 2 out]
        n1083 = To Double Precision Float(number=w2234) -> (double precision float=w2235:dbl)
        n1084 = To Double Precision Float(number=w2232) -> (double precision float=w2238:dbl)
        n1085 = To Double Precision Float(number=w2261) -> (double precision float=w2262:dbl)
        n1086 = To Double Precision Float(number=w2259) -> (double precision float=w2264:dbl)
        n1087 = Divide(x=w2235, y=w2238) -> (x/y=w2237:dbl)
        n1088 = Divide(x=w2262, y=w2264) -> (x/y=w2263:dbl)
        n1089 = Multiply(x=w2237, y=w2212) -> (x*y=w2236:dbl)
        n1090 = Add(x=w2236, y=w2231) -> (x+y=w2233:dbl)
        n1091 = Multiply(x=w2263, y=w2212) -> (x*y=w2260:dbl)
        n1092 = property on="X Velocity MV mm/sec" class="DigNum (strict)"("Val(Sgnl)"=w2260) -> ()  [unwired: 2 in, 2 out]
        n1093 = property on="X Position MV mm" class="DigNum (strict)"("Val(Sgnl)"=w2233) -> ()  [unwired: 2 in, 2 out]
        n1094 = property on="R steps/rev" class="DigNum (strict)"() -> ("Value"=w2247:u32)  [unwired: 2 in, 2 out]
        n1095 = property on="R Step SP" class="DigNum (strict)"() -> ("Value"=w2218:i32)  [unwired: 2 in, 2 out]
        n1096 = property on="R steps/rev" class="DigNum (strict)"() -> ("Value"=w2216:u32)  [unwired: 2 in, 2 out]
        n1097 = property on="R deg/rev" class="DigNum (strict)"() -> ("Value"=w2214:dbl)  [unwired: 2 in, 2 out]
        n1098 = property on="R offset deg" class="DigNum (strict)"() -> ("Value"=w2215:dbl)  [unwired: 2 in, 2 out]
        n1099 = property on="R Velocity SP step/sec" class="DigNum (strict)"() -> ("Value"=w2249:i32)  [unwired: 2 in, 2 out]
        n1100 = To Double Precision Float(number=w2218) -> (double precision float=w2219:dbl)
        n1101 = To Double Precision Float(number=w2216) -> (double precision float=w2222:dbl)
        n1102 = To Double Precision Float(number=w2247) -> (double precision float=w2252:dbl)
        n1103 = To Double Precision Float(number=w2249) -> (double precision float=w2250:dbl)
        n1104 = Divide(x=w2219, y=w2222) -> (x/y=w2221:dbl)
        n1105 = Divide(x=w2250, y=w2252) -> (x/y=w2251:dbl)
        n1106 = Multiply(x=w2221, y=w2214) -> (x*y=w2220:dbl)
        n1107 = Multiply(x=w2251, y=w2214) -> (x*y=w2248:dbl)
        n1108 = Add(x=w2220, y=w2215) -> (x+y=w2217:dbl)
        n1109 = Absolute Value(x=w2248) -> (abs(x)=w2210:dbl)
        n1110 = property on="R Position MV deg" class="DigNum (strict)"("Val(Sgnl)"=w2217) -> ()  [unwired: 2 in, 2 out]
        n1111 = property on="R Velocity MVdeg/sec" class="DigNum (strict)"("Val(Sgnl)"=w2210) -> ()  [unwired: 2 in, 2 out]
      }
      event #7 {
        n1112 = event-data() -> ()  [unwired: 1 in, 5 out]
        n1113 = property on="R Step PV" class="DigNum (strict)"() -> ("Value"=w2311:i32)  [unwired: 2 in, 2 out]
        n1114 = property on="R Step SP" class="DigNum (strict)"() -> ("Maximum"=w2319:dbl)  [unwired: 2 in, 2 out]
        n1115 = property on="R Step SP" class="DigNum (strict)"() -> ("Minimum"=w2316:dbl)  [unwired: 2 in, 2 out]
        n1116 = property on="X Step PV" class="DigNum (strict)"() -> ("Value"=w2351:i32)  [unwired: 2 in, 2 out]
        n1117 = property on="Z Step PV" class="DigNum (strict)"() -> ("Value"=w2325:i32)  [unwired: 2 in, 2 out]
        n1118 = property on="Z Step SP" class="DigNum (strict)"() -> ("Minimum"=w2332:dbl)  [unwired: 2 in, 2 out]
        n1119 = property on="Z Step SP" class="DigNum (strict)"() -> ("Maximum"=w2331:dbl)  [unwired: 2 in, 2 out]
        n1120 = property on="X Step SP" class="DigNum (strict)"() -> ("Maximum"=w2355:dbl)  [unwired: 2 in, 2 out]
        n1121 = property on="Y Step SP" class="DigNum (strict)"() -> ("Minimum"=w2345:dbl)  [unwired: 2 in, 2 out]
        n1122 = property on="Y Step SP" class="DigNum (strict)"() -> ("Maximum"=w2344:dbl)  [unwired: 2 in, 2 out]
        n1123 = property on="X Step SP" class="DigNum (strict)"() -> ("Minimum"=w2356:dbl)  [unwired: 2 in, 2 out]
        n1124 = property on="Y Step PV" class="DigNum (strict)"() -> ("Value"=w2338:i32)  [unwired: 2 in, 2 out]
        n1125 = To Double Precision Float(number=w2311) -> (double precision float=w2302:dbl)
        n1126 = To Double Precision Float(number=w2351) -> (double precision float=w2305:dbl)
        n1127 = To Double Precision Float(number=w2325) -> (double precision float=w2303:dbl)
        n1128 = To Double Precision Float(number=w2338) -> (double precision float=w2304:dbl)
        n1129 = Subtract(x=w2316, y=w2302) -> (x-y=w2317:dbl)
        n1130 = Subtract(x=w2319, y=w2302) -> (x-y=w2318:dbl)
        n1131 = Subtract(x=w2345, y=w2304) -> (x-y=w2346:dbl)
        n1132 = Subtract(x=w2344, y=w2304) -> (x-y=w2343:dbl)
        n1133 = Subtract(x=w2356, y=w2305) -> (x-y=w2357:dbl)
        n1134 = Subtract(x=w2355, y=w2305) -> (x-y=w2354:dbl)
        n1135 = Subtract(x=w2332, y=w2303) -> (x-y=w2333:dbl)
        n1136 = Subtract(x=w2331, y=w2303) -> (x-y=w2330:dbl)
        n1137 = property on="R Scan Length SP steps" class="DigNum (strict)"("Minimum"=w2317) -> ()  [unwired: 2 in, 2 out]
        n1138 = property on="R Scan Length SP steps" class="DigNum (strict)"("Maximum"=w2318) -> ()  [unwired: 2 in, 2 out]
        n1139 = property on="Y Scan Length SP steps" class="DigNum (strict)"("Minimum"=w2346) -> ()  [unwired: 2 in, 2 out]
        n1140 = property on="Y Scan Length SP steps" class="DigNum (strict)"("Maximum"=w2343) -> ()  [unwired: 2 in, 2 out]
        n1141 = property on="X Scan Length SP steps" class="DigNum (strict)"("Minimum"=w2357) -> ()  [unwired: 2 in, 2 out]
        n1142 = property on="X Scan Length SP steps" class="DigNum (strict)"("Maximum"=w2354) -> ()  [unwired: 2 in, 2 out]
        n1143 = property on="Z Scan Length SP steps" class="DigNum (strict)"("Minimum"=w2333) -> ()  [unwired: 2 in, 2 out]
        n1144 = property on="Z Scan Length SP steps" class="DigNum (strict)"("Maximum"=w2330) -> ()  [unwired: 2 in, 2 out]
        n1145 = property on="X steps/rev" class="DigNum (strict)"() -> ("Value"=w2352:u32)  [unwired: 2 in, 2 out]
        n1146 = property on="X Scan Length SP steps" class="DigNum (strict)"() -> ("Value"=w2349:i32)  [unwired: 2 in, 2 out]
        n1147 = property on="X Scan Velocity SP steps/sec" class="DigNum (strict)"() -> ("Value"=w2353:i32)  [unwired: 2 in, 2 out]
        n1148 = property on="Y steps/rev" class="DigNum (strict)"() -> ("Value"=w2340:u32)  [unwired: 2 in, 2 out]
        n1149 = property on="R Scan Length SP steps" class="DigNum (strict)"() -> ("Value"=w2314:i32)  [unwired: 2 in, 2 out]
        n1150 = property on="R steps/rev" class="DigNum (strict)"() -> ("Value"=w2313:u32)  [unwired: 2 in, 2 out]
        n1151 = property on="R Scan Velocity SP steps/sec" class="DigNum (strict)"() -> ("Value"=w2309:i32)  [unwired: 2 in, 2 out]
        n1152 = property on="Y Scan Length SP steps" class="DigNum (strict)"() -> ("Value"=w2341:i32)  [unwired: 2 in, 2 out]
        n1153 = property on="Y Scan Velocity SP steps/sec" class="DigNum (strict)"() -> ("Value"=w2337:i32)  [unwired: 2 in, 2 out]
        n1154 = property on="Z Scan Length SP steps" class="DigNum (strict)"() -> ("Value"=w2328:i32)  [unwired: 2 in, 2 out]
        n1155 = property on="Z steps/rev" class="DigNum (strict)"() -> ("Value"=w2327:u32)  [unwired: 2 in, 2 out]
        n1156 = property on="Z Scan Velocity SP steps/sec" class="DigNum (strict)"() -> ("Value"=w2323:i32)  [unwired: 2 in, 2 out]
        n1157 = To Double Precision Float(number=w2349) -> (double precision float=w2292:dbl)
        n1158 = To Double Precision Float(number=w2352) -> (double precision float=w2350:dbl)
        n1159 = To Double Precision Float(number=w2353) -> (double precision float=w2291:dbl)
        n1160 = To Double Precision Float(number=w2314) -> (double precision float=w2299:dbl)
        n1161 = To Double Precision Float(number=w2313) -> (double precision float=w2310:dbl)
        n1162 = To Double Precision Float(number=w2309) -> (double precision float=w2298:dbl)
        n1163 = To Double Precision Float(number=w2328) -> (double precision float=w2301:dbl)
        n1164 = To Double Precision Float(number=w2327) -> (double precision float=w2324:dbl)
        n1165 = To Double Precision Float(number=w2323) -> (double precision float=w2300:dbl)
        n1166 = To Double Precision Float(number=w2341) -> (double precision float=w2294:dbl)
        n1167 = To Double Precision Float(number=w2340) -> (double precision float=w2295:dbl)
        n1168 = To Double Precision Float(number=w2337) -> (double precision float=w2293:dbl)
        n1169 = property on="R deg/rev" class="DigNum (strict)"() -> ("Value"=w2312:dbl)  [unwired: 2 in, 2 out]
        n1170 = Divide(x=w2299, y=w2310) -> (x/y=w2315:dbl)
        n1171 = property on="Z mm/rev" class="DigNum (strict)"() -> ("Value"=w2326:dbl)  [unwired: 2 in, 2 out]
        n1172 = property on="X mm/rev" class="DigNum (strict)"() -> ("Value"=w2278:dbl)  [unwired: 2 in, 2 out]
        n1173 = Divide(x=w2292, y=w2350) -> (x/y=w2279:dbl)
        n1174 = Divide(x=w2301, y=w2324) -> (x/y=w2329:dbl)
        n1175 = property on="Y mm/rev" class="DigNum (strict)"() -> ("Value"=w2339:dbl)  [unwired: 2 in, 2 out]
        n1176 = Divide(x=w2294, y=w2295) -> (x/y=w2342:dbl)
        n1177 = Divide(x=w2300, y=w2324) -> (x/y=w2322:dbl)
        n1178 = Divide(x=w2298, y=w2310) -> (x/y=w2308:dbl)
        n1179 = Multiply(x=w2329, y=w2326) -> (x*y=w2321:dbl)
        n1180 = Divide(x=w2293, y=w2295) -> (x/y=w2336:dbl)
        n1181 = Divide(x=w2291, y=w2350) -> (x/y=w2277:dbl)
        n1182 = Multiply(x=w2279, y=w2278) -> (x*y=w2347:dbl)
        n1183 = Divide(x=w2301, y=w2300) -> (x/y=w2296:dbl)
        n1184 = Multiply(x=w2326, y=w2322) -> (x*y=w2320:dbl)
        n1185 = Absolute Value(x=w2296) -> (abs(x)=→"Z Scan Duration":dbl)
        n1186 = Multiply(x=w2342, y=w2339) -> (x*y=w2335:dbl)
        n1187 = Multiply(x=w2339, y=w2336) -> (x*y=w2334:dbl)
        n1188 = Multiply(x=w2278, y=w2277) -> (x*y=w2348:dbl)
        n1189 = Divide(x=w2299, y=w2298) -> (x/y=w2297:dbl)
        n1190 = Multiply(x=w2315, y=w2312) -> (x*y=w2307:dbl)
        n1191 = Multiply(x=w2312, y=w2308) -> (x*y=w2306:dbl)
        n1192 = Absolute Value(x=w2297) -> (abs(x)=→"R Scan Duration":dbl)
        n1193 = Absolute Value(x=w2306) -> (abs(x)=w2290:dbl)
        n1194 = property on="Z Scan length MV mm" class="DigNum (strict)"("Value"=w2321) -> ()  [unwired: 2 in, 2 out]
        n1195 = property on="Z Scan velocity MV mm/sec" class="DigNum (strict)"("Val(Sgnl)"=w2320) -> ()  [unwired: 2 in, 2 out]
        n1196 = property on="X Scan length MV mm" class="DigNum (strict)"("Val(Sgnl)"=w2347) -> ()  [unwired: 2 in, 2 out]
        n1197 = property on="X Scan velocity MV mm/sec" class="DigNum (strict)"("Value"=w2348) -> ()  [unwired: 2 in, 2 out]
        n1198 = property on="Y Scan length MV mm" class="DigNum (strict)"("Value"=w2335) -> ()  [unwired: 2 in, 2 out]
        n1199 = property on="Y Scan velocity MV mm/sec" class="DigNum (strict)"("Val(Sgnl)"=w2334) -> ()  [unwired: 2 in, 2 out]
        n1200 = property on="R Scan length MV deg" class="DigNum (strict)"("Value"=w2307) -> ()  [unwired: 2 in, 2 out]
        n1201 = property on="R Scan Velocity SP deg/sec" class="DigNum (strict)"("Val(Sgnl)"=w2290) -> ()  [unwired: 2 in, 2 out]
        n1202 = property on="Y Scan Length SP mm" class="DigNum (strict)"() -> ("Value"=w2274:dbl)  [unwired: 2 in, 2 out]
        n1203 = property on="X Scan Length SP mm" class="DigNum (strict)"() -> ("Value"=w2273:dbl)  [unwired: 2 in, 2 out]
        n1204 = Equal?(x=w2274, y=0.0) -> (x = y?=w2272:bool)
        n1205 = Equal?(x=w2273, y=0.0) -> (x = y?=w2271:bool)
        n1206 = case shown="True" w2272 {
          tunnel: w2294 -> [w2366 _]
          tunnel: w2293 -> [w2365 _]
          frame #0 {
            n1207 = Divide(x=w2366, y=w2365) -> (x/y=w2364:dbl)
            n1208 = Absolute Value(x=w2364) -> (abs(x)=→"Y Scan Duration":dbl)
          }
          frame #1 {
            n1209 = local write "Y Scan Duration"(0.0 ("Y Scan Duration")) -> ()
          }
        }
        n1210 = case shown="True" w2271 {
          tunnel: w2292 -> [w2360 _]
          tunnel: w2291 -> [w2359 _]
          frame #0 {
            n1211 = Divide(x=w2360, y=w2359) -> (x/y=w2361:dbl)
            n1212 = Absolute Value(x=w2361) -> (abs(x)=→"X Scan Duration":dbl)
          }
          frame #1 {
            n1213 = local write "X Scan Duration"(0.0 ("X Scan Duration")) -> ()
          }
        }
      }
      event #8 {
        n1214 = event-data() -> ()  [unwired: 1 in, 7 out]
        n1215 = Wait (ms)(milliseconds to wait=u32 100) -> ()  [unwired: 1 out]
        n1216 = local write "STATUS"("SETTING Y" ("STATUS")) -> ()
        n1217 = property on="Y Position SP mm" class="DigNum (strict)"() -> ("Value"=w2391:dbl)  [unwired: 2 in, 2 out]
        n1218 = property on="Y offset mm" class="DigNum (strict)"() -> ("Value"=w2392:dbl)  [unwired: 2 in, 2 out]
        n1219 = property on="Y mm/rev" class="DigNum (strict)"() -> ("Value"=w2378:dbl)  [unwired: 2 in, 2 out]
        n1220 = property on="Y Velocity SP mm/sec" class="DigNum (strict)"() -> ("Value"=w2385:dbl)  [unwired: 2 in, 2 out]
        n1221 = property on="Y steps/rev" class="DigNum (strict)"() -> ("Value"=w2394:u32)  [unwired: 2 in, 2 out]
        n1222 = Subtract(x=w2391, y=w2392) -> (x-y=w2395:dbl)
        n1223 = Divide(x=w2385, y=w2378) -> (x/y=w2386:dbl)
        n1224 = To Double Precision Float(number=w2394) -> (double precision float=w2379:dbl)
        n1225 = Divide(x=w2395, y=w2378) -> (x/y=w2396:dbl)
        n1226 = Multiply(x=w2386, y=w2379) -> (x*y=w2383:dbl)
        n1227 = property on="Y Velocity SP step/sec" class="DigNum (strict)"() -> ("Maximum"=w2381:dbl)  [unwired: 2 in, 2 out]
        n1228 = property on="Y Velocity SP step/sec" class="DigNum (strict)"() -> ("Minimum"=w2380:dbl)  [unwired: 2 in, 2 out]
        n1229 = Multiply(x=w2396, y=w2379) -> (x*y=w2390:dbl)
        n1230 = In Range and Coerce(upper limit=w2381, x=w2383, lower limit=w2380) -> (coerced(x)=w2382:dbl)  [unwired: 1 out]
        n1231 = property on="Y Step SP" class="DigNum (strict)"() -> ("Maximum"=w2388:dbl)  [unwired: 2 in, 2 out]
        n1232 = property on="Y Step SP" class="DigNum (strict)"() -> ("Minimum"=w2387:dbl)  [unwired: 2 in, 2 out]
        n1233 = To Long Integer(number=w2382) -> (32bit integer=w2384:i32)
        n1234 = property on="Y Velocity SP step/sec" class="DigNum (strict)"("Val(Sgnl)"=w2384) -> ()  [unwired: 2 in, 2 out]
        n1235 = In Range and Coerce(upper limit=w2388, x=w2390, lower limit=w2387) -> (coerced(x)=w2389:dbl)  [unwired: 1 out]
        n1236 = To Long Integer(number=w2389) -> (32bit integer=w2393:i32)
        n1237 = property on="Y Step SP" class="DigNum (strict)"("Val(Sgnl)"=w2393) -> ()  [unwired: 2 in, 2 out]
      }
      event #9 {
        n1238 = event-data() -> ()  [unwired: 1 in, 7 out]
        n1239 = Wait (ms)(milliseconds to wait=u32 100) -> ()  [unwired: 1 out]
        n1240 = property on="X Position SP mm" class="DigNum (strict)"() -> ("Value"=w2420:dbl)  [unwired: 2 in, 2 out]
        n1241 = property on="X offset mm" class="DigNum (strict)"() -> ("Value"=w2421:dbl)  [unwired: 2 in, 2 out]
        n1242 = property on="X steps/rev" class="DigNum (strict)"() -> ("Value"=w2423:u32)  [unwired: 2 in, 2 out]
        n1243 = property on="X Velocity SP mm/sec" class="DigNum (strict)"() -> ("Value"=w2414:dbl)  [unwired: 2 in, 2 out]
        n1244 = property on="X mm/rev" class="DigNum (strict)"() -> ("Value"=w2407:dbl)  [unwired: 2 in, 2 out]
        n1245 = Subtract(x=w2420, y=w2421) -> (x-y=w2424:dbl)
        n1246 = Divide(x=w2414, y=w2407) -> (x/y=w2415:dbl)
        n1247 = To Double Precision Float(number=w2423) -> (double precision float=w2408:dbl)
        n1248 = local write "STATUS"("SETTING X" ("STATUS")) -> ()
        n1249 = Divide(x=w2424, y=w2407) -> (x/y=w2425:dbl)
        n1250 = Multiply(x=w2415, y=w2408) -> (x*y=w2412:dbl)
        n1251 = property on="X Velocity SP step/sec" class="DigNum (strict)"() -> ("Maximum"=w2410:dbl)  [unwired: 2 in, 2 out]
        n1252 = property on="X Velocity SP step/sec" class="DigNum (strict)"() -> ("Minimum"=w2409:dbl)  [unwired: 2 in, 2 out]
        n1253 = Multiply(x=w2425, y=w2408) -> (x*y=w2419:dbl)
        n1254 = property on="X Step SP" class="DigNum (strict)"() -> ("Maximum"=w2417:dbl)  [unwired: 2 in, 2 out]
        n1255 = property on="X Step SP" class="DigNum (strict)"() -> ("Minimum"=w2416:dbl)  [unwired: 2 in, 2 out]
        n1256 = In Range and Coerce(upper limit=w2410, x=w2412, lower limit=w2409) -> (coerced(x)=w2411:dbl)  [unwired: 1 out]
        n1257 = To Long Integer(number=w2411) -> (32bit integer=w2413:i32)
        n1258 = In Range and Coerce(upper limit=w2417, x=w2419, lower limit=w2416) -> (coerced(x)=w2418:dbl)  [unwired: 1 out]
        n1259 = property on="X Velocity SP step/sec" class="DigNum (strict)"("Val(Sgnl)"=w2413) -> ()  [unwired: 2 in, 2 out]
        n1260 = To Long Integer(number=w2418) -> (32bit integer=w2422:i32)
        n1261 = property on="X Step SP" class="DigNum (strict)"("Val(Sgnl)"=w2422) -> ()  [unwired: 2 in, 2 out]
      }
      event #10 {
        n1262 = event-data() -> ()  [unwired: 1 in, 7 out]
        n1263 = Wait (ms)(milliseconds to wait=u32 100) -> ()  [unwired: 1 out]
        n1264 = property on="Z mm/rev" class="DigNum (strict)"() -> ("Value"=w2453:dbl)  [unwired: 2 in, 2 out]
        n1265 = property on="Z steps/rev" class="DigNum (strict)"() -> ("Value"=w2450:u32)  [unwired: 2 in, 2 out]
        n1266 = property on="Z Velocity SP mm/sec" class="DigNum (strict)"() -> ("Value"=w2441:dbl)  [unwired: 2 in, 2 out]
        n1267 = property on="Z Position SP mm" class="DigNum (strict)"() -> ("Value"=w2447:dbl)  [unwired: 2 in, 2 out]
        n1268 = property on="Z offset mm" class="DigNum (strict)"() -> ("Value"=w2448:dbl)  [unwired: 2 in, 2 out]
        n1269 = Divide(x=w2441, y=w2453) -> (x/y=w2442:dbl)
        n1270 = To Double Precision Float(number=w2450) -> (double precision float=w2454:dbl)
        n1271 = Subtract(x=w2447, y=w2448) -> (x-y=w2451:dbl)
        n1272 = Divide(x=w2451, y=w2453) -> (x/y=w2452:dbl)
        n1273 = Multiply(x=w2442, y=w2454) -> (x*y=w2439:dbl)
        n1274 = property on="Z Velocity SP step/sec" class="DigNum (strict)"() -> ("Maximum"=w2437:dbl)  [unwired: 2 in, 2 out]
        n1275 = property on="Z Velocity SP step/sec" class="DigNum (strict)"() -> ("Minimum"=w2436:dbl)  [unwired: 2 in, 2 out]
        n1276 = local write "STATUS"("SETTING Z" ("STATUS")) -> ()
        n1277 = Multiply(x=w2452, y=w2454) -> (x*y=w2446:dbl)
        n1278 = In Range and Coerce(upper limit=w2437, x=w2439, lower limit=w2436) -> (coerced(x)=w2438:dbl)  [unwired: 1 out]
        n1279 = property on="Z Step SP" class="DigNum (strict)"() -> ("Maximum"=w2444:dbl)  [unwired: 2 in, 2 out]
        n1280 = property on="Z Step SP" class="DigNum (strict)"() -> ("Minimum"=w2443:dbl)  [unwired: 2 in, 2 out]
        n1281 = To Long Integer(number=w2438) -> (32bit integer=w2440:i32)
        n1282 = property on="Z Velocity SP step/sec" class="DigNum (strict)"("Val(Sgnl)"=w2440) -> ()  [unwired: 2 in, 2 out]
        n1283 = In Range and Coerce(upper limit=w2444, x=w2446, lower limit=w2443) -> (coerced(x)=w2445:dbl)  [unwired: 1 out]
        n1284 = To Long Integer(number=w2445) -> (32bit integer=w2449:i32)
        n1285 = property on="Z Step SP" class="DigNum (strict)"("Val(Sgnl)"=w2449) -> ()  [unwired: 2 in, 2 out]
      }
      event #11 {
        n1286 = event-data() -> ()  [unwired: 1 in, 7 out]
        n1287 = property on="R offset deg" class="DigNum (strict)"() -> ("Value"=w2480:dbl)  [unwired: 2 in, 2 out]
        n1288 = property on="R Position SP deg" class="DigNum (strict)"() -> ("Value"=w2479:dbl)  [unwired: 2 in, 2 out]
        n1289 = Wait (ms)(milliseconds to wait=u32 100) -> ()  [unwired: 1 out]
        n1290 = Subtract(x=w2479, y=w2480) -> (x-y=w2483:dbl)
        n1291 = property on="R deg/rev" class="DigNum (strict)"() -> ("Value"=w2466:dbl)  [unwired: 2 in, 2 out]
        n1292 = property on="R Velocity SP deg/sec" class="DigNum (strict)"() -> ("Value"=w2473:dbl)  [unwired: 2 in, 2 out]
        n1293 = Divide(x=w2483, y=w2466) -> (x/y=w2484:dbl)
        n1294 = property on="R steps/rev" class="DigNum (strict)"() -> ("Value"=w2482:u32)  [unwired: 2 in, 2 out]
        n1295 = Divide(x=w2473, y=w2466) -> (x/y=w2474:dbl)
        n1296 = To Double Precision Float(number=w2482) -> (double precision float=w2467:dbl)
        n1297 = Multiply(x=w2474, y=w2467) -> (x*y=w2471:dbl)
        n1298 = Multiply(x=w2484, y=w2467) -> (x*y=w2478:dbl)
        n1299 = property on="R Velocity SP step/sec" class="DigNum (strict)"() -> ("Maximum"=w2469:dbl)  [unwired: 2 in, 2 out]
        n1300 = property on="R Step SP" class="DigNum (strict)"() -> ("Maximum"=w2476:dbl)  [unwired: 2 in, 2 out]
        n1301 = property on="R Step SP" class="DigNum (strict)"() -> ("Minimum"=w2475:dbl)  [unwired: 2 in, 2 out]
        n1302 = property on="R Velocity SP step/sec" class="DigNum (strict)"() -> ("Minimum"=w2468:dbl)  [unwired: 2 in, 2 out]
        n1303 = Absolute Value(x=w2471) -> (abs(x)=w2465:dbl)
        n1304 = In Range and Coerce(upper limit=w2476, x=w2478, lower limit=w2475) -> (coerced(x)=w2477:dbl)  [unwired: 1 out]
        n1305 = In Range and Coerce(upper limit=w2469, x=w2465, lower limit=w2468) -> (coerced(x)=w2470:dbl)  [unwired: 1 out]
        n1306 = To Long Integer(number=w2477) -> (32bit integer=w2481:i32)
        n1307 = To Long Integer(number=w2470) -> (32bit integer=w2472:i32)
        n1308 = local write "STATUS"("SETTING R" ("STATUS")) -> ()
        n1309 = property on="R Step SP" class="DigNum (strict)"("Val(Sgnl)"=w2481) -> ()  [unwired: 2 in, 2 out]
        n1310 = property on="R Velocity SP step/sec" class="DigNum (strict)"("Val(Sgnl)"=w2472) -> ()  [unwired: 2 in, 2 out]
      }
      event #12 {
        n1311 = event-data() -> ()  [unwired: 1 in, 5 out]
        n1312 = flat-sequence {
          frame #0 {
            n1313 = property on="Y mm/rev" class="DigNum (strict)"() -> ("Value"=w2494:dbl)  [unwired: 2 in, 2 out]
            n1314 = property on="Z mm/rev" class="DigNum (strict)"() -> ("Value"=w2546:dbl)  [unwired: 2 in, 2 out]
            n1315 = property on="Z Scan Length SP mm" class="DigNum (strict)"() -> ("Value"=w2559:dbl)  [unwired: 2 in, 2 out]
            n1316 = property on="Y Scan Length SP mm" class="DigNum (strict)"() -> ("Value"=w2507:dbl)  [unwired: 2 in, 2 out]
            n1317 = property on="Y steps/rev" class="DigNum (strict)"() -> ("Value"=w2509:u32)  [unwired: 2 in, 2 out]
            n1318 = Divide(x=w2559, y=w2546) -> (x/y=w2562:dbl)
            n1319 = Divide(x=w2507, y=w2494) -> (x/y=w2510:dbl)
            n1320 = property on="Z steps/rev" class="DigNum (strict)"() -> ("Value"=w2561:u32)  [unwired: 2 in, 2 out]
            n1321 = To Double Precision Float(number=w2509) -> (double precision float=w2495:dbl)
            n1322 = To Double Precision Float(number=w2561) -> (double precision float=w2547:dbl)
            n1323 = Multiply(x=w2510, y=w2495) -> (x*y=w2506:dbl)
            n1324 = property on="Y Step SP" class="DigNum (strict)"() -> ("Minimum"=w2504:dbl)  [unwired: 2 in, 2 out]
            n1325 = property on="Y Step SP" class="DigNum (strict)"() -> ("Maximum"=w2503:dbl)  [unwired: 2 in, 2 out]
            n1326 = property on="Z Step SP" class="DigNum (strict)"() -> ("Maximum"=w2555:dbl)  [unwired: 2 in, 2 out]
            n1327 = property on="Z Step SP" class="DigNum (strict)"() -> ("Minimum"=w2556:dbl)  [unwired: 2 in, 2 out]
            n1328 = Multiply(x=w2562, y=w2547) -> (x*y=w2558:dbl)
            n1329 = In Range and Coerce(upper limit=w2503, x=w2506, lower limit=w2504) -> (coerced(x)=w2505:dbl)  [unwired: 1 out]
            n1330 = In Range and Coerce(upper limit=w2555, x=w2558, lower limit=w2556) -> (coerced(x)=w2557:dbl)  [unwired: 1 out]
            n1331 = To Long Integer(number=w2505) -> (32bit integer=w2508:i32)
            n1332 = property on="Y Scan Velocity SP mm/sec" class="DigNum (strict)"() -> ("Value"=w2501:dbl)  [unwired: 2 in, 2 out]
            n1333 = property on="Z Scan Velocity SP mm/sec" class="DigNum (strict)"() -> ("Value"=w2553:dbl)  [unwired: 2 in, 2 out]
            n1334 = To Long Integer(number=w2557) -> (32bit integer=w2560:i32)
            n1335 = Divide(x=w2501, y=w2494) -> (x/y=w2502:dbl)
            n1336 = property on="Y Scan Length SP steps" class="DigNum (strict)"("Val(Sgnl)"=w2508) -> ()  [unwired: 2 in, 2 out]
            n1337 = property on="Y Scan Velocity SP steps/sec" class="DigNum (strict)"() -> ("Maximum"=w2497:dbl)  [unwired: 2 in, 2 out]
            n1338 = property on="Z Scan Velocity SP steps/sec" class="DigNum (strict)"() -> ("Maximum"=w2549:dbl)  [unwired: 2 in, 2 out]
            n1339 = Divide(x=w2553, y=w2546) -> (x/y=w2554:dbl)
            n1340 = property on="Y Scan Velocity SP steps/sec" class="DigNum (strict)"() -> ("Minimum"=w2496:dbl)  [unwired: 2 in, 2 out]
            n1341 = property on="Z Scan Length SP steps" class="DigNum (strict)"("Val(Sgnl)"=w2560) -> ()  [unwired: 2 in, 2 out]
            n1342 = property on="Z Scan Velocity SP steps/sec" class="DigNum (strict)"() -> ("Minimum"=w2548:dbl)  [unwired: 2 in, 2 out]
            n1343 = Multiply(x=w2502, y=w2495) -> (x*y=w2499:dbl)
            n1344 = Multiply(x=w2554, y=w2547) -> (x*y=w2551:dbl)
            n1345 = In Range and Coerce(upper limit=w2497, x=w2499, lower limit=w2496) -> (coerced(x)=w2498:dbl)  [unwired: 1 out]
            n1346 = In Range and Coerce(upper limit=w2549, x=w2551, lower limit=w2548) -> (coerced(x)=w2550:dbl)  [unwired: 1 out]
            n1347 = To Long Integer(number=w2498) -> (32bit integer=w2500:i32)
            n1348 = To Long Integer(number=w2550) -> (32bit integer=w2552:i32)
            n1349 = property on="Y Scan Velocity SP steps/sec" class="DigNum (strict)"("Val(Sgnl)"=w2500) -> ()  [unwired: 2 in, 2 out]
            n1350 = property on="Z Scan Velocity SP steps/sec" class="DigNum (strict)"("Val(Sgnl)"=w2552) -> ()  [unwired: 2 in, 2 out]
            n1351 = property on="X mm/rev" class="DigNum (strict)"() -> ("Value"=w2529:dbl)  [unwired: 2 in, 2 out]
            n1352 = property on="X Scan Length SP mm" class="DigNum (strict)"() -> ("Value"=w2542:dbl)  [unwired: 2 in, 2 out]
            n1353 = property on="R deg/rev" class="DigNum (strict)"() -> ("Value"=w2512:dbl)  [unwired: 2 in, 2 out]
            n1354 = property on="R Scan Length SP deg" class="DigNum (strict)"() -> ("Value"=w2525:dbl)  [unwired: 2 in, 2 out]
            n1355 = Divide(x=w2525, y=w2512) -> (x/y=w2528:dbl)
            n1356 = Divide(x=w2542, y=w2529) -> (x/y=w2545:dbl)
            n1357 = property on="X steps/rev" class="DigNum (strict)"() -> ("Value"=w2544:u32)  [unwired: 2 in, 2 out]
            n1358 = property on="R steps/rev" class="DigNum (strict)"() -> ("Value"=w2527:u32)  [unwired: 2 in, 2 out]
            n1359 = To Double Precision Float(number=w2544) -> (double precision float=w2530:dbl)
            n1360 = To Double Precision Float(number=w2527) -> (double precision float=w2513:dbl)
            n1361 = property on="X Step SP" class="DigNum (strict)"() -> ("Minimum"=w2539:dbl)  [unwired: 2 in, 2 out]
            n1362 = property on="X Step SP" class="DigNum (strict)"() -> ("Maximum"=w2538:dbl)  [unwired: 2 in, 2 out]
            n1363 = Multiply(x=w2545, y=w2530) -> (x*y=w2541:dbl)
            n1364 = In Range and Coerce(upper limit=w2538, x=w2541, lower limit=w2539) -> (coerced(x)=w2540:dbl)  [unwired: 1 out]
            n1365 = property on="R Step SP" class="DigNum (strict)"() -> ("Maximum"=w2521:dbl)  [unwired: 2 in, 2 out]
            n1366 = property on="R Step SP" class="DigNum (strict)"() -> ("Minimum"=w2522:dbl)  [unwired: 2 in, 2 out]
            n1367 = Multiply(x=w2528, y=w2513) -> (x*y=w2524:dbl)
            n1368 = property on="X Scan Velocity SP mm/sec" class="DigNum (strict)"() -> ("Value"=w2536:dbl)  [unwired: 2 in, 2 out]
            n1369 = property on="R Scan Velocity SP deg/sec" class="DigNum (strict)"() -> ("Value"=w2519:dbl)  [unwired: 2 in, 2 out]
            n1370 = To Long Integer(number=w2540) -> (32bit integer=w2543:i32)
            n1371 = Divide(x=w2536, y=w2529) -> (x/y=w2537:dbl)
            n1372 = property on="X Scan Velocity SP steps/sec" class="DigNum (strict)"() -> ("Maximum"=w2532:dbl)  [unwired: 2 in, 2 out]
            n1373 = property on="X Scan Velocity SP steps/sec" class="DigNum (strict)"() -> ("Minimum"=w2531:dbl)  [unwired: 2 in, 2 out]
            n1374 = In Range and Coerce(upper limit=w2521, x=w2524, lower limit=w2522) -> (coerced(x)=w2523:dbl)  [unwired: 1 out]
            n1375 = Divide(x=w2519, y=w2512) -> (x/y=w2520:dbl)
            n1376 = property on="X Scan Length SP steps" class="DigNum (strict)"("Val(Sgnl)"=w2543) -> ()  [unwired: 2 in, 2 out]
            n1377 = Multiply(x=w2537, y=w2530) -> (x*y=w2534:dbl)
            n1378 = Multiply(x=w2520, y=w2513) -> (x*y=w2517:dbl)
            n1379 = To Long Integer(number=w2523) -> (32bit integer=w2526:i32)
            n1380 = property on="R Velocity SP step/sec" class="DigNum (strict)"() -> ("Maximum"=w2515:dbl)  [unwired: 2 in, 2 out]
            n1381 = property on="R Scan Velocity SP steps/sec" class="DigNum (strict)"() -> ("Minimum"=w2514:dbl)  [unwired: 2 in, 2 out]
            n1382 = Absolute Value(x=w2517) -> (abs(x)=w2511:dbl)
            n1383 = property on="R Scan Length SP steps" class="DigNum (strict)"("Val(Sgnl)"=w2526) -> ()  [unwired: 2 in, 2 out]
            n1384 = In Range and Coerce(upper limit=w2532, x=w2534, lower limit=w2531) -> (coerced(x)=w2533:dbl)  [unwired: 1 out]
            n1385 = In Range and Coerce(upper limit=w2515, x=w2511, lower limit=w2514) -> (coerced(x)=w2516:dbl)  [unwired: 1 out]
            n1386 = To Long Integer(number=w2533) -> (32bit integer=w2535:i32)
            n1387 = To Long Integer(number=w2516) -> (32bit integer=w2518:i32)
            n1388 = property on="X Scan Velocity SP steps/sec" class="DigNum (strict)"("Val(Sgnl)"=w2535) -> ()  [unwired: 2 in, 2 out]
            n1389 = property on="R Scan Velocity SP steps/sec" class="DigNum (strict)"("Val(Sgnl)"=w2518) -> ()  [unwired: 2 in, 2 out]
          }
          frame #1 {
            n1390 = case shown="True" "Z as dominating length" {
              frame #0 {
              }
              frame #1 {
                n1391 = property on="Y Scan Length SP steps" class="DigNum (strict)"() -> ("Value"=w2572:i32)  [unwired: 2 in, 2 out]
                n1392 = property on="Z Scan Length SP steps" class="DigNum (strict)"() -> ("Value"=w2571:i32)  [unwired: 2 in, 2 out]
                n1393 = property on="Y Scan Velocity SP steps/sec" class="DigNum (strict)"() -> ("Value"=w2568:i32)  [unwired: 2 in, 2 out]
                n1394 = property on="X Scan Length SP steps" class="DigNum (strict)"() -> ("Value"=w2580:i32)  [unwired: 2 in, 2 out]
                n1395 = property on="Z Scan Length SP steps" class="DigNum (strict)"() -> ("Value"=w2579:i32)  [unwired: 2 in, 2 out]
                n1396 = property on="X Scan Velocity SP steps/sec" class="DigNum (strict)"() -> ("Value"=w2578:i32)  [unwired: 2 in, 2 out]
                n1397 = To Double Precision Float(number=w2572) -> (double precision float=w2570:dbl)
                n1398 = To Double Precision Float(number=w2571) -> (double precision float=w2569:dbl)
                n1399 = To Double Precision Float(number=w2568) -> (double precision float=w2567:dbl)
                n1400 = To Double Precision Float(number=w2580) -> (double precision float=w2574:dbl)
                n1401 = To Double Precision Float(number=w2579) -> (double precision float=w2575:dbl)
                n1402 = To Double Precision Float(number=w2578) -> (double precision float=w2576:dbl)
                n1403 = Divide(x=w2570, y=w2569) -> (x/y=w2564:dbl)
                n1404 = Divide(x=w2574, y=w2575) -> (x/y=w2581:dbl)
                n1405 = Multiply(x=w2564, y=w2567) -> (x*y=w2566:dbl)
                n1406 = Multiply(x=w2581, y=w2576) -> (x*y=w2577:dbl)
                n1407 = To Long Integer(number=w2566) -> (32bit integer=w2565:i32)
                n1408 = To Long Integer(number=w2577) -> (32bit integer=w2573:i32)
                n1409 = property on="Y Scan Velocity SP steps/sec" class="DigNum (strict)"("Val(Sgnl)"=w2565) -> ()  [unwired: 2 in, 2 out]
                n1410 = property on="X Scan Velocity SP steps/sec" class="DigNum (strict)"("Val(Sgnl)"=w2573) -> ()  [unwired: 2 in, 2 out]
              }
            }
          }
          frame #2 {
          }
        }
        n1411 = local write "STATUS"("SCANNING PARAMETERS SET" ("STATUS")) -> ()
      }
      event #13 {
        n1412 = event-data() -> ()  [unwired: 1 in, 5 out]
        n1413 = property on="Nr LOOPS" class="DigNum (strict)"() -> ("Value"=w2583:i32)  [unwired: 2 in, 2 out]
        n1414 = Not Equal?(x=w2583, y=0) -> (x != y?=w2584:bool)
        n1415 = case shown="True" w2584 {
          selector: w2584 -> [_ w2648]
          frame #0 {
          }
          frame #1 {
            n1416 = flat-sequence {
              tunnel: [w2651] -> w2649
              tunnel: w2648 -> [w2650]
              tunnel: [w2650] -> w2647
              tunnel: w2649 -> [w2656]
              tunnel: w2647 -> [w2655]
              tunnel: [w2654] -> w2646
              frame #0 {
                n1417 = Two Button Dialog(message="DO YOU WANT TO LOOP", 2:"YES" ("T button name (\"OK\")")) -> (T button?=w2651:bool)  [unwired: 1 in]
              }
              frame #1 {
                n1418 = Equal?(x=w2656, y=w2655) -> (x = y?=w2654:bool)
                n1419 = property on="LoopScanConfirmed" class="Bool (strict)"("Val(Sgnl)"=w2654) -> ()  [unwired: 2 in, 2 out]
              }
            }
            n1420 = property on="counter" class="DigNum (strict)"("Val(Sgnl)"=0 ("Value (Signaling)")) -> ()  [unwired: 2 in, 2 out]
            n1421 = property on="Z Moved" class="Bool (strict)"("Val(Sgnl)"=FALSE ("Value (Signaling)")) -> ()  [unwired: 2 in, 2 out]
            n1422 = property on="FirstScan" class="Bool (strict)"("Val(Sgnl)"=w2646) -> ()  [unwired: 2 in, 2 out]
          }
        }
        n1423 = flat-sequence {
          tunnel: [w2748] -> w2632
          tunnel: [w2747] -> w2630
          tunnel: w2638 -> [w2750]
          tunnel: w2637 -> [w2749]
          tunnel: w2632 -> [w2756]
          tunnel: [w2756] -> w2631
          tunnel: w2630 -> [w2755]
          tunnel: [w2755] -> w2629
          tunnel: w2631 -> [w2760]
          tunnel: [w2759] -> w2634
          tunnel: w2629 -> [w2758]
          tunnel: [w2757] -> w2633
          tunnel: w2634 -> [w2768]
          tunnel: [w2768] -> w2636
          tunnel: w2633 -> [w2767]
          tunnel: [w2767] -> w2635
          tunnel: w2636 -> [w2773]
          tunnel: w2635 -> [w2772]
          tunnel: [w2773] -> w2640
          tunnel: [w2772] -> w2639
          tunnel: [w2775] -> w2641
          tunnel: [w2776] -> w2642
          tunnel: w2640 -> [w2776]
          tunnel: w2639 -> [w2775]
          frame #0 {
            n1424 = property on="X Scan Velocity SP steps/sec" class="DigNum (strict)"() -> ("Value"=w2752:i32)  [unwired: 2 in, 2 out]
            n1425 = Number To Decimal String(number=w2752) -> (decimal integer string=w2753:string)  [unwired: 1 in]
            n1426 = call "mDrive Send Command.vi"("error in (no error)"=w2750, "Extra"=w2753, "Command"=T10."Max Velocity", "VISA resource name"=w2749) -> ("error out"=w2747:errorcluster, "VISA resource name out"=w2748:refnum<visa-resource-name>)  [unwired: 3 in, 1 out]
          }
          frame #1 {
            n1427 = Wait (ms)(milliseconds to wait=u32 100) -> ()  [unwired: 1 out]
          }
          frame #2 {
            # "VELOCITY"
            n1428 = call "mDrive Send Command.vi"("error in (no error)"=w2758, "Extra"="VM", "Command"=T10."Print Parameter", "VISA resource name"=w2760) -> ("error out"=w2757:errorcluster, "read buffer"=w2763:string, "VISA resource name out"=w2759:refnum<visa-resource-name>)  [unwired: 3 in]
            n1429 = Decimal String To Number(string=w2763, offset=0) -> (number=w2761:i32)  [unwired: 1 in, 1 out]
            n1430 = property on="X velocity PV step/sec" class="DigNum (strict)"("Val(Sgnl)"=w2761) -> ()  [unwired: 2 in, 2 out]
          }
          frame #3 {
            n1431 = Wait (ms)(milliseconds to wait=u32 100) -> ()  [unwired: 1 out]
          }
          frame #4 {
            n1432 = property on="X Scan Velocity SP steps/sec" class="DigNum (strict)"("DisabledEnum"=T1."Disabled and Grayed Out" ("Disabled")) -> ()  [unwired: 2 in, 2 out]
            n1433 = property on="X Scan Length SP steps" class="DigNum (strict)"("DisabledEnum"=T1."Disabled and Grayed Out" ("Disabled")) -> ()  [unwired: 2 in, 2 out]
            n1434 = property on="Scan Go" class="Bool (strict)"("DisabledEnum"=T1."Enabled" ("Disabled")) -> ()  [unwired: 2 in, 2 out]
          }
          frame #5 {
            n1435 = property on="X Scan" class="Bool (strict)"("Val(Sgnl)"=TRUE ("Slew Ready 2")) -> ()  [unwired: 2 in, 2 out]
          }
        }
        n1436 = flat-sequence {
          tunnel: [w2690] -> w2614
          tunnel: [w2689] -> w2613
          tunnel: w2604 -> [w2688]
          tunnel: w2603 -> [w2687]
          tunnel: w2614 -> [w2696]
          tunnel: [w2696] -> w2612
          tunnel: w2613 -> [w2695]
          tunnel: [w2695] -> w2611
          tunnel: w2612 -> [w2702]
          tunnel: [w2701] -> w2610
          tunnel: w2611 -> [w2700]
          tunnel: [w2699] -> w2609
          tunnel: w2610 -> [w2708]
          tunnel: [w2708] -> w2608
          tunnel: w2609 -> [w2707]
          tunnel: [w2707] -> w2607
          tunnel: w2608 -> [w2713]
          tunnel: w2607 -> [w2712]
          tunnel: [w2713] -> w2606
          tunnel: [w2712] -> w2605
          tunnel: [w2715] -> w2601
          tunnel: [w2716] -> w2602
          tunnel: w2606 -> [w2716]
          tunnel: w2605 -> [w2715]
          frame #0 {
            n1437 = property on="Z Scan Velocity SP steps/sec" class="DigNum (strict)"() -> ("Value"=w2692:i32)  [unwired: 2 in, 2 out]
            n1438 = Number To Decimal String(number=w2692) -> (decimal integer string=w2693:string)  [unwired: 1 in]
            n1439 = call "mDrive Send Command.vi"("error in (no error)"=w2688, "Extra"=w2693, "Command"=T10."Max Velocity", "VISA resource name"=w2687) -> ("error out"=w2689:errorcluster, "VISA resource name out"=w2690:refnum<visa-resource-name>)  [unwired: 3 in, 1 out]
          }
          frame #1 {
            n1440 = Wait (ms)(milliseconds to wait=u32 100) -> ()  [unwired: 1 out]
          }
          frame #2 {
            # "VELOCITY"
            n1441 = call "mDrive Send Command.vi"("error in (no error)"=w2700, "Extra"="VM", "Command"=T10."Print Parameter", "VISA resource name"=w2702) -> ("error out"=w2699:errorcluster, "read buffer"=w2703:string, "VISA resource name out"=w2701:refnum<visa-resource-name>)  [unwired: 3 in]
            n1442 = Decimal String To Number(string=w2703, offset=0) -> (number=w2704:i32)  [unwired: 1 in, 1 out]
            n1443 = property on="Z  velocity PV step/sec" class="DigNum (strict)"("Val(Sgnl)"=w2704) -> ()  [unwired: 2 in, 2 out]
          }
          frame #3 {
            n1444 = Wait (ms)(milliseconds to wait=u32 100) -> ()  [unwired: 1 out]
          }
          frame #4 {
            n1445 = property on="Z Scan Length SP steps" class="DigNum (strict)"("DisabledEnum"=T1."Disabled and Grayed Out" ("Disabled")) -> ()  [unwired: 2 in, 2 out]
            n1446 = property on="Z Scan Velocity SP steps/sec" class="DigNum (strict)"("DisabledEnum"=T1."Disabled and Grayed Out" ("Disabled")) -> ()  [unwired: 2 in, 2 out]
            n1447 = property on="Scan Go" class="Bool (strict)"("DisabledEnum"=T1."Enabled" ("Disabled")) -> ()  [unwired: 2 in, 2 out]
          }
          frame #5 {
            n1448 = property on="Z Scan" class="Bool (strict)"("Val(Sgnl)"=TRUE ("Slew Ready 2")) -> ()  [unwired: 2 in, 2 out]
          }
        }
        n1449 = flat-sequence {
          tunnel: [w2720] -> w2628
          tunnel: [w2719] -> w2627
          tunnel: w2617 -> [w2718]
          tunnel: w2616 -> [w2717]
          tunnel: w2628 -> [w2726]
          tunnel: [w2726] -> w2626
          tunnel: w2627 -> [w2725]
          tunnel: [w2725] -> w2625
          tunnel: w2626 -> [w2730]
          tunnel: [w2729] -> w2624
          tunnel: w2625 -> [w2728]
          tunnel: [w2727] -> w2623
          tunnel: w2624 -> [w2738]
          tunnel: [w2738] -> w2622
          tunnel: w2623 -> [w2737]
          tunnel: [w2737] -> w2621
          tunnel: w2622 -> [w2743]
          tunnel: w2621 -> [w2742]
          tunnel: [w2743] -> w2620
          tunnel: [w2742] -> w2619
          tunnel: [w2745] -> w2618
          tunnel: [w2746] -> w2615
          tunnel: w2620 -> [w2746]
          tunnel: w2619 -> [w2745]
          frame #0 {
            n1450 = property on="Y Scan Velocity SP steps/sec" class="DigNum (strict)"() -> ("Value"=w2722:i32)  [unwired: 2 in, 2 out]
            n1451 = Number To Decimal String(number=w2722) -> (decimal integer string=w2723:string)  [unwired: 1 in]
            n1452 = call "mDrive Send Command.vi"("error in (no error)"=w2718, "Extra"=w2723, "Command"=T10."Max Velocity", "VISA resource name"=w2717) -> ("error out"=w2719:errorcluster, "VISA resource name out"=w2720:refnum<visa-resource-name>)  [unwired: 3 in, 1 out]
          }
          frame #1 {
            n1453 = Wait (ms)(milliseconds to wait=u32 100) -> ()  [unwired: 1 out]
          }
          frame #2 {
            # "VELOCITY"
            n1454 = call "mDrive Send Command.vi"("error in (no error)"=w2728, "Extra"="VM", "Command"=T10."Print Parameter", "VISA resource name"=w2730) -> ("error out"=w2727:errorcluster, "read buffer"=w2734:string, "VISA resource name out"=w2729:refnum<visa-resource-name>)  [unwired: 3 in]
            n1455 = Decimal String To Number(string=w2734, offset=0) -> (number=w2732:i32)  [unwired: 1 in, 1 out]
            n1456 = property on="Y velocity PV step/sec" class="DigNum (strict)"("Val(Sgnl)"=w2732) -> ()  [unwired: 2 in, 2 out]
          }
          frame #3 {
            n1457 = Wait (ms)(milliseconds to wait=u32 100) -> ()  [unwired: 1 out]
          }
          frame #4 {
            n1458 = property on="Y Scan Velocity SP steps/sec" class="DigNum (strict)"("DisabledEnum"=T1."Disabled and Grayed Out" ("Disabled")) -> ()  [unwired: 2 in, 2 out]
            n1459 = property on="Y Scan Length SP steps" class="DigNum (strict)"("DisabledEnum"=T1."Disabled and Grayed Out" ("Disabled")) -> ()  [unwired: 2 in, 2 out]
            n1460 = property on="Scan Go" class="Bool (strict)"("DisabledEnum"=T1."Enabled" ("Disabled")) -> ()  [unwired: 2 in, 2 out]
          }
          frame #5 {
            n1461 = property on="Y Scan" class="Bool (strict)"("Val(Sgnl)"=TRUE ("Slew Ready 2")) -> ()  [unwired: 2 in, 2 out]
          }
        }
        n1462 = flat-sequence {
          tunnel: [w2660] -> w2600
          tunnel: [w2659] -> w2599
          tunnel: w2590 -> [w2658]
          tunnel: w2589 -> [w2657]
          tunnel: w2600 -> [w2666]
          tunnel: [w2666] -> w2598
          tunnel: w2599 -> [w2665]
          tunnel: [w2665] -> w2597
          tunnel: w2598 -> [w2672]
          tunnel: [w2671] -> w2596
          tunnel: w2597 -> [w2670]
          tunnel: [w2669] -> w2595
          tunnel: w2596 -> [w2678]
          tunnel: w2595 -> [w2677]
          tunnel: [w2678] -> w2594
          tunnel: [w2677] -> w2593
          tunnel: w2594 -> [w2683]
          tunnel: w2593 -> [w2682]
          tunnel: [w2683] -> w2592
          tunnel: [w2682] -> w2591
          tunnel: [w2685] -> w2587
          tunnel: [w2686] -> w2588
          tunnel: w2592 -> [w2686]
          tunnel: w2591 -> [w2685]
          frame #0 {
            n1463 = property on="R Scan Velocity SP steps/sec" class="DigNum (strict)"() -> ("Value"=w2662:i32)  [unwired: 2 in, 2 out]
            n1464 = Number To Decimal String(number=w2662) -> (decimal integer string=w2663:string)  [unwired: 1 in]
            n1465 = call "mDrive Send Command.vi"("error in (no error)"=w2658, "Extra"=w2663, "Command"=T10."Max Velocity", "VISA resource name"=w2657) -> ("error out"=w2659:errorcluster, "VISA resource name out"=w2660:refnum<visa-resource-name>)  [unwired: 3 in, 1 out]
          }
          frame #1 {
            n1466 = Wait (ms)(milliseconds to wait=u32 100) -> ()  [unwired: 1 out]
          }
          frame #2 {
            # "VELOCITY"
            n1467 = call "mDrive Send Command.vi"("error in (no error)"=w2670, "Extra"="VM", "Command"=T10."Print Parameter", "VISA resource name"=w2672) -> ("error out"=w2669:errorcluster, "read buffer"=w2674:string, "VISA resource name out"=w2671:refnum<visa-resource-name>)  [unwired: 3 in]
            n1468 = Decimal String To Number(string=w2674, offset=0) -> (number=w2673:i32)  [unwired: 1 in, 1 out]
            n1469 = property on="R velocity PV step/sec" class="DigNum (strict)"("Val(Sgnl)"=w2673) -> ()  [unwired: 2 in, 2 out]
          }
          frame #3 {
            n1470 = Wait (ms)(milliseconds to wait=u32 100) -> ()  [unwired: 1 out]
          }
          frame #4 {
            n1471 = property on="R Scan Velocity SP steps/sec" class="DigNum (strict)"("DisabledEnum"=T1."Disabled and Grayed Out" ("Disabled")) -> ()  [unwired: 2 in, 2 out]
            n1472 = property on="R Scan Length SP steps" class="DigNum (strict)"("DisabledEnum"=T1."Disabled and Grayed Out" ("Disabled")) -> ()  [unwired: 2 in, 2 out]
            n1473 = property on="Scan Go" class="Bool (strict)"("DisabledEnum"=T1."Enabled" ("Disabled")) -> ()  [unwired: 2 in, 2 out]
          }
          frame #5 {
            n1474 = property on="R Scan" class="Bool (strict)"("Val(Sgnl)"=TRUE ("Slew Ready 2")) -> ()  [unwired: 2 in, 2 out]
          }
        }
        n1475 = local write "STATUS"("READY TO SCAN" ("STATUS")) -> ()
        n1476 = property on="NewLoop" class="Bool (strict)"() -> ("Value"=w2582:bool)  [unwired: 2 in, 2 out]
        n1477 = case shown="True" w2582 {
          frame #0 {
          }
          frame #1 {
            n1478 = property on="Loop Scan" class="Bool (strict)"("Val(Sgnl)"=FALSE ("Value (Signaling)")) -> ()  [unwired: 2 in, 2 out]
          }
        }
      }
      event #14 {
        w2777 = FALSE ("Value (Signaling)")
        w2778 = FALSE ("Scan Go")
        n1479 = event-data() -> ()  [unwired: 1 in, 7 out]
        n1480 = flat-sequence {
          tunnel: [w2831] -> w2801
          tunnel: [w2830] -> w2800
          tunnel: w2789 -> [w2828]
          tunnel: w2787 -> [w2827]
          tunnel: [w2835] -> w2798
          tunnel: [w2836] -> w2799
          tunnel: w2801 -> [w2836]
          tunnel: w2800 -> [w2835]
          frame #0 {
            n1481 = call "mDrive Send Command.vi"("error in (no error)"=w2827, "Command"=T10."Stop", "VISA resource name"=w2828) -> ("error out"=w2830:errorcluster, "VISA resource name out"=w2831:refnum<visa-resource-name>)  [unwired: 4 in, 1 out]
          }
          frame #1 {
            n1482 = property on="X Scan" class="Bool (strict)"("Value"=FALSE ("Slew Ready")) -> ()  [unwired: 2 in, 2 out]
            n1483 = property on="X Scan Velocity SP steps/sec" class="DigNum (strict)"("DisabledEnum"=T1."Enabled" ("Disabled")) -> ()  [unwired: 2 in, 2 out]
            n1484 = property on="X Scan Length SP steps" class="DigNum (strict)"("DisabledEnum"=T1."Enabled" ("Disabled")) -> ()  [unwired: 2 in, 2 out]
          }
        }
        n1485 = flat-sequence {
          tunnel: [w2821] -> w2797
          tunnel: [w2820] -> w2796
          tunnel: w2788 -> [w2818]
          tunnel: w2786 -> [w2817]
          tunnel: [w2825] -> w2794
          tunnel: [w2826] -> w2795
          tunnel: w2797 -> [w2826]
          tunnel: w2796 -> [w2825]
          frame #0 {
            n1486 = call "mDrive Send Command.vi"("error in (no error)"=w2817, "Command"=T10."Stop", "VISA resource name"=w2818) -> ("error out"=w2820:errorcluster, "VISA resource name out"=w2821:refnum<visa-resource-name>)  [unwired: 4 in, 1 out]
          }
          frame #1 {
            n1487 = property on="Z Scan" class="Bool (strict)"("Value"=FALSE ("Slew Ready")) -> ()  [unwired: 2 in, 2 out]
            n1488 = property on="Z Scan Length SP steps" class="DigNum (strict)"("DisabledEnum"=T1."Enabled" ("Disabled")) -> ()  [unwired: 2 in, 2 out]
            n1489 = property on="Z Scan Velocity SP steps/sec" class="DigNum (strict)"("DisabledEnum"=T1."Enabled" ("Disabled")) -> ()  [unwired: 2 in, 2 out]
          }
        }
        n1490 = flat-sequence {
          tunnel: [w2841] -> w2803
          tunnel: [w2840] -> w2802
          tunnel: w2785 -> [w2838]
          tunnel: w2783 -> [w2837]
          tunnel: [w2845] -> w2805
          tunnel: [w2846] -> w2806
          tunnel: w2803 -> [w2846]
          tunnel: w2802 -> [w2845]
          frame #0 {
            n1491 = call "mDrive Send Command.vi"("error in (no error)"=w2837, "Command"=T10."Stop", "VISA resource name"=w2838) -> ("error out"=w2840:errorcluster, "VISA resource name out"=w2841:refnum<visa-resource-name>)  [unwired: 4 in, 1 out]
          }
          frame #1 {
            n1492 = property on="Y Scan" class="Bool (strict)"("Value"=FALSE ("Slew Ready")) -> ()  [unwired: 2 in, 2 out]
            n1493 = property on="Y Scan Velocity SP steps/sec" class="DigNum (strict)"("DisabledEnum"=T1."Enabled" ("Disabled")) -> ()  [unwired: 2 in, 2 out]
            n1494 = property on="Y Scan Length SP steps" class="DigNum (strict)"("DisabledEnum"=T1."Enabled" ("Disabled")) -> ()  [unwired: 2 in, 2 out]
          }
        }
        n1495 = flat-sequence {
          tunnel: [w2811] -> w2793
          tunnel: [w2810] -> w2792
          tunnel: w2784 -> [w2808]
          tunnel: w2782 -> [w2807]
          tunnel: [w2815] -> w2790
          tunnel: [w2816] -> w2791
          tunnel: w2793 -> [w2816]
          tunnel: w2792 -> [w2815]
          frame #0 {
            n1496 = call "mDrive Send Command.vi"("error in (no error)"=w2807, "Command"=T10."Stop", "VISA resource name"=w2808) -> ("error out"=w2810:errorcluster, "VISA resource name out"=w2811:refnum<visa-resource-name>)  [unwired: 4 in, 1 out]
          }
          frame #1 {
            n1497 = property on="R Scan" class="Bool (strict)"("Value"=FALSE ("Slew Ready")) -> ()  [unwired: 2 in, 2 out]
            n1498 = property on="R Scan Velocity SP steps/sec" class="DigNum (strict)"("DisabledEnum"=T1."Enabled" ("Disabled")) -> ()  [unwired: 2 in, 2 out]
            n1499 = property on="R Scan Length SP steps" class="DigNum (strict)"("DisabledEnum"=T1."Enabled" ("Disabled")) -> ()  [unwired: 2 in, 2 out]
          }
        }
        n1500 = property on="Set for Scan" class="Bool (strict)"("DisabledEnum"=T1."Enabled" ("Disabled")) -> ()  [unwired: 2 in, 2 out]
        n1501 = property on="Scan Go" class="Bool (strict)"("DisabledEnum"=T1."Disabled and Grayed Out" ("Disabled")) -> ()  [unwired: 2 in, 2 out]
        n1502 = property on="LoopScanConfirmed" class="Bool (strict)"("Val(Sgnl)"=w2778) -> ()  [unwired: 2 in, 2 out]
        n1503 = property on="Scan Go" class="Bool (strict)"("Val(Sgnl)"=w2778) -> ()  [unwired: 2 in, 2 out]
        n1504 = property on="Z Moved" class="Bool (strict)"("Val(Sgnl)"=w2778) -> ()  [unwired: 2 in, 2 out]
        n1505 = property on="GOBACK" class="Bool (strict)"("Val(Sgnl)"=w2778) -> ()  [unwired: 2 in, 2 out]
        n1506 = property on="GO" class="Bool"("DisabledEnum"=T1."Enabled" ("Disabled")) -> ()  [unwired: 2 in, 2 out]
        n1507 = property on="Set Scan \nParameters" class="Bool (strict)"("DisabledEnum"=T1."Enabled" ("Disabled")) -> ()  [unwired: 2 in, 2 out]
        n1508 = property on="LoopCheck" class="Bool (strict)"("Val(Sgnl)"=w2777) -> ()  [unwired: 2 in, 2 out]
        n1509 = property on="NewLoop" class="Bool (strict)"("Val(Sgnl)"=w2777) -> ()  [unwired: 2 in, 2 out]
        n1510 = property on="FirstScan" class="Bool (strict)"("Val(Sgnl)"=w2777) -> ()  [unwired: 2 in, 2 out]
      }
      event #15 {
        n1511 = event-data() -> ()  [unwired: 1 in, 7 out]
        n1512 = flat-sequence {
          tunnel: [w2930] -> w2914
          tunnel: [w2928] -> w2907
          tunnel: [w2929] -> w2904
          tunnel: [w2923] -> w2903
          tunnel: [w2927] -> w2902
          tunnel: [w2926] -> w2901
          tunnel: [w2925] -> w2900
          tunnel: [w2924] -> w2899
          tunnel: w2866 -> [w2922]
          tunnel: w2865 -> [w2921]
          tunnel: w2864 -> [w2920]
          tunnel: w2863 -> [w2919]
          tunnel: w2862 -> [w2918]
          tunnel: w2861 -> [w2917]
          tunnel: w2860 -> [w2916]
          tunnel: w2859 -> [w2915]
          tunnel: [w2922] -> w2858
          tunnel: [w2921] -> w2857
          tunnel: [w2920] -> w2856
          tunnel: [w2919] -> w2855
          tunnel: [w2918] -> w2854
          tunnel: [w2917] -> w2853
          tunnel: [w2916] -> w2852
          tunnel: [w2915] -> w2851
          tunnel: [w2982] -> w2911
          tunnel: [w2981] -> w2909
          tunnel: w2914 -> [w2980]
          tunnel: w2907 -> [w2979]
          tunnel: [w2979] -> w2905
          tunnel: w2904 -> [w2978]
          tunnel: w2903 -> [w2967]
          tunnel: w2902 -> [w2977]
          tunnel: w2901 -> [w2973]
          tunnel: w2900 -> [w2970]
          tunnel: w2899 -> [w2976]
          tunnel: [w2975] -> w2897
          tunnel: [w2974] -> w2895
          tunnel: [w2973] -> w2892
          tunnel: [w2972] -> w2890
          tunnel: [w2971] -> w2888
          tunnel: [w2970] -> w2886
          tunnel: [w2969] -> w2884
          tunnel: [w2968] -> w2882
          tunnel: [w2967] -> w2881
          tunnel: w2858 -> [w2966]
          tunnel: w2857 -> [w2965]
          tunnel: w2856 -> [w2964]
          tunnel: w2855 -> [w2963]
          tunnel: w2854 -> [w2962]
          tunnel: w2853 -> [w2961]
          tunnel: w2852 -> [w2960]
          tunnel: w2851 -> [w2959]
          tunnel: w2911 -> [w3023]
          tunnel: [w3023] -> w2910
          tunnel: w2909 -> [w3022]
          tunnel: [w3022] -> w2908
          tunnel: [w3021] -> w2906
          tunnel: w2905 -> [w3021]
          tunnel: [w3020] -> w2898
          tunnel: w2897 -> [w3020]
          tunnel: [w3019] -> w2896
          tunnel: w2895 -> [w3019]
          tunnel: [w3018] -> w2894
          tunnel: [w3017] -> w2893
          tunnel: w2892 -> [w3017]
          tunnel: [w3016] -> w2891
          tunnel: w2890 -> [w3016]
          tunnel: [w3015] -> w2889
          tunnel: w2888 -> [w3015]
          tunnel: [w3014] -> w2887
          tunnel: w2886 -> [w3014]
          tunnel: [w3013] -> w2885
          tunnel: w2884 -> [w3013]
          tunnel: [w3012] -> w2883
          tunnel: w2882 -> [w3012]
          tunnel: w2881 -> [w3018]
          tunnel: w2910 -> [w3043]
          tunnel: [w3041] -> w2913
          tunnel: w2908 -> [w3042]
          tunnel: [w3040] -> w2912
          tunnel: w2906 -> [w3039]
          tunnel: w2898 -> [w3038]
          tunnel: w2896 -> [w3037]
          tunnel: w2894 -> [w3036]
          tunnel: w2893 -> [w3035]
          tunnel: w2891 -> [w3034]
          tunnel: w2889 -> [w3033]
          tunnel: w2887 -> [w3032]
          tunnel: w2885 -> [w3031]
          tunnel: w2883 -> [w3030]
          tunnel: [w3029] -> w2880
          tunnel: [w3028] -> w2879
          tunnel: [w3027] -> w2874
          tunnel: [w3026] -> w2871
          tunnel: [w3025] -> w2869
          tunnel: [w3024] -> w2867
          tunnel: w2913 -> [w3100]
          tunnel: w2912 -> [w3099]
          tunnel: [w3100] -> w2878
          tunnel: [w3099] -> w2877
          tunnel: [w3094] -> w2876
          tunnel: w2880 -> [w3094]
          tunnel: [w3093] -> w2875
          tunnel: w2879 -> [w3093]
          tunnel: w2874 -> [w3083]
          tunnel: [w3083] -> w2873
          tunnel: [w3082] -> w2872
          tunnel: w2871 -> [w3082]
          tunnel: [w3081] -> w2870
          tunnel: w2869 -> [w3081]
          tunnel: [w3080] -> w2868
          tunnel: w2867 -> [w3080]
          frame #0 {
            n1513 = property on="X Scan" class="Bool (strict)"() -> ("Value"=w2923:bool)  [unwired: 2 in, 2 out]
            n1514 = property on="Z Scan" class="Bool (strict)"() -> ("Value"=w2925:bool)  [unwired: 2 in, 2 out]
            n1515 = property on="Y Scan" class="Bool (strict)"() -> ("Value"=w2928:bool)  [unwired: 2 in, 2 out]
            n1516 = property on="R Scan" class="Bool (strict)"() -> ("Value"=w2926:bool)  [unwired: 2 in, 2 out]
            n1517 = case shown="True" w2928 {
              tunnel: ["" w2953] -> w2930
              frame #0 {
              }
              frame #1 {
                n1518 = property on="Y Scan Length SP steps" class="DigNum (strict)"() -> ("Value"=w2958:i32)  [unwired: 2 in, 2 out]
                n1519 = Number To Decimal String(number=w2958) -> (decimal integer string=w2955:string)  [unwired: 1 in]
                n1520 = call <vilib>:"Space Constant.vi"() -> ("String"=w2956:string)
                n1521 = Concatenate Strings("MR", w2956, w2955, "\r") -> (w2953:string)
              }
            }
            n1522 = case shown="True" w2923 {
              tunnel: ["" w2946] -> w2929
              frame #0 {
              }
              frame #1 {
                n1523 = property on="X Scan Length SP steps" class="DigNum (strict)"() -> ("Value"=w2951:i32)  [unwired: 2 in, 2 out]
                n1524 = Number To Decimal String(number=w2951) -> (decimal integer string=w2948:string)  [unwired: 1 in]
                n1525 = call <vilib>:"Space Constant.vi"() -> ("String"=w2949:string)
                n1526 = Concatenate Strings("MR", w2949, w2948, "\r") -> (w2946:string)
              }
            }
            n1527 = case shown="True" w2926 {
              tunnel: ["" w2932] -> w2924
              frame #0 {
              }
              frame #1 {
                n1528 = property on="R Scan Length SP steps" class="DigNum (strict)"() -> ("Value"=w2937:i32)  [unwired: 2 in, 2 out]
                n1529 = Number To Decimal String(number=w2937) -> (decimal integer string=w2934:string)  [unwired: 1 in]
                n1530 = call <vilib>:"Space Constant.vi"() -> ("String"=w2935:string)
                n1531 = Concatenate Strings("MR", w2935, w2934, "\r") -> (w2932:string)
              }
            }
            n1532 = case shown="True" w2925 {
              tunnel: ["" w2939] -> w2927
              frame #0 {
              }
              frame #1 {
                n1533 = property on="Z Scan Length SP steps" class="DigNum (strict)"() -> ("Value"=w2944:i32)  [unwired: 2 in, 2 out]
                n1534 = Number To Decimal String(number=w2944) -> (decimal integer string=w2941:string)  [unwired: 1 in]
                n1535 = call <vilib>:"Space Constant.vi"() -> ("String"=w2942:string)
                n1536 = Concatenate Strings("MR", w2942, w2941, "\r") -> (w2939:string)
              }
            }
          }
          frame #1 {
            n1537 = case shown="True" w2967 {
              tunnel: [w2998 w3003] -> w2975
              tunnel: [w2997 w3002] -> w2974
              tunnel: w2978 -> [_ w3001]
              tunnel: w2966 -> [w2998 w3000]
              tunnel: w2965 -> [w2997 w2999]
              frame #0 {
              }
              frame #1 {
                n1538 = VISA Write(VISA resource name=w3000, write buffer=w3001, error in (no error)=w2999) -> (VISA resource name out=w3003:refnum<visa-resource-name>, error out=w3002:errorcluster)  [unwired: 1 out]
              }
            }
            n1539 = case shown="True" w2970 {
              tunnel: [w2991 w2996] -> w2969
              tunnel: [w2990 w2995] -> w2968
              tunnel: w2977 -> [_ w2994]
              tunnel: w2964 -> [w2991 w2993]
              tunnel: w2963 -> [w2990 w2992]
              frame #0 {
              }
              frame #1 {
                n1540 = VISA Write(VISA resource name=w2993, write buffer=w2994, error in (no error)=w2992) -> (VISA resource name out=w2996:refnum<visa-resource-name>, error out=w2995:errorcluster)  [unwired: 1 out]
              }
            }
            n1541 = case shown="True" w2979 {
              tunnel: [w3005 w3010] -> w2982
              tunnel: [w3004 w3009] -> w2981
              tunnel: w2980 -> [_ w3008]
              tunnel: w2962 -> [w3005 w3007]
              tunnel: w2961 -> [w3004 w3006]
              frame #0 {
              }
              frame #1 {
                n1542 = VISA Write(VISA resource name=w3007, write buffer=w3008, error in (no error)=w3006) -> (VISA resource name out=w3010:refnum<visa-resource-name>, error out=w3009:errorcluster)  [unwired: 1 out]
              }
            }
            n1543 = case shown="True" w2973 {
              tunnel: [w2984 w2989] -> w2972
              tunnel: [w2983 w2988] -> w2971
              tunnel: w2976 -> [_ w2987]
              tunnel: w2960 -> [w2984 w2986]
              tunnel: w2959 -> [w2983 w2985]
              frame #0 {
              }
              frame #1 {
                n1544 = VISA Write(VISA resource name=w2986, write buffer=w2987, error in (no error)=w2985) -> (VISA resource name out=w2989:refnum<visa-resource-name>, error out=w2988:errorcluster)  [unwired: 1 out]
              }
            }
          }
          frame #2 {
            n1545 = Wait (ms)(milliseconds to wait=u32 100) -> ()  [unwired: 1 out]
          }
          frame #3 {
            n1546 = case shown="True" w3036 {
              tunnel: w3038 -> [w3063 w3067]
              tunnel: w3037 -> [w3062 w3066]
              tunnel: [w3063 w3065] -> w3025
              tunnel: [w3062 w3064] -> w3024
              frame #0 {
              }
              frame #1 {
                n1547 = property class="Instr"(reference=w3067, error in=w3066) -> (reference out=w3069:refnum<visa-resource-name>, error out=w3068:errorcluster, "Serial Settings:Number of Bytes at Serial Port"=w3070:u32)
                n1548 = VISA Read(VISA resource name=w3069, byte count=w3070, error in (no error)=w3068) -> (VISA resource name out=w3065:refnum<visa-resource-name>, error out=w3064:errorcluster)  [unwired: 2 out]
              }
            }
            n1549 = case shown="True" w3032 {
              tunnel: w3031 -> [w3045 w3049]
              tunnel: w3030 -> [w3044 w3048]
              tunnel: [w3045 w3047] -> w3029
              tunnel: [w3044 w3046] -> w3028
              frame #0 {
              }
              frame #1 {
                n1550 = property class="Instr"(reference=w3049, error in=w3048) -> (reference out=w3051:refnum<visa-resource-name>, error out=w3050:errorcluster, "Serial Settings:Number of Bytes at Serial Port"=w3052:u32)
                n1551 = VISA Read(VISA resource name=w3051, byte count=w3052, error in (no error)=w3050) -> (VISA resource name out=w3047:refnum<visa-resource-name>, error out=w3046:errorcluster)  [unwired: 2 out]
              }
            }
            n1552 = case shown="True" w3039 {
              tunnel: w3043 -> [w3072 w3076]
              tunnel: w3042 -> [w3071 w3075]
              tunnel: [w3072 w3074] -> w3041
              tunnel: [w3071 w3073] -> w3040
              frame #0 {
              }
              frame #1 {
                n1553 = property class="Instr"(reference=w3076, error in=w3075) -> (reference out=w3078:refnum<visa-resource-name>, error out=w3077:errorcluster, "Serial Settings:Number of Bytes at Serial Port"=w3079:u32)
                n1554 = VISA Read(VISA resource name=w3078, byte count=w3079, error in (no error)=w3077) -> (VISA resource name out=w3074:refnum<visa-resource-name>, error out=w3073:errorcluster)  [unwired: 2 out]
              }
            }
            n1555 = case shown="True" w3035 {
              tunnel: w3034 -> [w3054 w3058]
              tunnel: w3033 -> [w3053 w3057]
              tunnel: [w3054 w3056] -> w3027
              tunnel: [w3053 w3055] -> w3026
              frame #0 {
              }
              frame #1 {
                n1556 = property class="Instr"(reference=w3058, error in=w3057) -> (reference out=w3060:refnum<visa-resource-name>, error out=w3059:errorcluster, "Serial Settings:Number of Bytes at Serial Port"=w3061:u32)
                n1557 = VISA Read(VISA resource name=w3060, byte count=w3061, error in (no error)=w3059) -> (VISA resource name out=w3056:refnum<visa-resource-name>, error out=w3055:errorcluster)  [unwired: 2 out]
              }
            }
          }
          frame #4 {
            n1558 = property on="Y Scan" class="Bool (strict)"("Val(Sgnl)"=FALSE ("Slew Ready 2")) -> ()  [unwired: 2 in, 2 out]
            n1559 = property on="Z Scan" class="Bool (strict)"("Val(Sgnl)"=FALSE ("Slew Ready 2")) -> ()  [unwired: 2 in, 2 out]
            n1560 = property on="X Scan" class="Bool (strict)"("Val(Sgnl)"=FALSE ("Slew Ready 2")) -> ()  [unwired: 2 in, 2 out]
            n1561 = property on="R Scan" class="Bool (strict)"("Val(Sgnl)"=FALSE ("Slew Ready 2")) -> ()  [unwired: 2 in, 2 out]
            n1562 = property on="R Scan Length SP steps" class="DigNum (strict)"("DisabledEnum"=T1."Enabled" ("Disabled")) -> ()  [unwired: 2 in, 2 out]
            n1563 = property on="Y Scan Selocity SP steps/sec" class="DigNum (strict)"("DisabledEnum"=T1."Enabled" ("Disabled")) -> ()  [unwired: 2 in, 2 out]
            n1564 = property on="Scan Go" class="Bool (strict)"("DisabledEnum"=T1."Disabled and Grayed Out" ("Disabled")) -> ()  [unwired: 2 in, 2 out]
            n1565 = property on="Z Scan Velocity SP steps/sec" class="DigNum (strict)"("DisabledEnum"=T1."Enabled" ("Disabled")) -> ()  [unwired: 2 in, 2 out]
            n1566 = property on="X Scan Velocity SP steps/sec" class="DigNum (strict)"("DisabledEnum"=T1."Enabled" ("Disabled")) -> ()  [unwired: 2 in, 2 out]
            n1567 = property on="Y Scan Length SP steps" class="DigNum (strict)"("DisabledEnum"=T1."Enabled" ("Disabled")) -> ()  [unwired: 2 in, 2 out]
            n1568 = property on="R Scan Velocity SP steps/sec" class="DigNum (strict)"("DisabledEnum"=T1."Enabled" ("Disabled")) -> ()  [unwired: 2 in, 2 out]
            n1569 = property on="X Scan Length SP steps" class="DigNum (strict)"("DisabledEnum"=T1."Enabled" ("Disabled")) -> ()  [unwired: 2 in, 2 out]
            n1570 = property on="Z Scan Length SP steps" class="DigNum (strict)"("DisabledEnum"=T1."Enabled" ("Disabled")) -> ()  [unwired: 2 in, 2 out]
          }
        }
        n1571 = local write "STATUS"("SCANNING" ("STATUS")) -> ()
        n1572 = property on="GO" class="Bool"("DisabledEnum"=T1."Disabled and Grayed Out" ("Disabled")) -> ()  [unwired: 2 in, 2 out]
      }
      event #16 {
        n1573 = event-data() -> ()  [unwired: 1 in, 5 out]
        n1574 = property on="GO" class="Bool"("DisabledEnum"=T1."Disabled and Grayed Out" ("Disabled")) -> ()  [unwired: 2 in, 2 out]
        n1575 = flat-sequence {
          tunnel: [w3184] -> w3168
          tunnel: [w3169] -> w3167
          tunnel: [w3183] -> w3166
          tunnel: [w3171] -> w3165
          tunnel: [w3182] -> w3164
          tunnel: [w3172] -> w3163
          tunnel: [w3170] -> w3162
          tunnel: [w3181] -> w3161
          tunnel: w3126 -> [w3180]
          tunnel: w3128 -> [w3179]
          tunnel: w3125 -> [w3178]
          tunnel: w3127 -> [w3177]
          tunnel: w3124 -> [w3176]
          tunnel: w3122 -> [w3175]
          tunnel: w3123 -> [w3174]
          tunnel: w3121 -> [w3173]
          tunnel: [w3180] -> w3160
          tunnel: [w3179] -> w3159
          tunnel: [w3178] -> w3158
          tunnel: [w3177] -> w3157
          tunnel: [w3176] -> w3156
          tunnel: [w3175] -> w3155
          tunnel: [w3174] -> w3154
          tunnel: [w3173] -> w3153
          tunnel: [w3236] -> w3152
          tunnel: [w3235] -> w3151
          tunnel: w3168 -> [w3234]
          tunnel: w3167 -> [w3233]
          tunnel: [w3233] -> w3150
          tunnel: w3166 -> [w3232]
          tunnel: w3165 -> [w3221]
          tunnel: w3164 -> [w3231]
          tunnel: w3163 -> [w3227]
          tunnel: w3162 -> [w3224]
          tunnel: w3161 -> [w3230]
          tunnel: [w3229] -> w3149
          tunnel: [w3228] -> w3148
          tunnel: [w3227] -> w3147
          tunnel: [w3226] -> w3146
          tunnel: [w3225] -> w3145
          tunnel: [w3224] -> w3144
          tunnel: [w3223] -> w3143
          tunnel: [w3222] -> w3142
          tunnel: [w3221] -> w3141
          tunnel: w3160 -> [w3220]
          tunnel: w3159 -> [w3219]
          tunnel: w3158 -> [w3218]
          tunnel: w3157 -> [w3217]
          tunnel: w3156 -> [w3216]
          tunnel: w3155 -> [w3215]
          tunnel: w3154 -> [w3214]
          tunnel: w3153 -> [w3213]
          tunnel: w3152 -> [w3277]
          tunnel: [w3277] -> w3140
          tunnel: w3151 -> [w3276]
          tunnel: [w3276] -> w3139
          tunnel: [w3275] -> w3138
          tunnel: w3150 -> [w3275]
          tunnel: [w3274] -> w3137
          tunnel: w3149 -> [w3274]
          tunnel: [w3273] -> w3136
          tunnel: w3148 -> [w3273]
          tunnel: [w3272] -> w3135
          tunnel: [w3271] -> w3134
          tunnel: w3147 -> [w3271]
          tunnel: [w3270] -> w3133
          tunnel: w3146 -> [w3270]
          tunnel: [w3269] -> w3132
          tunnel: w3145 -> [w3269]
          tunnel: [w3268] -> w3131
          tunnel: w3144 -> [w3268]
          tunnel: [w3267] -> w3130
          tunnel: w3143 -> [w3267]
          tunnel: [w3266] -> w3129
          tunnel: w3142 -> [w3266]
          tunnel: w3141 -> [w3272]
          tunnel: w3140 -> [w3297]
          tunnel: w3139 -> [w3296]
          tunnel: w3138 -> [w3293]
          tunnel: w3137 -> [w3292]
          tunnel: w3136 -> [w3291]
          tunnel: w3135 -> [w3290]
          tunnel: w3134 -> [w3289]
          tunnel: w3133 -> [w3288]
          tunnel: w3132 -> [w3287]
          tunnel: w3131 -> [w3286]
          tunnel: w3130 -> [w3285]
          tunnel: w3129 -> [w3284]
          tunnel: [w3295] -> w3110
          tunnel: [w3294] -> w3109
          tunnel: [w3283] -> w3108
          tunnel: [w3282] -> w3107
          tunnel: [w3281] -> w3106
          tunnel: [w3280] -> w3105
          tunnel: [w3279] -> w3104
          tunnel: [w3278] -> w3103
          tunnel: [w3336] -> w3119
          tunnel: [w3337] -> w3120
          tunnel: [w3338] -> w3113
          tunnel: [w3339] -> w3114
          tunnel: [w3340] -> w3117
          tunnel: [w3341] -> w3118
          tunnel: [w3342] -> w3115
          tunnel: [w3343] -> w3116
          tunnel: w3110 -> [w3343]
          tunnel: w3109 -> [w3342]
          tunnel: w3108 -> [w3341]
          tunnel: w3107 -> [w3340]
          tunnel: w3106 -> [w3339]
          tunnel: w3105 -> [w3338]
          tunnel: w3104 -> [w3337]
          tunnel: w3103 -> [w3336]
          frame #0 {
            n1576 = property on="Z Scan" class="Bool (strict)"() -> ("Value"=w3170:bool)  [unwired: 2 in, 2 out]
            n1577 = property on="X Scan" class="Bool (strict)"() -> ("Value"=w3171:bool)  [unwired: 2 in, 2 out]
            n1578 = property on="R Scan" class="Bool (strict)"() -> ("Value"=w3172:bool)  [unwired: 2 in, 2 out]
            n1579 = property on="Y Scan" class="Bool (strict)"() -> ("Value"=w3169:bool)  [unwired: 2 in, 2 out]
            n1580 = case shown="True" w3169 {
              tunnel: ["" w3208] -> w3184
              frame #0 {
              }
              frame #1 {
                n1581 = property on="Y Scan Length SP steps" class="DigNum (strict)"() -> ("Value"=w3207:i32)  [unwired: 2 in, 2 out]
                n1582 = Number To Decimal String(number=w3207) -> (decimal integer string=w3210:string)  [unwired: 1 in]
                n1583 = call <vilib>:"Space Constant.vi"() -> ("String"=w3211:string)
                n1584 = Concatenate Strings("MR", w3211, w3210, "\r") -> (w3208:string)
              }
            }
            n1585 = case shown="True" w3171 {
              tunnel: ["" w3201] -> w3183
              frame #0 {
              }
              frame #1 {
                n1586 = property on="X Scan Length SP steps" class="DigNum (strict)"() -> ("Value"=w3200:i32)  [unwired: 2 in, 2 out]
                n1587 = Number To Decimal String(number=w3200) -> (decimal integer string=w3203:string)  [unwired: 1 in]
                n1588 = call <vilib>:"Space Constant.vi"() -> ("String"=w3204:string)
                n1589 = Concatenate Strings("MR", w3204, w3203, "\r") -> (w3201:string)
              }
            }
            n1590 = case shown="True" w3172 {
              tunnel: ["" w3187] -> w3181
              frame #0 {
              }
              frame #1 {
                n1591 = property on="R Scan Length SP steps" class="DigNum (strict)"() -> ("Value"=w3186:i32)  [unwired: 2 in, 2 out]
                n1592 = Number To Decimal String(number=w3186) -> (decimal integer string=w3189:string)  [unwired: 1 in]
                n1593 = call <vilib>:"Space Constant.vi"() -> ("String"=w3190:string)
                n1594 = Concatenate Strings("MR", w3190, w3189, "\r") -> (w3187:string)
              }
            }
            n1595 = case shown="True" w3170 {
              tunnel: ["" w3194] -> w3182
              frame #0 {
              }
              frame #1 {
                n1596 = property on="Z Scan Length SP steps" class="DigNum (strict)"() -> ("Value"=w3193:i32)  [unwired: 2 in, 2 out]
                n1597 = Number To Decimal String(number=w3193) -> (decimal integer string=w3196:string)  [unwired: 1 in]
                n1598 = call <vilib>:"Space Constant.vi"() -> ("String"=w3197:string)
                n1599 = Concatenate Strings("MR", w3197, w3196, "\r") -> (w3194:string)
              }
            }
          }
          frame #1 {
            n1600 = case shown="True" w3221 {
              tunnel: [w3252 w3257] -> w3229
              tunnel: [w3251 w3256] -> w3228
              tunnel: w3232 -> [_ w3255]
              tunnel: w3220 -> [w3252 w3254]
              tunnel: w3219 -> [w3251 w3253]
              frame #0 {
              }
              frame #1 {
                n1601 = VISA Write(VISA resource name=w3254, write buffer=w3255, error in (no error)=w3253) -> (VISA resource name out=w3257:refnum<visa-resource-name>, error out=w3256:errorcluster)  [unwired: 1 out]
              }
            }
            n1602 = case shown="True" w3224 {
              tunnel: [w3245 w3250] -> w3223
              tunnel: [w3244 w3249] -> w3222
              tunnel: w3231 -> [_ w3248]
              tunnel: w3218 -> [w3245 w3247]
              tunnel: w3217 -> [w3244 w3246]
              frame #0 {
              }
              frame #1 {
                n1603 = VISA Write(VISA resource name=w3247, write buffer=w3248, error in (no error)=w3246) -> (VISA resource name out=w3250:refnum<visa-resource-name>, error out=w3249:errorcluster)  [unwired: 1 out]
              }
            }
            n1604 = case shown="True" w3233 {
              tunnel: [w3259 w3264] -> w3236
              tunnel: [w3258 w3263] -> w3235
              tunnel: w3234 -> [_ w3262]
              tunnel: w3216 -> [w3259 w3261]
              tunnel: w3215 -> [w3258 w3260]
              frame #0 {
              }
              frame #1 {
                n1605 = VISA Write(VISA resource name=w3261, write buffer=w3262, error in (no error)=w3260) -> (VISA resource name out=w3264:refnum<visa-resource-name>, error out=w3263:errorcluster)  [unwired: 1 out]
              }
            }
            n1606 = case shown="True" w3227 {
              tunnel: [w3238 w3243] -> w3226
              tunnel: [w3237 w3242] -> w3225
              tunnel: w3230 -> [_ w3241]
              tunnel: w3214 -> [w3238 w3240]
              tunnel: w3213 -> [w3237 w3239]
              frame #0 {
              }
              frame #1 {
                n1607 = VISA Write(VISA resource name=w3240, write buffer=w3241, error in (no error)=w3239) -> (VISA resource name out=w3243:refnum<visa-resource-name>, error out=w3242:errorcluster)  [unwired: 1 out]
              }
            }
          }
          frame #2 {
            n1608 = Wait (ms)(milliseconds to wait=u32 100) -> ()  [unwired: 1 out]
          }
          frame #3 {
            n1609 = case shown="True" w3290 {
              tunnel: w3292 -> [w3317 w3321]
              tunnel: w3291 -> [w3316 w3320]
              tunnel: [w3317 w3319] -> w3279
              tunnel: [w3316 w3318] -> w3278
              frame #0 {
              }
              frame #1 {
                n1610 = property class="Instr"(reference=w3321, error in=w3320) -> (reference out=w3323:refnum<visa-resource-name>, error out=w3322:errorcluster, "Serial Settings:Number of Bytes at Serial Port"=w3324:u32)
                n1611 = VISA Read(VISA resource name=w3323, byte count=w3324, error in (no error)=w3322) -> (VISA resource name out=w3319:refnum<visa-resource-name>, error out=w3318:errorcluster)  [unwired: 2 out]
              }
            }
            n1612 = case shown="True" w3286 {
              tunnel: w3285 -> [w3299 w3303]
              tunnel: w3284 -> [w3298 w3302]
              tunnel: [w3299 w3301] -> w3283
              tunnel: [w3298 w3300] -> w3282
              frame #0 {
              }
              frame #1 {
                n1613 = property class="Instr"(reference=w3303, error in=w3302) -> (reference out=w3305:refnum<visa-resource-name>, error out=w3304:errorcluster, "Serial Settings:Number of Bytes at Serial Port"=w3306:u32)
                n1614 = VISA Read(VISA resource name=w3305, byte count=w3306, error in (no error)=w3304) -> (VISA resource name out=w3301:refnum<visa-resource-name>, error out=w3300:errorcluster)  [unwired: 2 out]
              }
            }
            n1615 = case shown="True" w3293 {
              tunnel: w3297 -> [w3326 w3330]
              tunnel: w3296 -> [w3325 w3329]
              tunnel: [w3326 w3328] -> w3295
              tunnel: [w3325 w3327] -> w3294
              frame #0 {
              }
              frame #1 {
                n1616 = property class="Instr"(reference=w3330, error in=w3329) -> (reference out=w3332:refnum<visa-resource-name>, error out=w3331:errorcluster, "Serial Settings:Number of Bytes at Serial Port"=w3333:u32)
                n1617 = VISA Read(VISA resource name=w3332, byte count=w3333, error in (no error)=w3331) -> (VISA resource name out=w3328:refnum<visa-resource-name>, error out=w3327:errorcluster)  [unwired: 2 out]
              }
            }
            n1618 = case shown="True" w3289 {
              tunnel: w3288 -> [w3308 w3312]
              tunnel: w3287 -> [w3307 w3311]
              tunnel: [w3308 w3310] -> w3281
              tunnel: [w3307 w3309] -> w3280
              frame #0 {
              }
              frame #1 {
                n1619 = property class="Instr"(reference=w3312, error in=w3311) -> (reference out=w3314:refnum<visa-resource-name>, error out=w3313:errorcluster, "Serial Settings:Number of Bytes at Serial Port"=w3315:u32)
                n1620 = VISA Read(VISA resource name=w3314, byte count=w3315, error in (no error)=w3313) -> (VISA resource name out=w3310:refnum<visa-resource-name>, error out=w3309:errorcluster)  [unwired: 2 out]
              }
            }
          }
          frame #4 {
            w3334 = FALSE ("Value (Signaling)")
            n1621 = Wait (ms)(milliseconds to wait=u32 75) -> ()  [unwired: 1 out]
            n1622 = property on="Y Scan" class="Bool (strict)"("Val(Sgnl)"=w3334) -> ()  [unwired: 2 in, 2 out]
            n1623 = property on="X Scan" class="Bool (strict)"("Val(Sgnl)"=w3334) -> ()  [unwired: 2 in, 2 out]
            n1624 = property on="Z Scan" class="Bool (strict)"("Val(Sgnl)"=w3334) -> ()  [unwired: 2 in, 2 out]
            n1625 = property on="R Scan" class="Bool (strict)"("Val(Sgnl)"=w3334) -> ()  [unwired: 2 in, 2 out]
          }
        }
        n1626 = property on="FirstScan" class="Bool (strict)"("Val(Sgnl)"=TRUE ("Value (Signaling)")) -> ()  [unwired: 2 in, 2 out]
        n1627 = property on="NewLoop" class="Bool (strict)"("Val(Sgnl)"=FALSE ("Value (Signaling)")) -> ()  [unwired: 2 in, 2 out]
        n1628 = property on="LoopCheck" class="Bool (strict)"("Val(Sgnl)"=FALSE ("Value (Signaling)")) -> ()  [unwired: 2 in, 2 out]
      }
      event #17 {
        n1629 = event-data() -> ()  [unwired: 1 in, 7 out]
        n1630 = flat-sequence {
          tunnel: [w3383] -> w3359
          tunnel: [w3384] -> w3358
          tunnel: w3351 -> [w3382]
          tunnel: w3347 -> [w3381]
          frame #0 {
            n1631 = property on="Reset X Motor Steps" class="DigNum (strict)"() -> ("Value"=w3385:i32)  [unwired: 2 in, 2 out]
            n1632 = Number To Decimal String(number=w3385) -> (decimal integer string=w3386:string)  [unwired: 1 in]
            n1633 = call "mDrive Send Command.vi"("error in (no error)"=w3382, "Extra"=w3386, "Command"=T10."Set Current Position", "VISA resource name"=w3381) -> ("error out"=w3384:errorcluster, "VISA resource name out"=w3383:refnum<visa-resource-name>)  [unwired: 3 in, 1 out]
          }
        }
        n1634 = flat-sequence {
          tunnel: [w3377] -> w3357
          tunnel: [w3378] -> w3356
          tunnel: w3350 -> [w3375]
          tunnel: w3346 -> [w3374]
          frame #0 {
            n1635 = property on="Reset Z Motor Steps" class="DigNum (strict)"() -> ("Value"=w3376:i32)  [unwired: 2 in, 2 out]
            n1636 = Number To Decimal String(number=w3376) -> (decimal integer string=w3379:string)  [unwired: 1 in]
            n1637 = call "mDrive Send Command.vi"("error in (no error)"=w3375, "Extra"=w3379, "Command"=T10."Set Current Position", "VISA resource name"=w3374) -> ("error out"=w3378:errorcluster, "VISA resource name out"=w3377:refnum<visa-resource-name>)  [unwired: 3 in, 1 out]
          }
        }
        n1638 = flat-sequence {
          tunnel: [w3370] -> w3355
          tunnel: [w3371] -> w3354
          tunnel: w3349 -> [w3368]
          tunnel: w3345 -> [w3367]
          frame #0 {
            n1639 = property on="Reset Y Motor Steps" class="DigNum (strict)"() -> ("Value"=w3369:i32)  [unwired: 2 in, 2 out]
            n1640 = Number To Decimal String(number=w3369) -> (decimal integer string=w3372:string)  [unwired: 1 in]
            n1641 = call "mDrive Send Command.vi"("error in (no error)"=w3368, "Extra"=w3372, "Command"=T10."Set Current Position", "VISA resource name"=w3367) -> ("error out"=w3371:errorcluster, "VISA resource name out"=w3370:refnum<visa-resource-name>)  [unwired: 3 in, 1 out]
          }
        }
        n1642 = flat-sequence {
          tunnel: [w3363] -> w3353
          tunnel: [w3364] -> w3352
          tunnel: w3348 -> [w3361]
          tunnel: w3344 -> [w3360]
          frame #0 {
            n1643 = property on="Reset R Motor Steps" class="DigNum (strict)"() -> ("Value"=w3362:i32)  [unwired: 2 in, 2 out]
            n1644 = Number To Decimal String(number=w3362) -> (decimal integer string=w3365:string)  [unwired: 1 in]
            n1645 = call "mDrive Send Command.vi"("error in (no error)"=w3361, "Extra"=w3365, "Command"=T10."Set Current Position", "VISA resource name"=w3360) -> ("error out"=w3364:errorcluster, "VISA resource name out"=w3363:refnum<visa-resource-name>)  [unwired: 3 in, 1 out]
          }
        }
      }
    }
    n1646 = case shown="False" "Set Button" {
      tunnel: "Preset positions" -> [_ w318]
      frame #0 {
      }
      frame #1 {
        n1647 = local read "Presets"() -> (w319:i32[][])
        n1648 = Index Array(array=w319, index (row)=w318) -> (element=w317:i32[])  [unwired: 1 in]
        n1649 = Array To Cluster(array=w317) -> (cluster=w316:T11)
        n1650 = Unbundle(w316) -> ("Presets[0]"=w315:i32, "Presets[1]"=w314:i32, "Presets[2]"=w313:i32, "Presets[3]"=w312:i32)  [unwired: 5 out]
        n1651 = property on="X Step SP" class="DigNum (strict)"("Val(Sgnl)"=w315) -> ()  [unwired: 2 in, 2 out]
        n1652 = property on="Y Step SP" class="DigNum (strict)"("Val(Sgnl)"=w314) -> ()  [unwired: 2 in, 2 out]
        n1653 = property on="Z Step SP" class="DigNum (strict)"("Val(Sgnl)"=w313) -> ()  [unwired: 2 in, 2 out]
        n1654 = property on="R Step SP" class="DigNum (strict)"("Val(Sgnl)"=w312) -> ()  [unwired: 2 in, 2 out]
      }
    }
    n1655 = property on="Preset positions" class="Ring (strict)"() -> ("Strings []"=w263:string[])  [unwired: 2 in, 2 out]
    n1656 = case shown="False" "Add Button" {
      tunnel: w263 -> [_ w311]
      frame #0 {
      }
      frame #1 {
        n1657 = property on="X Step PV" class="DigNum (strict)"() -> ("Value"=w305:i32)  [unwired: 2 in, 2 out]
        n1658 = property on="Y Step PV" class="DigNum (strict)"() -> ("Value"=w304:i32)  [unwired: 2 in, 2 out]
        n1659 = property on="Z Step PV" class="DigNum (strict)"() -> ("Value"=w302:i32)  [unwired: 2 in, 2 out]
        n1660 = property on="R Step PV" class="DigNum (strict)"() -> ("Value"=w303:i32)  [unwired: 2 in, 2 out]
        n1661 = Build Array(w305, w304, w302, w303) -> (w308:i32[])
        n1662 = local read "Presets"() -> (w309:i32[][])
        n1663 = Build Array (concatenate)(w309, w308) -> (w307:i32[][])
        n1664 = Build Array (concatenate)(w311, "String") -> (w306:string[])
        n1665 = local write "Presets"(w307) -> ()
        n1666 = property on="Preset positions" class="Ring (strict)"("Strings []"=w306) -> ()  [unwired: 2 in, 2 out]
      }
    }
    n1667 = case shown="False" "Delete Button" {
      tunnel: w263 -> [_ w301]
      frame #0 {
      }
      frame #1 {
        n1668 = local read "Preset positions"() -> (w299:i32)
        n1669 = local read "Presets"() -> (w300:i32[][])
        n1670 = Delete From Array(array=w301, index=w299) -> (array with subset deleted=w297:string[])  [unwired: 1 in, 1 out]
        n1671 = Delete From Array(array=w300, index (row)=w299) -> (array with subset deleted=w298:i32[][])  [unwired: 2 in, 1 out]
        n1672 = property on="Preset positions" class="Ring (strict)"("Strings []"=w297) -> ()  [unwired: 2 in, 2 out]
        n1673 = local write "Presets"(w298) -> ()
      }
    }
    n1674 = case shown="False" "Stop" {
      selector: "Stop" -> [w328 w370]
      tunnel: [w328 w367] -> w270
      tunnel: w287 -> [w323 w358]
      tunnel: w286 -> [w322 w357]
      tunnel: w285 -> [w321 w359]
      tunnel: w284 -> [w324 w360]
      tunnel: w283 -> [w325 w361]
      tunnel: w282 -> [w326 w362]
      tunnel: w281 -> [w327 w364]
      tunnel: w280 -> [w320 w363]
      tunnel: [w327 w333] -> w279
      tunnel: [w326 w339] -> w278
      tunnel: [w325 w336] -> w277
      tunnel: [w324 w345] -> w276
      tunnel: [w323 w351] -> w275
      tunnel: [w322 w348] -> w274
      tunnel: [w321 w342] -> w273
      tunnel: [w320 w330] -> w272
      tunnel: w269 -> [_ w354]
      tunnel: w268 -> [_ w329]
      frame #0 {
      }
      frame #1 {
        n1675 = flat-sequence {
          tunnel: w370 -> [w436]
          tunnel: [w436] -> w369
          tunnel: [w435] -> w365
          tunnel: w364 -> [w429]
          tunnel: w363 -> [w428]
          tunnel: w362 -> [w427]
          tunnel: w361 -> [w426]
          tunnel: w360 -> [w425]
          tunnel: w359 -> [w422]
          tunnel: w358 -> [w424]
          tunnel: w357 -> [w423]
          tunnel: [w434] -> w355
          tunnel: w354 -> [w434]
          tunnel: [w381] -> w352
          tunnel: [w380] -> w349
          tunnel: [w390] -> w346
          tunnel: [w389] -> w343
          tunnel: [w400] -> w340
          tunnel: [w398] -> w337
          tunnel: [w409] -> w334
          tunnel: [w407] -> w331
          tunnel: w329 -> [w417]
          tunnel: w369 -> [w448]
          tunnel: [w448] -> w368
          tunnel: [w437] -> w366
          tunnel: w365 -> [w447]
          tunnel: [w446] -> w356
          tunnel: w355 -> [w446]
          tunnel: [w445] -> w353
          tunnel: w352 -> [w445]
          tunnel: [w444] -> w350
          tunnel: w349 -> [w444]
          tunnel: [w443] -> w347
          tunnel: w346 -> [w443]
          tunnel: [w442] -> w344
          tunnel: w343 -> [w442]
          tunnel: [w441] -> w341
          tunnel: w340 -> [w441]
          tunnel: [w440] -> w338
          tunnel: w337 -> [w440]
          tunnel: [w439] -> w335
          tunnel: w334 -> [w439]
          tunnel: [w438] -> w332
          tunnel: w331 -> [w438]
          tunnel: w368 -> [w460]
          tunnel: [w460] -> w367
          tunnel: w366 -> [w450]
          tunnel: w356 -> [w459]
          tunnel: w353 -> [w458]
          tunnel: [w458] -> w351
          tunnel: w350 -> [w457]
          tunnel: [w457] -> w348
          tunnel: w347 -> [w456]
          tunnel: [w456] -> w345
          tunnel: [w455] -> w342
          tunnel: w344 -> [w455]
          tunnel: [w454] -> w339
          tunnel: w341 -> [w454]
          tunnel: [w453] -> w336
          tunnel: w338 -> [w453]
          tunnel: [w452] -> w333
          tunnel: w335 -> [w452]
          tunnel: [w451] -> w330
          tunnel: w332 -> [w451]
          frame #0 {
            n1676 = local read "Presets"() -> (w416:i32[][])
            n1677 = call "mDrive Send Command.vi"("error in (no error)"=w428, "Command"=T10."Stop", "VISA resource name"=w429) -> ("error out"=w408:errorcluster, "VISA resource name out"=w410:refnum<visa-resource-name>)  [unwired: 4 in, 1 out]
            n1678 = call "mDrive Send Command.vi"("error in (no error)"=w426, "Command"=T10."Stop", "VISA resource name"=w427) -> ("error out"=w399:errorcluster, "VISA resource name out"=w401:refnum<visa-resource-name>)  [unwired: 4 in, 1 out]
            n1679 = call "mDrive Send Command.vi"("error in (no error)"=w422, "Command"=T10."Stop", "VISA resource name"=w425) -> ("error out"=w391:errorcluster, "VISA resource name out"=w392:refnum<visa-resource-name>)  [unwired: 4 in, 1 out]
            n1680 = call "mDrive Send Command.vi"("error in (no error)"=w423, "Command"=T10."Stop", "VISA resource name"=w424) -> ("error out"=w382:errorcluster, "VISA resource name out"=w383:refnum<visa-resource-name>)  [unwired: 4 in, 1 out]
            n1681 = property on="Preset positions" class="Ring (strict)"() -> ("Strings []"=w415:string[])  [unwired: 2 in, 2 out]
            n1682 = Number To Fractional String(number=w416) -> (F-format string=w418:string[][])  [unwired: 3 in]
            n1683 = property on="X  in Range" class="Bool (strict)"("Val(Sgnl)"=FALSE ("Value (Signaling)")) -> ()  [unwired: 2 in, 2 out]
            n1684 = property on="Y in Range" class="Bool (strict)"("Val(Sgnl)"=FALSE ("Value (Signaling)")) -> ()  [unwired: 2 in, 2 out]
            n1685 = property on="Z in Range" class="Bool (strict)"("Val(Sgnl)"=FALSE ("Value (Signaling)")) -> ()  [unwired: 2 in, 2 out]
            n1686 = property on="R in Range" class="Bool (strict)"("Val(Sgnl)"=FALSE ("Value (Signaling)")) -> ()  [unwired: 2 in, 2 out]
            n1687 = property on="X Ready" class="Bool (strict)"("Val(Sgnl)"=FALSE ("Value (Signaling)")) -> ()  [unwired: 2 in, 2 out]
            n1688 = property on="Y Ready" class="Bool (strict)"("Val(Sgnl)"=FALSE ("Value (Signaling)")) -> ()  [unwired: 2 in, 2 out]
            n1689 = property on="Z Ready" class="Bool (strict)"("Val(Sgnl)"=FALSE ("Value (Signaling)")) -> ()  [unwired: 2 in, 2 out]
            n1690 = property on="R Ready" class="Bool (strict)"("Val(Sgnl)"=FALSE ("Value (Signaling)")) -> ()  [unwired: 2 in, 2 out]
            n1691 = Transpose 2D Array(2D array=w418) -> (transposed array=w419:string[][])
            n1692 = Build Array (concatenate)(w415, w419) -> (w420:string[][])
            n1693 = call "mDrive Send Command.vi"("error in (no error)"=w399, "Extra"="P", "Command"=T10."Print Parameter", "VISA resource name"=w401) -> ("error out"=w398:errorcluster, "read buffer"=w405:string, "VISA resource name out"=w400:refnum<visa-resource-name>)  [unwired: 3 in]
            n1694 = call "mDrive Send Command.vi"("error in (no error)"=w391, "Extra"="P", "Command"=T10."Print Parameter", "VISA resource name"=w392) -> ("error out"=w389:errorcluster, "read buffer"=w396:string, "VISA resource name out"=w390:refnum<visa-resource-name>)  [unwired: 3 in]
            n1695 = call "mDrive Send Command.vi"("error in (no error)"=w408, "Extra"="P", "Command"=T10."Print Parameter", "VISA resource name"=w410) -> ("error out"=w407:errorcluster, "read buffer"=w414:string, "VISA resource name out"=w409:refnum<visa-resource-name>)  [unwired: 3 in]
            n1696 = call "mDrive Send Command.vi"("error in (no error)"=w382, "Extra"="P", "Command"=T10."Print Parameter", "VISA resource name"=w383) -> ("error out"=w380:errorcluster, "read buffer"=w387:string, "VISA resource name out"=w381:refnum<visa-resource-name>)  [unwired: 3 in]
            n1697 = Transpose 2D Array(2D array=w420) -> (transposed array=w421:string[][])
            n1698 = Decimal String To Number(string=w405, offset=0) -> (number=w397:i32)  [unwired: 1 in, 1 out]
            n1699 = Decimal String To Number(string=w396, offset=0) -> (number=w388:i32)  [unwired: 1 in, 1 out]
            n1700 = Decimal String To Number(string=w414, offset=0) -> (number=w406:i32)  [unwired: 1 in, 1 out]
            n1701 = Decimal String To Number(string=w387, offset=0) -> (number=w379:i32)  [unwired: 1 in, 1 out]
            n1702 = call-poly <vilib>:"Write To Spreadsheet File.vi"("2D data"=w421, "file path (dialog if empty)"=w417) -> ()  [unwired: 6 in, 1 out]
            n1703 = Build Array(w406, w388, w397, w379) -> (w435:i32[])
          }
          frame #1 {
            n1704 = To Double Precision Float(number=w447) -> (double precision float=w437:dbl[])
            n1705 = Wait (ms)(milliseconds to wait=u32 20) -> ()  [unwired: 1 out]
          }
          frame #2 {
            n1706 = call-poly <vilib>:"Write To Spreadsheet File.vi"("1D data"=w450, "file path (dialog if empty)"=w459) -> ()  [unwired: 6 in, 1 out]
          }
        }
      }
    }
  }
  n1707 = property on="LoopCheck" class="Bool (strict)"("Val(Sgnl)"=w3) -> ()  [unwired: 2 in, 2 out]
  n1708 = property on="Z Moved" class="Bool (strict)"("Val(Sgnl)"=w3) -> ()  [unwired: 2 in, 2 out]
  n1709 = property on="NewLoop" class="Bool (strict)"("Val(Sgnl)"=FALSE ("Value (Signaling)")) -> ()  [unwired: 2 in, 2 out]
  n1710 = property on="LoopScanConfirmed" class="Bool (strict)"("Val(Sgnl)"=FALSE ("Value (Signaling)")) -> ()  [unwired: 2 in, 2 out]
  n1711 = flat-sequence {
    tunnel: w52 -> [w3392]
    tunnel: w51 -> [w3389]
    frame #0 {
      n1712 = call "mDrive Send Command.vi"("error in (no error)"=w3389, "Command"=T10."Stop", "VISA resource name"=w3392) -> ("error out"=w3390:errorcluster, "VISA resource name out"=w3391:refnum<visa-resource-name>)  [unwired: 4 in, 1 out]
      n1713 = VISA Close(VISA resource name=w3391, error in (no error)=w3390) -> ()  [unwired: 1 out]
    }
  }
  n1714 = flat-sequence {
    tunnel: w46 -> [w3397]
    tunnel: w45 -> [w3394]
    frame #0 {
      n1715 = call "mDrive Send Command.vi"("error in (no error)"=w3394, "Command"=T10."Stop", "VISA resource name"=w3397) -> ("error out"=w3395:errorcluster, "VISA resource name out"=w3396:refnum<visa-resource-name>)  [unwired: 4 in, 1 out]
      n1716 = VISA Close(VISA resource name=w3396, error in (no error)=w3395) -> ()  [unwired: 1 out]
    }
  }
  n1717 = flat-sequence {
    tunnel: w44 -> [w3402]
    tunnel: w43 -> [w3399]
    frame #0 {
      n1718 = call "mDrive Send Command.vi"("error in (no error)"=w3399, "Command"=T10."Stop", "VISA resource name"=w3402) -> ("error out"=w3400:errorcluster, "VISA resource name out"=w3401:refnum<visa-resource-name>)  [unwired: 4 in, 1 out]
      n1719 = VISA Close(VISA resource name=w3401, error in (no error)=w3400) -> ()  [unwired: 1 out]
    }
  }
  n1720 = flat-sequence {
    tunnel: w42 -> [w3407]
    tunnel: w41 -> [w3404]
    frame #0 {
      n1721 = call "mDrive Send Command.vi"("error in (no error)"=w3404, "Command"=T10."Stop", "VISA resource name"=w3407) -> ("error out"=w3405:errorcluster, "VISA resource name out"=w3406:refnum<visa-resource-name>)  [unwired: 4 in, 1 out]
      n1722 = VISA Close(VISA resource name=w3406, error in (no error)=w3405) -> ()  [unwired: 1 out]
    }
  }
  "YCONSTArray" <- w40
  "XCONSTArray" <- w39
  "RCONSTArray" <- w38
  "ZCONSTArray" <- w37
  "RUNHOLDArray" <- w36
